vi "StreamEye_host_v6_32bit.vi"() -> ()   [LabVIEW 2018]
uses:
  CryoSubVIs/SubVIs/JS_Comm.llb/Comm_Paras.ctl
  CryoSubVIs/SubVIs/JS_Comm.llb/Comm_Method.ctl
  CryoSubVIs/SMC SubVIs/SMC_SubVIs.llb/SMC Paras.ctl
  CryoSubVIs/SMC SubVIs/SMC_SubVIs.llb/VENUSNr.ctl
  <vilib>/DAQmx/write.llb/DAQmx Write (Analog DBL 1Chan 1Samp).vi
  CryoSubVIs/SMC SubVIs/SMC_SubVIs.llb/glb_stop.vi
  CryoSubVIs/SMC SubVIs/SMC_SubVIs.llb/glb_pos.vi
  <vilib>/DAQmx/miscellaneous.llb/DAQmx Fill In Error Info.vi
  <vilib>/Utility/file.llb/Write Delimited Spreadsheet (I64).vi
  <vilib>/Utility/file.llb/Write Delimited Spreadsheet (DBL).vi
  <vilib>/DAQmx/create/channels.llb/DAQmx Create Channel (AO-Voltage-Basic).vi
  PicoHarpLibrary/ttrmode32_custom.llb/Global.vi
  PicoHarpLibrary/PHLib.dll
panel:
  in  "Start Sync":bool
  in  "Drift Comp BackStep":dbl caption="BackStep (µm)" min=-10000.0 max=10000.0 step=0.001
  in  "Compensate Int Time":dbl=1000.0 caption="Int. Time (s)" min=0.5 max=36000.0 step=0.5 format="%.1f"
  out "FiFo Overrun":bool
  out "T2 Photon Count":i32 caption="Sum Photon Count" format="%0#_6p"
  in  "T2 Segments":u32 caption="Segments (#)" min=1
  in  "Drift Comp Step":dbl caption="Step (µm)" min=-10000.0 max=10000.0 step=0.001
  in  "Drift Comp Range":dbl caption="+/- Range (µm)" min=-10000.0 max=10000.0 step=0.001
  in  "Drift Compensate Time":i32=1000 caption="Drift Period (s)" min=0 max=1000000 step=1
  in  "Start T2 Collect":bool
  out "TTTR ON":bool
  in  "Enable T2":bool
  in  "Compensate":bool
  in  "Acc. Threshold (cts)":i64=1000 min=-1000000000 max=1000000000 step=1
  in  "Integration Number (#)":i32=1000 min=1 max=36000 step=1
  in  "SyncOffset (ps)":i32=1000 min=0 max=1000000 step=1
  out "Histo Graph":cluster{"Array":dbl[], u32[]}(graph)
  in  "Start Histogram":bool
  in  "Start Cursors Pair XY Sca":bool
  in  "Wait Scan.":bool
  in  "G-asym":dbl
  out "Res. (ps)":i32 min=0 max=2000 step=1
  in  "Histo Time (s)":dbl=1000.0 min=0.5 max=36000.0 step=0.5 format="%.1f"
  out "PicoHarp error":bool
  in  "Signal source selection":T1(radio)
  in  "Binning":i32 min=0 max=7 step=1
  in  "Sync div":enum16{"1", "2", "4", "8"}(ring)
  in  "Apply PicoHarp Settings":bool
  in  "Ch1 Level (mV)":i32=50 min=0 max=800 step=10
  in  "Ch1 ZeroX (mV)":i32=10 min=0 max=20 step=1
  in  "Ch0 ZeroX (mV)":i32=10 min=0 max=20 step=1
  in  "Ch0 Level (mV)":i32=50 min=0 max=800 step=10
  in  "Init Picoharp":bool
  out "PicoHarp ON":bool
  out "Ch1 Rate":dbl caption="Ch1" format="%#_3p"
  out "Ch0 Rate":dbl caption="Ch0" format="%#_3p"
  in  "Start Cursor XY Sca":bool
  in  "G-Scalling (µm/V)":dbl
  in  "Filaname":string
  in  "Path":path
  out "time elapsed dummy":dbl caption="int."
  in  "Intensity mode selection":T2(radio)
  out "time elapsed":dbl caption="Time per step (s)"
  out "XYZ MegaArray Sca":i32[][][](array[numeric])
  out "Data available XW":bool
  in  "Save Data XW":bool
  in  "Save Data Gal":bool
  in  "Save Data Sca":bool
  out "Data available Sca":bool
  out "Data available Gal":bool
  in  "Steps Hyperspectral Sca":u32 caption="Steps Hyperspectral (#)"
  in  "Steps Hyperspectral Gal":u32 caption="Steps Hyperspectral (#)"
  out "busy":bool
  in  "Start Stream":bool
  in  "Misc Info/Variables":T3(tab)
  out "Yscale Gal":dbl[](array[numeric]) format="%.2f"
  out "Wscale Gal":dbl[](array[numeric]) format="%.2f"
  out "Wscale Sca":dbl[](array[numeric]) format="%.2f"
  out "XYZ MegaArray Gal":i32[][][](array[numeric])
  out "XW MegaArray":i32[][](array[numeric])
  out "Xscale hyper":dbl[](array[numeric]) format="%.2f"
  out "Yscale hyper":dbl[](array[numeric]) format="%.2f"
  out "Wscale hyper":dbl[](array[numeric]) format="%.2f"
  out "XY Array Sca":i32[][](array[numeric])
  out "XY Array Gal":i32[][](array[numeric])
  out "Xscale Sca":dbl[](array[numeric]) format="%.2f"
  out "Yscale Sca":dbl[](array[numeric]) format="%.2f"
  out "Xscale Gal":dbl[](array[numeric]) format="%.2f"
  out "Scanner error out":errorcluster
  out "Galvo error out X":errorcluster
  out "Galvo task out X":refnum<k21>
  out "Galvo error out Y":errorcluster
  out "Galvo task out Y":refnum<k21>
  in  "numPixels":u16
  out "time start":i32 caption="Time per step (s)"
  out "single spectrum?":bool
  out "error reader":errorcluster
  out "error writer":errorcluster
  out "writer endpoint":refnum<k21>
  out "reader endpoint":refnum<k21>
  in  "T2 Block Size":u16(ring) items=["Min"=1, "Small"=2, "Mid"=3, "Large"=4, "Max"=5]
  in  "Test Comp histo":bool
  in  "Autosave Histograms":bool
  out "PicoHarp handle":i32
  out "DLL Version (must be 3.0)":string caption="DLL Version"
  out "Initialization Status":string
  out "Calibration Status":string
  out "file error status":errorcluster
  in  "Start Cursors Pair XY Gal":bool
  in  "Start image Sca":bool
  in  "Start Hyperspectral Sca":bool
  in  "Start image Gal":bool
  in  "Start Hyperspectral Gal":bool
  in  "Start Cursor XY Gal":bool
  in  "Yoffset_Sca":dbl min=-10000.0 max=10000.0 step=0.001
  in  "Xoffset_Sca":dbl min=-10000.0 max=10000.0 step=0.001
  out "Xsteps_Sca":u32
  out "Ysteps_Sca":u32 caption="yRead"
  in  "Ydelay_Sca":dbl=0.001 min=0.0 max=300000.0 step=0.001
  in  "Ystep_Sca":dbl=0.001 min=0.001 max=200.0 step=0.001
  in  "Xstep_Sca":dbl=0.001 min=-1000.0 max=1000.0 step=0.001
  in  "Xdelay_Sca":dbl=0.1 min=0.0 max=360000.0 step=0.001
  in  "Yend_Sca":dbl min=-10000.0 max=10000.0 step=0.001
  in  "Ystart_Sca":dbl min=-10000.0 max=10000.0 step=0.001
  in  "Xend_Sca":dbl min=-10000.0 max=10000.0 step=0.001
  in  "Xstart_Sca":dbl min=-10000.0 max=10000.0 step=0.001
  out "Xread_Sca":dbl format="%#.3g"
  out "Yread_Sca":dbl caption="yRead" format="%#.3g"
  in  "Yset_Sca":dbl min=-5000.0 max=5000.0 step=0.001
  in  "Xset_Sca":dbl min=-10000.0 max=10000.0 step=0.001
  in  "Yoffset_Gal":dbl min=-100.0 max=100.0 step=0.001
  in  "Xoffset_Gal":dbl min=-100.0 max=100.0 step=0.001
  out "Xsteps_Gal":u32
  out "Ysteps_Gal":u32 caption="yRead"
  in  "Stop Measurement":bool
  out "Hosts Synchronized":bool
  in  "Synchronize Hosts":bool
  out "XYZ Graph Scanner":i32[][](graph)
  out "XYZ Graph Galvos":i32[][](graph)
  out "XYZ hyperspectral graph":i32[][](graph)
  out "Current Intensity":dbl format="%#_6p"
  out "Time Trace":dbl(graph)
  out "Spectrum Graph":T4(graph)
  in  "Go position Gal":bool
  in  "Ydelay_Gal":dbl=0.001 min=0.0 max=300000.0 step=0.001
  in  "Ystep_Gal":dbl=0.001 min=0.001 max=200.0 step=0.001
  in  "Xstep_Gal":dbl=0.001 min=-1000.0 max=1000.0 step=0.001
  in  "Xdelay_Gal":dbl=0.1 min=0.0 max=360000.0 step=0.001
  in  "Yend_Gal":dbl min=-100.0 max=100.0 step=0.001
  in  "Ystart_Gal":dbl min=-100.0 max=100.0 step=0.001
  in  "Xend_Gal":dbl min=-100.0 max=100.0 step=0.001
  in  "Xstart_Gal":dbl min=-100.0 max=100.0 step=0.001
  out "Xread_Gal":dbl format="%#.3g"
  out "Yread_Gal":dbl caption="yRead" format="%#.3g"
  in  "Yset_Gal":dbl min=-1000.0 max=1000.0 step=0.001
  in  "Xset_Gal":dbl min=-1000.0 max=1000.0 step=0.001
  out "Galvos ON":bool
  in  "Init Galvos":bool
  in  "Go position Sca":bool
  out "Scanner ON":bool
  in  "Init Scanner":bool
  in  "Exit":bool
  # "Signal Source"
  # "Stream Mode"
  # "Scanner"
  # "Galvos"
  # "X-axis"
  # "X-axis"
  # "Y-axis"
  # "Y-axis"
  # "Offset (µm)"
  # "Set (µm)"
  # "Readout"
  # "Start (µm)"
  # "End (µm)"
  # "Step (µm)"
  # "Intensity"
  # "Steps (#)"
  # "Delay (s)"
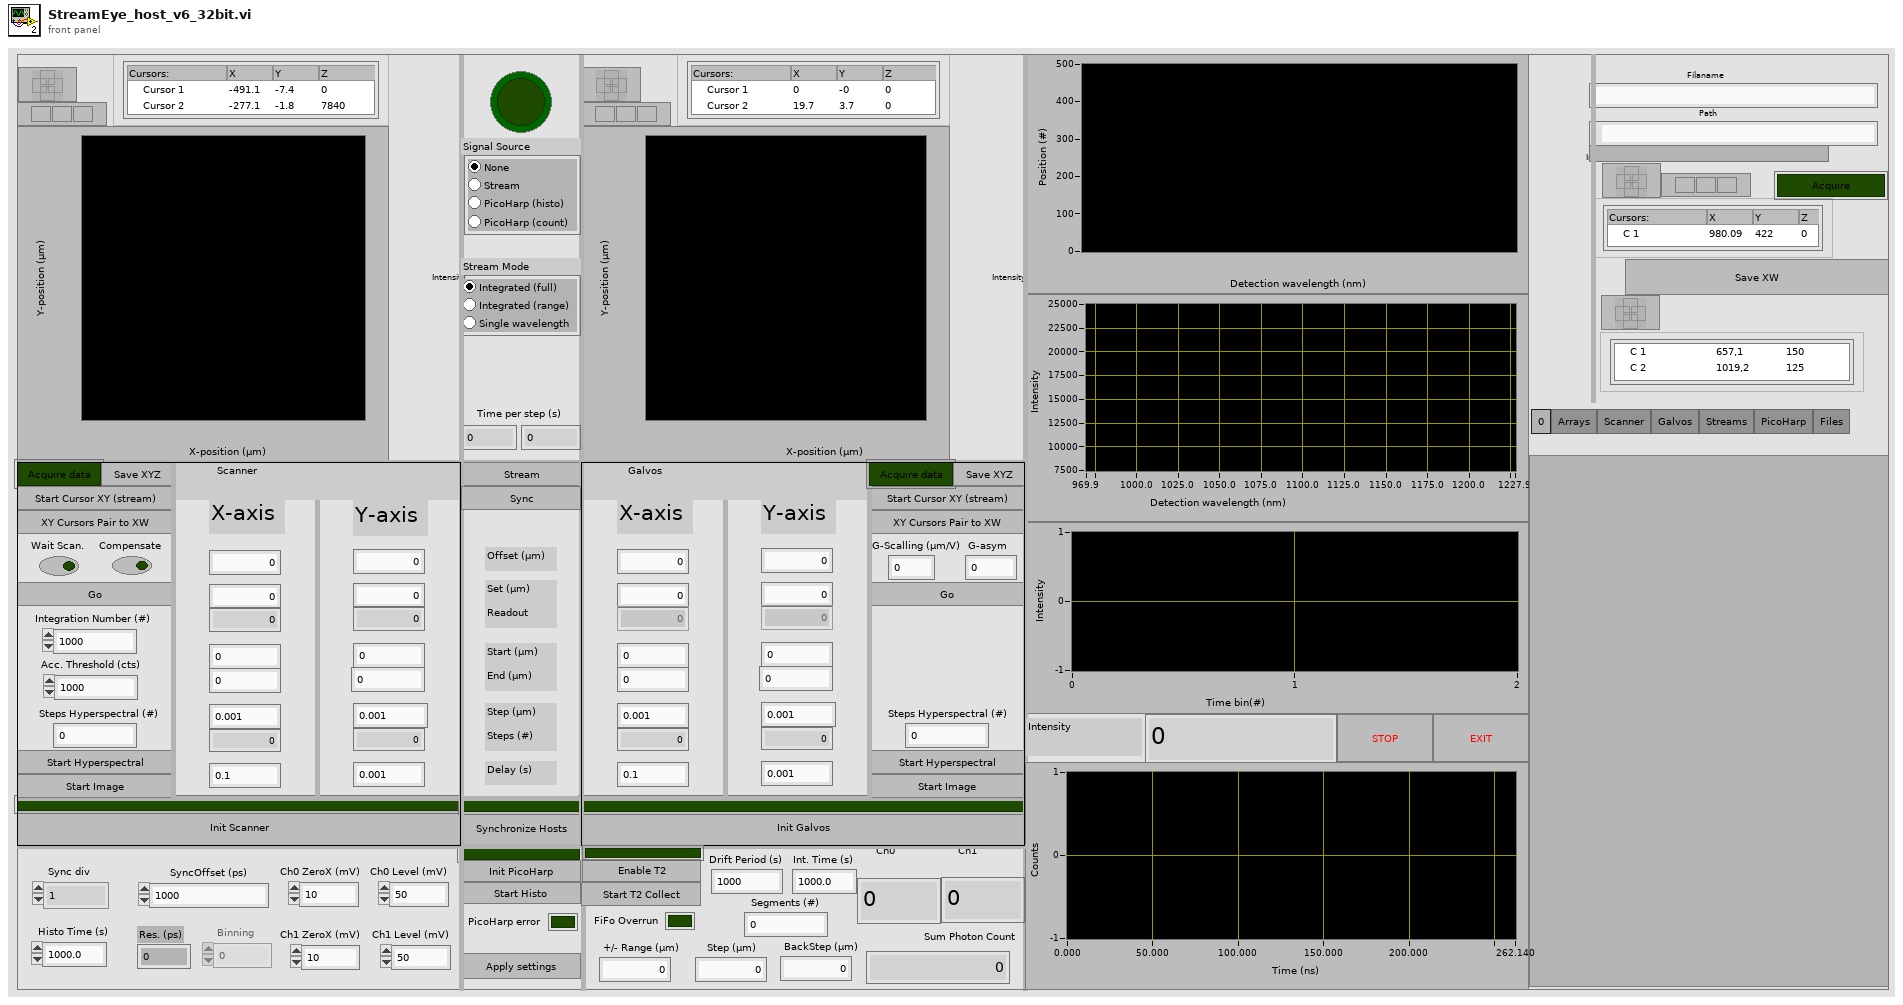
[diagram p1: front panel]
types:
  T1 = enum32{"Signal None", "Signal Stream", "Signal PicoHarp histro", "Signal PicoHarp count rate"}
  T2 = enum32{"Integrated (full)", "Integrated (range)", "Single wavelength"}
  T3 = enum32{"0", "Arrays", "Scanner", "Galvos", "Streams", "PicoHarp", "Files"}
  T4 = cluster{"Calibrated Array":dbl[], "Array F32":sgl[]}
  T5 = enum16{"big-endian, network order", "native, host order", "little-endian"}
  T6 = enum16{"open", "replace", "create", "open or create", "replace or create", "replace or create with confirmation"}
  T7 = typedef "SMC Paras.ctl" = cluster{"VENUS Language":T8, "Number of Axis":u8, "Controller Nr":u8, "Simulation":bool}
  T8 = typedef "VENUSNr.ctl" = enum16{"VENUS 2", "VENUS 1"}
  T9 = typedef "Comm_Paras.ctl" = cluster{"Comm Method":T10, "Com Port":i32, "Baud Rate":u32, "IP Address":string, "Remote Port":u16, "GPIB Address":string, "VISA Resource Name":refnum<visa-resource-name>, "Visa Baud Rate":u32, "Visa Serial":bool}
  T10 = typedef "Comm_Method.ctl" = enum16{"RS232", "TCPIP", "GPIB", "VISA"}
  T11 = typedef "LVCursorListTypeDef.ctl" = cluster{"Name":string, "Color":u32, "Style":u8, "Point Style":u8, "Name Visible":bool, "Allow Drag":bool, "Cursor Mode":u32, "Plot":i32, "Index":i32, "Position":cluster{"X":dbl, "Y":dbl}, "X Scale":u32, "Y Scale":u32, "Watch Plots":i32[], "Watch All Plots":bool, "Plot Area":i32, "Label Offset":cluster{"X":dbl, "Y":dbl}}[]
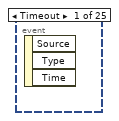
[diagram p2: hidden frame]
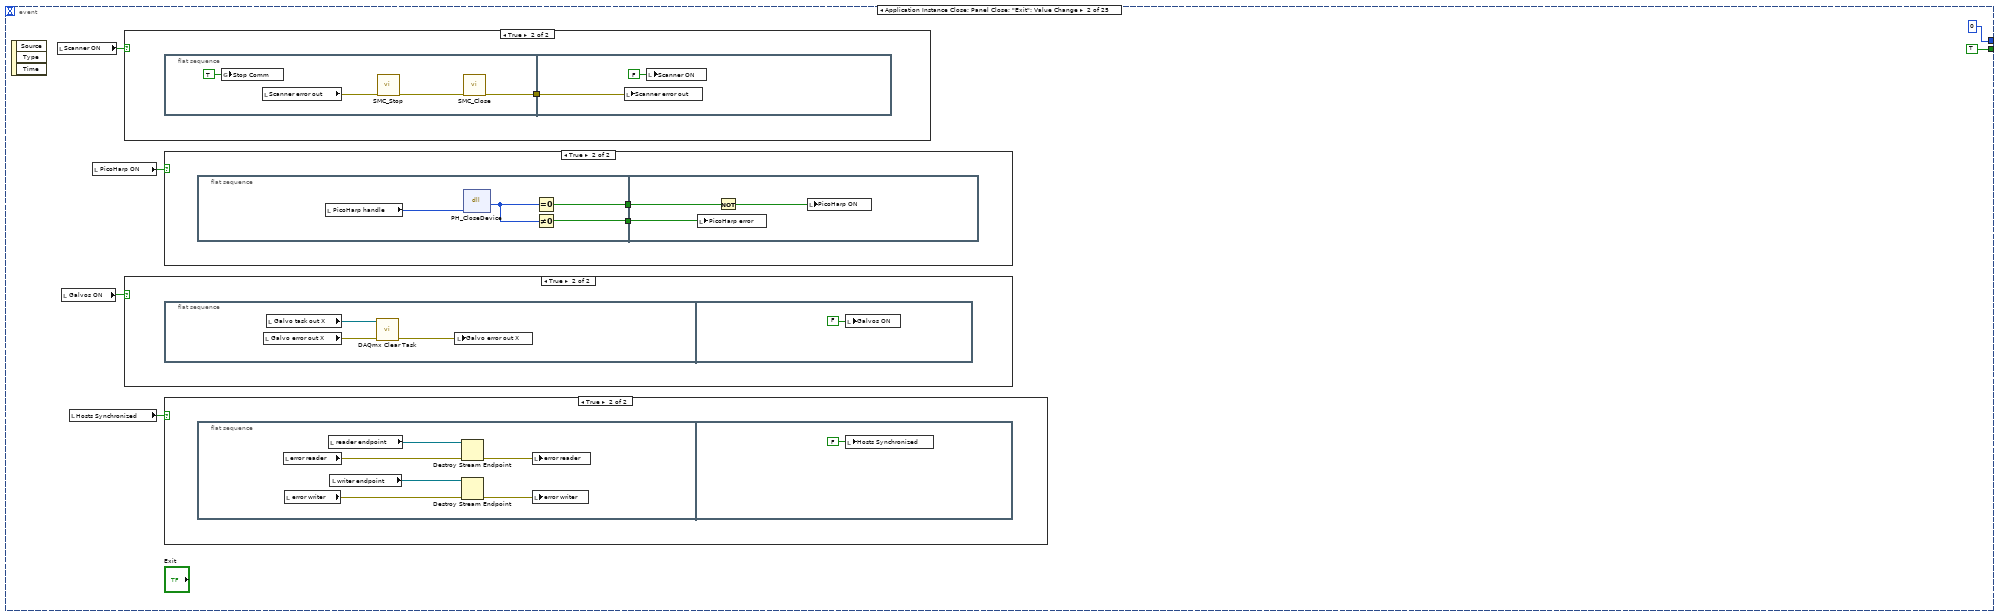
[diagram p3: hidden frame]
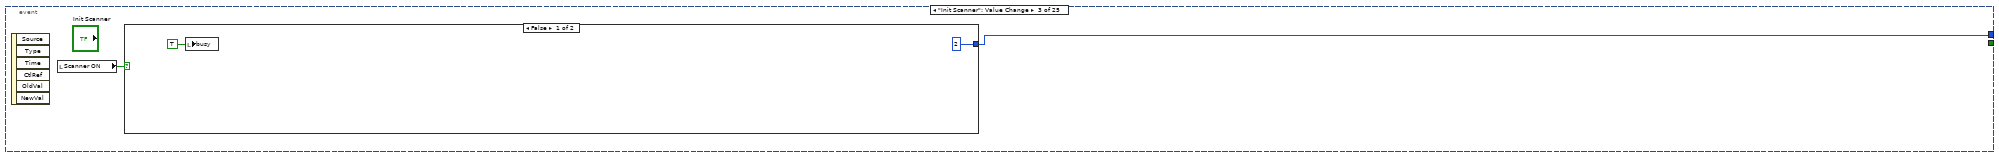
[diagram p8: hidden frame]
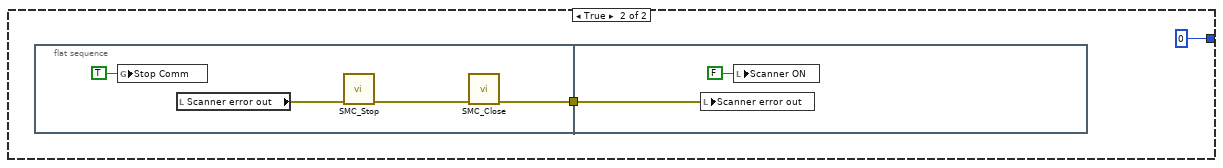
[diagram p9: hidden frame]
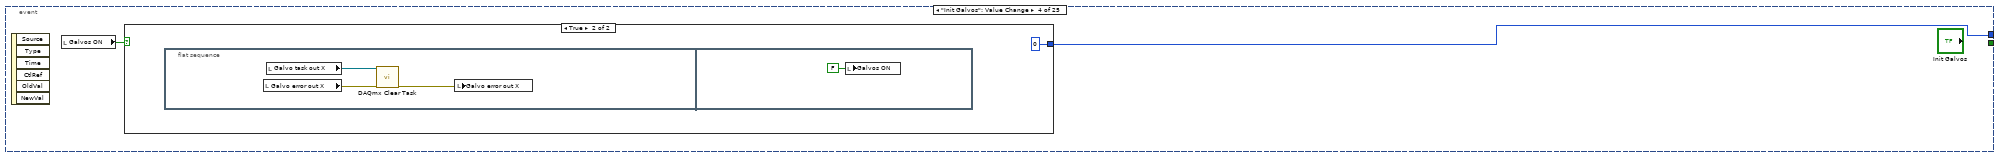
[diagram p10: hidden frame]
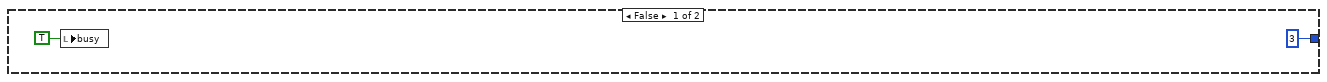
[diagram p11: hidden frame]
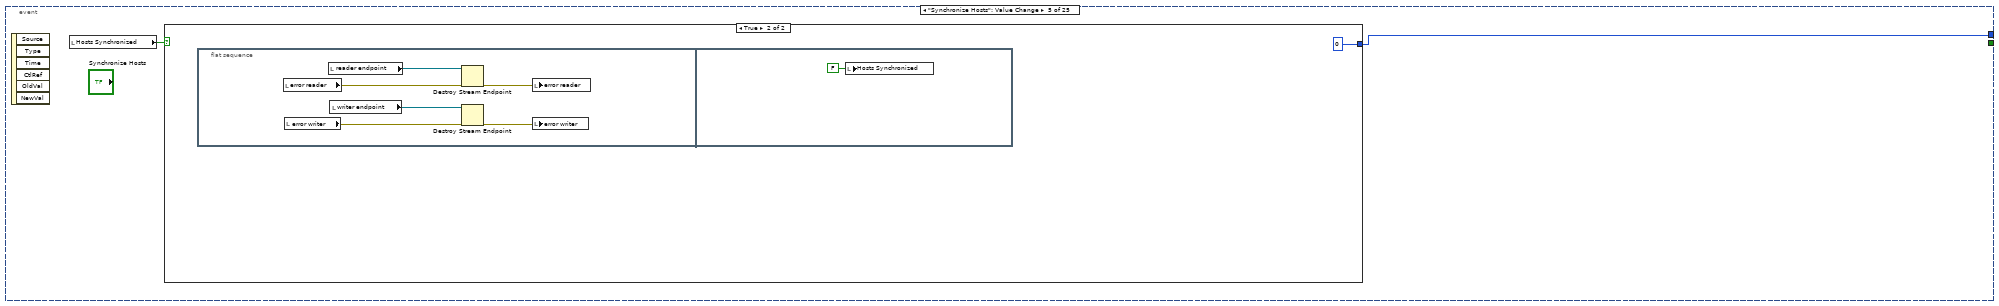
[diagram p12: hidden frame]
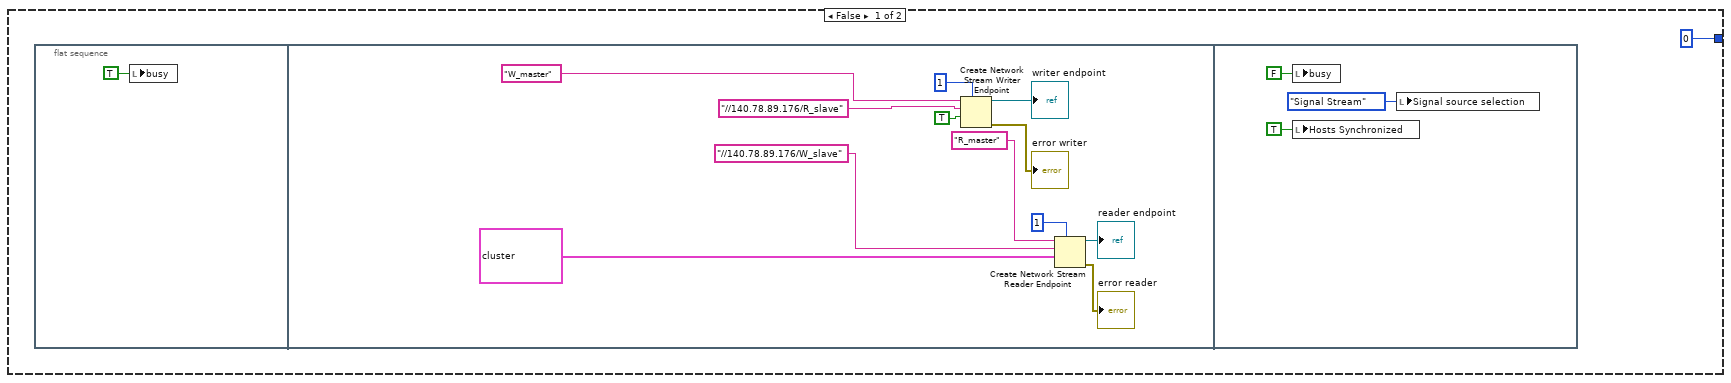
[diagram p13: hidden frame]
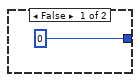
[diagram p14: hidden frame]
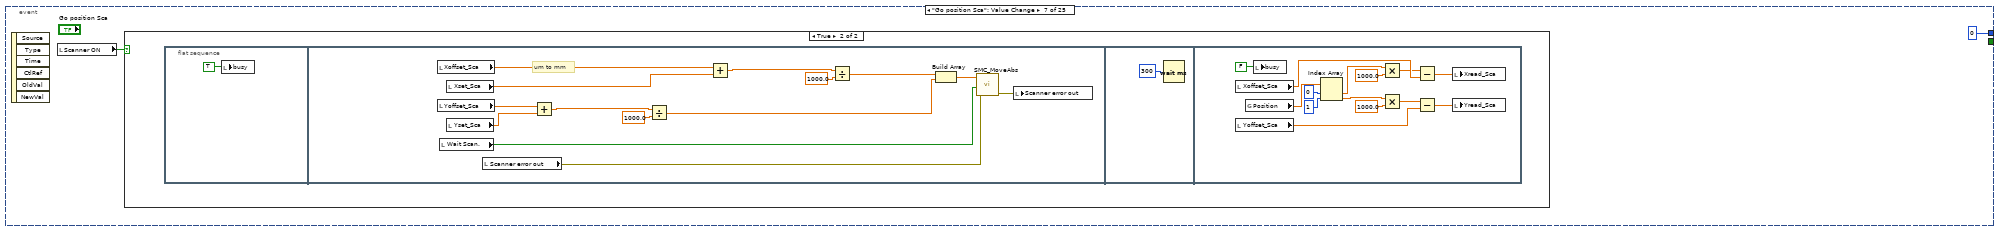
[diagram p15: hidden frame]
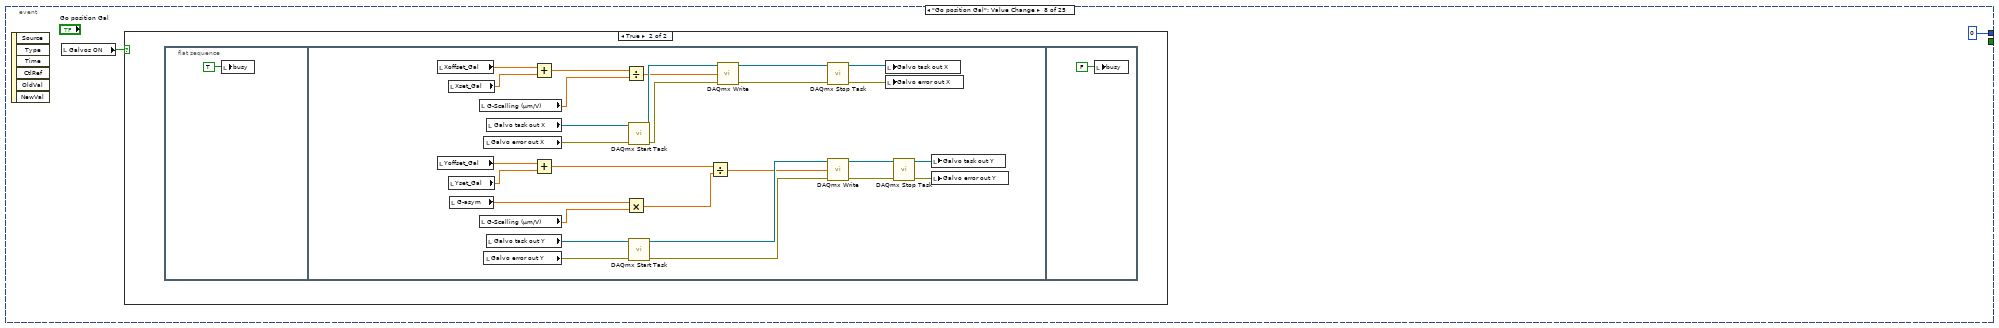
[diagram p17: hidden frame]
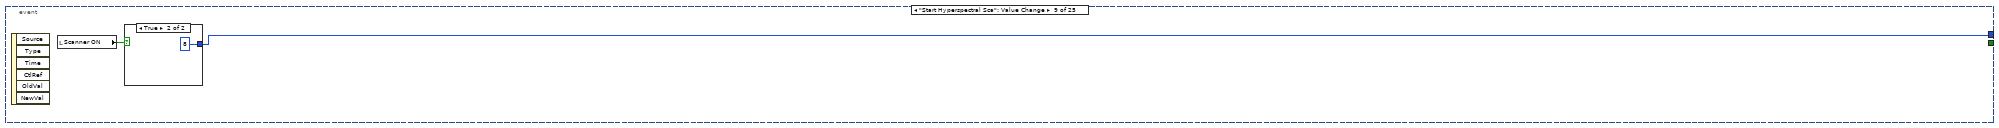
[diagram p19: hidden frame]
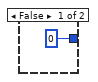
[diagram p20: hidden frame]
diagram:
  n1 = flat-sequence {
    frame #0 {
      w1 = u16 3 items=["Min"=1, "Small"=2, "Mid"=3, "Large"=4, "Max"=5] ("T2 Block Size")
      w22 = 1 ("dimension size")
      w21 = 1 ("dimension size")
      w19 = 1 ("dimension size")
      w20 = 1 ("dimension size")
      w2 = FALSE ("busy")
      n2 = Initialize Array(w22, w22, 1 ("dimension size")) -> (→"XY Array Sca":i32[][])
      n3 = Initialize Array(0, 1 ("dimension size"), 1 ("dimension size")) -> (→"XY Array Gal":i32[][])
      n4 = Initialize Array(w19, w19, 1 ("dimension size")) -> (→"XW MegaArray":i32[][])
      n5 = local write "Binning"(0 ("Range#")) -> ()
      n6 = local write "SyncOffset (ps)"(0 ("SyncOffset (ps)")) -> ()
      n7 = local write "Yoffset_Gal"(0.0 ("Yoffset_Gal")) -> ()
      n8 = local write "Histo Time (s)"(1.0 ("Histro Time (s)")) -> ()
      n9 = local write "Wait Scan."(TRUE ("Wait scanner?")) -> ()
      n10 = local write "Xoffset_Gal"(30.0 ("Xoffset_Gal")) -> ()
      n11 = local write "Ch1 ZeroX (mV)"(10 ("Ch1 ZeroX (mV)")) -> ()
      n12 = local write "G-Scalling (µm/V)"(30.0 ("Galvo Scalling (µm/V)")) -> ()
      n13 = local write "Ch0 ZeroX (mV)"(10 ("Ch0 ZeroX (mV)")) -> ()
      n14 = local write "Ch1 Level (mV)"(200 ("Ch1 Level (mV)")) -> ()
      n15 = local write "Ch0 Level (mV)"(200 ("Ch0 Level (mV)")) -> ()
      n16 = local write "G-asym"(1.45 ("G-asym")) -> ()
      n17 = local write "numPixels"(u16 1024 ("numPixels")) -> ()
      n18 = local write "numPixels"(u16 1024 ("numPixels")) -> ()
      n19 = local write "Sync div"(enum16{"1", "2", "4", "8"}."1" ("Syncdiv")) -> ()
      n20 = local write "T2 Block Size"(w1) -> ()
      n21 = call "subVI_RampGenerator.vi"("Number of Positions"=u16 1, "End  (um)"=10.0, "Start  (um)"=0.0) -> ("Array"=→"Xscale Sca" →"Xscale Gal" →"Yscale Gal" →"Yscale Sca" →"Wscale Gal" →"Wscale Sca" →"Xscale hyper" →"Yscale hyper" →"Wscale hyper":dbl[])  [unwired: 1 in]
      n22 = Initialize Array(w20, w20, 1 ("dimension size"), 1 ("dimension size")) -> (→"XYZ MegaArray Sca":i32[][][])
      n23 = Initialize Array(w21, w21, 1 ("dimension size"), 1 ("dimension size")) -> (→"XYZ MegaArray Gal":i32[][][])
      n24 = local write "Compensate"(w2) -> ()
      n25 = local write "Stop Measurement"(w2) -> ()
      "Scanner ON" <- w2
      "Galvos ON" <- w2
      "Hosts Synchronized" <- w2
      "busy" <- w2
      "Data available Gal" <- w2
      "Data available Sca" <- w2
      "single spectrum?" <- TRUE ("single spectrum?")
      "Data available XW" <- w2
      "PicoHarp ON" <- w2
      "PicoHarp error" <- w2
      "TTTR ON" <- w2
      "T2 Photon Count" <- u32 0 ("T2 Photon Count")
      "FiFo Overrun" <- w2
    }
    frame #1 {
      n26 = while {
        stop <- w42 stop-if-true
        n27 = flat-sequence {
          tunnel: [w45] -> w43
          tunnel: [w44] -> w42
          tunnel: w43 -> [w443]
          frame #0 {
            # "event catcher"
            n28 = event shown="[5] \"Start Stream\": Value Change" {
              selector: _ -> [_ _ _ _ _ _ _ _ _ _ _ _ _ _ _ _ _ _ _ _ _ _ _ _ _]
              dyn-events: _ -> [_ _ _ _ _ _ _ _ _ _ _ _ _ _ _ _ _ _ _ _ _ _ _ _ _]
              timeout: 250 -> [_ _ _ _ _ _ _ _ _ _ _ _ _ _ _ _ _ _ _ _ _ _ _ _ _]
              tunnel: [_ 0 w80 w93 w101 w133 0 0 w201 w205 w209 w213 w217 w221 _ _ _ w313 w318 _ w369 w372 w379 w383 w440] -> w45
              tunnel: [_ TRUE _ _ _ _ _ _ _ _ _ _ _ _ _ _ _ _ _ _ _ _ _ _ _] -> w44
              event Timeout {
                n29 = event-data() -> ()  [unwired: 1 in, 3 out]
              }
              event Application Instance Close; Panel Close; "Exit": Value Change {
                n30 = event-data() -> ()  [unwired: 1 in, 3 out]
                n31 = local read "Scanner ON"() -> (w49:bool)
                n32 = local read "Galvos ON"() -> (w48:bool)
                n33 = local read "Hosts Synchronized"() -> (w52:bool)
                n34 = local read "PicoHarp ON"() -> (w47:bool)
                n35 = case shown="True" w49 {
                  frame False {
                  }
                  frame True {
                    n36 = flat-sequence {
                      tunnel: [w70] -> w66
                      tunnel: w66 -> [w71]
                      frame #0 {
                        n37 = global write "glb_stop.vi" "Stop Comm"(TRUE ("Stop Comm")) -> ()
                        n38 = local read "Scanner error out"() -> (w67:errorcluster)
                        n39 = call "SMC_Stop.vi"("error in (no error)"=w67) -> ("error out"=w68:errorcluster)  [unwired: 10 in]
                        n40 = call "SMC_Close.vi"("error in (no error)"=w68) -> ("error out"=w70:errorcluster)  [unwired: 10 in]
                      }
                      frame #1 {
                        n41 = local write "Scanner error out"(w71) -> ()
                        n42 = local write "Scanner ON"(FALSE ("Scanner ON")) -> ()
                      }
                    }
                  }
                }
                n43 = case shown="True" w48 {
                  frame False {
                  }
                  frame True {
                    n44 = flat-sequence {
                      frame #0 {
                        n45 = local read "Galvo error out X"() -> (w63:errorcluster)
                        n46 = local read "Galvo task out X"() -> (w64:refnum<k21>)
                        n47 = call <vilib>:"DAQmx Clear Task.vi"("task in"=w64, "error in"=w63) -> ("error out"=w62:errorcluster)  [unwired: 13 in]
                        n48 = local write "Galvo error out X"(w62) -> ()
                      }
                      frame #1 {
                        n49 = local write "Galvos ON"(FALSE ("Galvos ON")) -> ()
                      }
                    }
                  }
                }
                n50 = case shown="True" w47 {
                  frame False {
                  }
                  frame True {
                    n51 = flat-sequence {
                      tunnel: [w56] -> w54
                      tunnel: [w55] -> w53
                      tunnel: w54 -> [w61]
                      tunnel: w53 -> [w59]
                      frame #0 {
                        n52 = local read "PicoHarp handle"() -> (w58:i32)
                        n53 = dll-call lib="F:/Users/Yuriy/Labview/JKU/StreamEye/StreamEye_master_v2_comp2015/PicoHarpLibrary/PHLib.dll" fn="PH_CloseDevice"("devidx"=w58) -> ("return type"=w57:i32)  [unwired: 4 in, 2 out]
                        n54 = Equal To 0?(x=w57) -> (x = 0?=w56:bool)
                        n55 = Not Equal To 0?(x=w57) -> (x != 0?=w55:bool)
                      }
                      frame #1 {
                        n56 = local write "PicoHarp error"(w59) -> ()
                        n57 = Not(x=w61) -> (.not. x?=w60:bool)
                        n58 = local write "PicoHarp ON"(w60) -> ()
                      }
                    }
                  }
                }
                n59 = case shown="True" w52 {
                  frame False {
                  }
                  frame True {
                    n60 = flat-sequence {
                      frame #0 {
                        n61 = local read "error reader"() -> (w78:errorcluster)
                        n62 = local read "error writer"() -> (w75:errorcluster)
                        n63 = local read "reader endpoint"() -> (w73:refnum<k21>)
                        n64 = local read "writer endpoint"() -> (w74:refnum<k21>)
                        n65 = Destroy Stream Endpoint(8:w78, 11:w73) -> (0:w77:errorcluster)
                        n66 = Destroy Stream Endpoint(8:w75, 11:w74) -> (0:w76:errorcluster)
                        n67 = local write "error reader"(w77) -> ()
                        n68 = local write "error writer"(w76) -> ()
                      }
                      frame #1 {
                        n69 = local write "Hosts Synchronized"(FALSE ("Hosts Synchronized")) -> ()
                      }
                    }
                  }
                }
              }
              event "Init Scanner": Value Change {
                n70 = event-data() -> ()  [unwired: 1 in, 6 out]
                n71 = local read "Scanner ON"() -> (w81:bool)
                n72 = case shown="False" w81 {
                  tunnel: [2 0] -> w80
                  frame False {
                    n73 = local write "busy"(TRUE ("busy")) -> ()
                  }
                  frame True {
                    n74 = flat-sequence {
                      tunnel: [w89] -> w84
                      tunnel: w84 -> [w90]
                      frame #0 {
                        n75 = global write "glb_stop.vi" "Stop Comm"(TRUE ("Stop Comm")) -> ()
                        n76 = local read "Scanner error out"() -> (w86:errorcluster)
                        n77 = call "SMC_Stop.vi"("error in (no error)"=w86) -> ("error out"=w87:errorcluster)  [unwired: 10 in]
                        n78 = call "SMC_Close.vi"("error in (no error)"=w87) -> ("error out"=w89:errorcluster)  [unwired: 10 in]
                      }
                      frame #1 {
                        n79 = local write "Scanner error out"(w90) -> ()
                        n80 = local write "Scanner ON"(FALSE ("Scanner ON")) -> ()
                      }
                    }
                  }
                }
              }
              event "Init Galvos": Value Change {
                n81 = event-data() -> ()  [unwired: 1 in, 6 out]
                n82 = local read "Galvos ON"() -> (w92:bool)
                n83 = case shown="True" w92 {
                  tunnel: [3 0] -> w93
                  frame False {
                    n84 = local write "busy"(TRUE ("busy")) -> ()
                  }
                  frame True {
                    n85 = flat-sequence {
                      frame #0 {
                        n86 = local read "Galvo error out X"() -> (w98:errorcluster)
                        n87 = local read "Galvo task out X"() -> (w99:refnum<k21>)
                        n88 = call <vilib>:"DAQmx Clear Task.vi"("task in"=w99, "error in"=w98) -> ("error out"=w97:errorcluster)  [unwired: 13 in]
                        n89 = local write "Galvo error out X"(w97) -> ()
                      }
                      frame #1 {
                        n90 = local write "Galvos ON"(FALSE ("Galvos ON")) -> ()
                      }
                    }
                  }
                }
              }
              event "Synchronize Hosts": Value Change {
                n91 = event-data() -> ()  [unwired: 1 in, 6 out]
                n92 = local read "Hosts Synchronized"() -> (w102:bool)
                n93 = case shown="True" w102 {
                  tunnel: [0 0] -> w101
                  frame False {
                    n94 = flat-sequence {
                      frame #0 {
                        n95 = local write "busy"(TRUE ("busy")) -> ()
                      }
                      frame #1 {
                        n96 = Create Network Stream Writer Endpoint(7:1 ("writer buffer size"), 9:TRUE, 10:"//140.78.89.176/R_slave" ("writer url"), 11:"W_master" ("reader name")) -> (0:→"error writer":errorcluster, 3:→"writer endpoint":refnum<k21>)  [unwired: 3 in]
                        n97 = Create Network Stream Reader Endpoint(7:1 ("reader buffer size"), 9:cluster{dbl[], dbl[]} {array[512 elements], array[512 elements]} ("XY Graph OMA V"), 10:"//140.78.89.176/W_slave" ("writer url"), 11:"R_master" ("reader name")) -> (0:→"error reader":errorcluster, 3:→"reader endpoint":refnum<k21>)  [unwired: 3 in]
                      }
                      frame #2 {
                        n98 = local write "busy"(FALSE ("busy")) -> ()
                        n99 = local write "Hosts Synchronized"(TRUE ("Hosts Synchronized")) -> ()
                        n100 = local write "Signal source selection"(T1."Signal Stream" ("Signal source selection")) -> ()
                      }
                    }
                  }
                  frame True {
                    n101 = flat-sequence {
                      frame #0 {
                        n102 = local read "error reader"() -> (w126:errorcluster)
                        n103 = local read "error writer"() -> (w123:errorcluster)
                        n104 = local read "reader endpoint"() -> (w121:refnum<k21>)
                        n105 = local read "writer endpoint"() -> (w122:refnum<k21>)
                        n106 = Destroy Stream Endpoint(8:w126, 11:w121) -> (0:w125:errorcluster)
                        n107 = Destroy Stream Endpoint(8:w123, 11:w122) -> (0:w124:errorcluster)
                        n108 = local write "error reader"(w125) -> ()
                        n109 = local write "error writer"(w124) -> ()
                      }
                      frame #1 {
                        n110 = local write "Hosts Synchronized"(FALSE ("Hosts Synchronized")) -> ()
                      }
                    }
                  }
                }
              }
              event "Start Stream": Value Change {
                n111 = event-data() -> ()  [unwired: 1 in, 6 out]
                n112 = local read "Hosts Synchronized"() -> (w131:bool)
                n113 = local read "Signal source selection"() -> (w130:T1)
                n114 = Equal?(x=w130, y=T1."Signal Stream" ("Signal source selection")) -> (x = y?=w128:bool)
                n115 = And(x=w131, y=w128) -> (x .and. y?=w132:bool)
                n116 = case shown="True" w132 {
                  tunnel: [0 5] -> w133
                  frame False {
                  }
                  frame True {
                  }
                }
              }
              event "Go position Sca": Value Change {
                n117 = event-data() -> ()  [unwired: 1 in, 6 out]
                n118 = local read "Scanner ON"() -> (w136:bool)
                n119 = case shown="True" w136 {
                  frame False {
                  }
                  frame True {
                    n120 = flat-sequence {
                      frame #0 {
                        n121 = local write "busy"(TRUE ("busy")) -> ()
                      }
                      frame #1 {
                        # "um to mm"
                        n122 = local read "Xoffset_Sca"() -> (w145:dbl)
                        n123 = local read "Yoffset_Sca"() -> (w147:dbl)
                        n124 = local read "Wait Scan."() -> (w139:bool)
                        n125 = local read "Xset_Sca"() -> (w144:dbl)
                        n126 = local read "Yset_Sca"() -> (w146:dbl)
                        n127 = local read "Scanner error out"() -> (w152:errorcluster)
                        n128 = Add(x=w147, y=w146) -> (x+y=w149:dbl)
                        n129 = Divide(x=w149, y=1000.0) -> (x/y=w142:dbl)
                        n130 = Add(x=w145, y=w144) -> (x+y=w151:dbl)
                        n131 = Divide(x=w151, y=1000.0) -> (x/y=w143:dbl)
                        n132 = Build Array(w143, w142) -> (w141:dbl[])
                        n133 = call "SMC_MoveAbs.vi"("error in (no error)"=w152, "WaitUntilReady"=w139, "Input Array"=w141) -> ("error out"=w140:errorcluster)  [unwired: 8 in]
                        n134 = local write "Scanner error out"(w140) -> ()
                      }
                      frame #2 {
                        n135 = Wait (ms)(milliseconds to wait=u32 300) -> ()  [unwired: 1 out]
                      }
                      frame #3 {
                        n136 = local read "Xoffset_Sca"() -> (w160:dbl)
                        n137 = local read "Yoffset_Sca"() -> (w163:dbl)
                        n138 = global read "glb_pos.vi" "Position"() -> (w158:dbl[])
                        n139 = local write "busy"(FALSE ("busy")) -> ()
                        n140 = Index Array(array=w158, index #1=0 ("index"), index #2=1 ("index")) -> (element #1=w162:dbl, element #2=w166:dbl)
                        n141 = Multiply(x=w162, y=1000.0) -> (x*y=w159:dbl)
                        n142 = Multiply(x=w166, y=1000.0) -> (x*y=w164:dbl)
                        n143 = Subtract(x=w159, y=w160) -> (x-y=w161:dbl)
                        n144 = Subtract(x=w164, y=w163) -> (x-y=w165:dbl)
                        n145 = local write "Xread_Sca"(w161) -> ()
                        n146 = local write "Yread_Sca"(w165) -> ()
                      }
                    }
                  }
                }
              }
              event "Go position Gal": Value Change {
                n147 = event-data() -> ()  [unwired: 1 in, 6 out]
                n148 = local read "Galvos ON"() -> (w168:bool)
                n149 = case shown="True" w168 {
                  frame False {
                  }
                  frame True {
                    n150 = flat-sequence {
                      frame #0 {
                        n151 = local write "busy"(TRUE ("busy")) -> ()
                      }
                      frame #1 {
                        n152 = local read "Xoffset_Gal"() -> (w198:dbl)
                        n153 = local read "Yoffset_Gal"() -> (w196:dbl)
                        n154 = local read "Xset_Gal"() -> (w197:dbl)
                        n155 = local read "Yset_Gal"() -> (w195:dbl)
                        n156 = local read "G-asym"() -> (w173:dbl)
                        n157 = local read "G-Scalling (µm/V)"() -> (w177:dbl)
                        n158 = local read "G-Scalling (µm/V)"() -> (w172:dbl)
                        n159 = local read "Galvo error out X"() -> (w187:errorcluster)
                        n160 = local read "Galvo error out Y"() -> (w179:errorcluster)
                        n161 = local read "Galvo task out X"() -> (w188:refnum<k21>)
                        n162 = local read "Galvo task out Y"() -> (w180:refnum<k21>)
                        n163 = Add(x=w198, y=w197) -> (x+y=w178:dbl)
                        n164 = Add(x=w196, y=w195) -> (x+y=w175:dbl)
                        n165 = Divide(x=w178, y=w177) -> (x/y=w176:dbl)
                        n166 = Multiply(x=w173, y=w172) -> (x*y=w171:dbl)
                        n167 = call <vilib>:"DAQmx Start Task.vi"("task/channels in"=w188, "error in"=w187) -> ("task out"=w192:refnum<k21>, "error out"=w189:errorcluster)  [unwired: 12 in]
                        n168 = call <vilib>:"DAQmx Start Task.vi"("task/channels in"=w180, "error in"=w179) -> ("task out"=w184:refnum<k21>, "error out"=w181:errorcluster)  [unwired: 12 in]
                        n169 = Divide(x=w175, y=w171) -> (x/y=w174:dbl)
                        n170 = call-poly <vilib>:"DAQmx Write.vi"("task/channels in"=w192, "data"=w176, "error in"=w189) -> ("task out"=w191:refnum<k21>, "error out"=w190:errorcluster)  [unwired: 10 in, 1 out]
                        n171 = call <vilib>:"DAQmx Stop Task.vi"("task/channels in"=w191, "error in"=w190) -> ("task out"=w193:refnum<k21>, "error out"=w194:errorcluster)  [unwired: 12 in]
                        n172 = call-poly <vilib>:"DAQmx Write.vi"("task/channels in"=w184, "data"=w174, "error in"=w181) -> ("task out"=w183:refnum<k21>, "error out"=w182:errorcluster)  [unwired: 10 in, 1 out]
                        n173 = local write "Galvo task out X"(w193) -> ()
                        n174 = local write "Galvo error out X"(w194) -> ()
                        n175 = call <vilib>:"DAQmx Stop Task.vi"("task/channels in"=w183, "error in"=w182) -> ("task out"=w185:refnum<k21>, "error out"=w186:errorcluster)  [unwired: 12 in]
                        n176 = local write "Galvo task out Y"(w185) -> ()
                        n177 = local write "Galvo error out Y"(w186) -> ()
                      }
                      frame #2 {
                        n178 = local write "busy"(FALSE ("busy")) -> ()
                      }
                    }
                  }
                }
              }
              event "Start Hyperspectral Sca": Value Change {
                n179 = event-data() -> ()  [unwired: 1 in, 6 out]
                n180 = local read "Scanner ON"() -> (w200:bool)
                n181 = case shown="True" w200 {
                  tunnel: [0 8] -> w201
                  frame False {
                  }
                  frame True {
                  }
                }
              }
              event "Start image Sca": Value Change {
                n182 = event-data() -> ()  [unwired: 1 in, 6 out]
                n183 = local read "Scanner ON"() -> (w204:bool)
                n184 = case shown="True" w204 {
                  tunnel: [0 9] -> w205
                  frame False {
                  }
                  frame True {
                  }
                }
              }
              event "Start Hyperspectral Gal": Value Change {
                n185 = event-data() -> ()  [unwired: 1 in, 6 out]
                n186 = local read "Galvos ON"() -> (w208:bool)
                n187 = case shown="True" w208 {
                  tunnel: [0 10] -> w209
                  frame False {
                  }
                  frame True {
                  }
                }
              }
              event "Start image Gal": Value Change {
                n188 = event-data() -> ()  [unwired: 1 in, 6 out]
                n189 = local read "Galvos ON"() -> (w212:bool)
                n190 = case shown="True" w212 {
                  tunnel: [0 11] -> w213
                  frame False {
                  }
                  frame True {
                  }
                }
              }
              event "Start Cursor XY Gal": Value Change {
                n191 = event-data() -> ()  [unwired: 1 in, 6 out]
                n192 = local read "Galvos ON"() -> (w216:bool)
                n193 = case shown="True" w216 {
                  tunnel: [0 12] -> w217
                  frame False {
                  }
                  frame True {
                  }
                }
              }
              event "Start Cursors Pair XY Gal": Value Change {
                n194 = event-data() -> ()  [unwired: 1 in, 6 out]
                n195 = local read "Data available Gal"() -> (w220:bool)
                n196 = case shown="True" w220 {
                  tunnel: [0 13] -> w221
                  frame False {
                  }
                  frame True {
                  }
                }
              }
              event "Save Data Sca": Value Change {
                n197 = event-data() -> ()  [unwired: 1 in, 6 out]
                n198 = local read "Data available Sca"() -> (w224:bool)
                n199 = case shown="True" w224 {
                  frame False {
                  }
                  frame True {
                    w225 = TRUE ("transpose? (F)")
                    # "scales in absolute values (no offset)"
                    n200 = local read "Path"() -> (w231:path)
                    n201 = local read "XY Array Sca"() -> (w244:i32[][])
                    n202 = local read "Wscale Sca"() -> (w255:dbl[])
                    n203 = local read "Yscale Sca"() -> (w256:dbl[])
                    n204 = local read "Xscale Sca"() -> (w257:dbl[])
                    n205 = local read "Filaname"() -> (w237:string)
                    n206 = local read "XYZ MegaArray Sca"() -> (w258:i32[][][])
                    n207 = Concatenate Strings(w237, "XYW_sca.dat") -> (w235:string)
                    n208 = Concatenate Strings(w237, "Wscale_sca.dat") -> (w232:string)
                    n209 = Concatenate Strings(w237, "Yscale_sca.dat") -> (w234:string)
                    n210 = Concatenate Strings(w237, "XY_sca.dat") -> (w236:string)
                    n211 = Concatenate Strings(w237, "Xscale_sca.dat") -> (w233:string)
                    n212 = Build Path(base path=w231, name or relative path=w235) -> (appended path=w226:path)
                    n213 = Build Path(base path=w231, name or relative path=w232) -> (appended path=w228:path)
                    n214 = Build Path(base path=w231, name or relative path=w234) -> (appended path=w230:path)
                    n215 = Build Path(base path=w231, name or relative path=w236) -> (appended path=w227:path)
                    n216 = Build Path(base path=w231, name or relative path=w233) -> (appended path=w229:path)
                    n217 = Open/Create/Replace File(file path (use dialog)=w226, operation (0:open)=T6."replace or create", access (0:read/write)=enum16{"read/write", "read-only", "write-only"}."read/write") -> (refnum out=w254:refnum<file>, error out=w253:errorcluster)  [unwired: 3 in, 1 out]
                    n218 = call-poly <vilib>:"Write Delimited Spreadsheet.vi"("file path (dialog if empty)"=w228, "1D data"=w255, "append to file? (new file:F)"=FALSE, "transpose? (no:F)"=w225) -> ()  [unwired: 10 in, 2 out]
                    n219 = call-poly <vilib>:"Write Delimited Spreadsheet.vi"("file path (dialog if empty)"=w230, "1D data"=w256, "append to file? (new file:F)"=FALSE, "transpose? (no:F)"=w225) -> ()  [unwired: 10 in, 2 out]
                    n220 = call-poly <vilib>:"Write Delimited Spreadsheet.vi"("file path (dialog if empty)"=w227, "2D data"=w244, "append to file? (new file:F)"=FALSE, "transpose? (no:F)"=w225) -> ()  [unwired: 10 in, 2 out]
                    n221 = call-poly <vilib>:"Write Delimited Spreadsheet.vi"("file path (dialog if empty)"=w229, "1D data"=w257, "append to file? (new file:F)"=FALSE, "transpose? (no:F)"=w225) -> ()  [unwired: 10 in, 2 out]
                    n222 = Write to Binary File(file (use dialog)=w254, data=w258, error in=w253, 9:T5."little-endian" ("byte order (0:big-endian, network order)")) -> (refnum out=w252:refnum<file>, error out=w251:errorcluster)  [unwired: 2 in, 1 out]
                    n223 = Close File(refnum=w252, error in=w251) -> ()  [unwired: 2 out]
                  }
                }
              }
              event "Save Data Gal": Value Change {
                n224 = event-data() -> ()  [unwired: 1 in, 6 out]
                n225 = local read "Data available Gal"() -> (w259:bool)
                n226 = case shown="True" w259 {
                  frame False {
                  }
                  frame True {
                    w260 = TRUE ("transpose? (F)")
                    # "scales in absolute values (no offset)"
                    n227 = local read "Path"() -> (w266:path)
                    n228 = local read "XY Array Gal"() -> (w279:i32[][])
                    n229 = local read "Wscale Gal"() -> (w290:dbl[])
                    n230 = local read "Yscale Gal"() -> (w291:dbl[])
                    n231 = local read "Xscale Gal"() -> (w292:dbl[])
                    n232 = local read "Filaname"() -> (w272:string)
                    n233 = local read "XYZ MegaArray Gal"() -> (w293:i32[][][])
                    n234 = Concatenate Strings(w272, "Yscale_gal.dat") -> (w269:string)
                    n235 = Concatenate Strings(w272, "XYW_gal.dat") -> (w270:string)
                    n236 = Concatenate Strings(w272, "Xscale_gal.dat") -> (w268:string)
                    n237 = Concatenate Strings(w272, "Wscale_gal.dat") -> (w267:string)
                    n238 = Concatenate Strings(w272, "XY_gal.dat") -> (w271:string)
                    n239 = Build Path(base path=w266, name or relative path=w270) -> (appended path=w261:path)
                    n240 = Build Path(base path=w266, name or relative path=w268) -> (appended path=w264:path)
                    n241 = Build Path(base path=w266, name or relative path=w267) -> (appended path=w263:path)
                    n242 = Build Path(base path=w266, name or relative path=w271) -> (appended path=w262:path)
                    n243 = Open/Create/Replace File(file path (use dialog)=w261, operation (0:open)=T6."replace or create", access (0:read/write)=enum16{"read/write", "read-only", "write-only"}."read/write") -> (refnum out=w289:refnum<file>, error out=w288:errorcluster)  [unwired: 3 in, 1 out]
                    n244 = call-poly <vilib>:"Write Delimited Spreadsheet.vi"("file path (dialog if empty)"=w264, "1D data"=w292, "append to file? (new file:F)"=FALSE, "transpose? (no:F)"=w260) -> ()  [unwired: 10 in, 2 out]
                    n245 = call-poly <vilib>:"Write Delimited Spreadsheet.vi"("file path (dialog if empty)"=w263, "1D data"=w290, "append to file? (new file:F)"=FALSE, "transpose? (no:F)"=w260) -> ()  [unwired: 10 in, 2 out]
                    n246 = call-poly <vilib>:"Write Delimited Spreadsheet.vi"("file path (dialog if empty)"=w262, "2D data"=w279, "append to file? (new file:F)"=FALSE, "transpose? (no:F)"=w260) -> ()  [unwired: 10 in, 2 out]
                    n247 = Write to Binary File(file (use dialog)=w289, data=w293, error in=w288, 9:T5."little-endian" ("byte order (0:big-endian, network order)")) -> (refnum out=w287:refnum<file>, error out=w286:errorcluster)  [unwired: 2 in, 1 out]
                    n248 = Close File(refnum=w287, error in=w286) -> ()  [unwired: 2 out]
                    n249 = Build Path(base path=w266, name or relative path=w269) -> (appended path=w265:path)
                    n250 = call-poly <vilib>:"Write Delimited Spreadsheet.vi"("file path (dialog if empty)"=w265, "1D data"=w291, "append to file? (new file:F)"=FALSE, "transpose? (no:F)"=w260) -> ()  [unwired: 10 in, 2 out]
                  }
                }
              }
              event "Save Data XW": Value Change {
                n251 = event-data() -> ()  [unwired: 1 in, 6 out]
                n252 = local read "Data available XW"() -> (w294:bool)
                n253 = case shown="True" w294 {
                  frame False {
                  }
                  frame True {
                    w295 = TRUE ("transpose? (F)")
                    # "scales in absolute values (no offset)"
                    n254 = local read "Path"() -> (w299:path)
                    n255 = local read "Xscale hyper"() -> (w312:dbl[])
                    n256 = local read "Filaname"() -> (w303:string)
                    n257 = local read "XW MegaArray"() -> (w308:i32[][])
                    n258 = local read "Wscale hyper"() -> (w311:dbl[])
                    n259 = Concatenate Strings(w303, "XW_hyper.dat") -> (w302:string)
                    n260 = Concatenate Strings(w303, "Xscale_hyper.dat") -> (w301:string)
                    n261 = Build Path(base path=w299, name or relative path=w302) -> (appended path=w296:path)
                    n262 = Concatenate Strings(w303, "Wscale_hyper.dat") -> (w300:string)
                    n263 = Build Path(base path=w299, name or relative path=w300) -> (appended path=w297:path)
                    n264 = call-poly <vilib>:"Write Delimited Spreadsheet.vi"("file path (dialog if empty)"=w296, "2D data"=w308, "append to file? (new file:F)"=FALSE, "transpose? (no:F)"=w295) -> ()  [unwired: 10 in, 2 out]
                    n265 = call-poly <vilib>:"Write Delimited Spreadsheet.vi"("file path (dialog if empty)"=w297, "1D data"=w311, "append to file? (new file:F)"=FALSE, "transpose? (no:F)"=w295) -> ()  [unwired: 10 in, 2 out]
                    n266 = Build Path(base path=w299, name or relative path=w301) -> (appended path=w298:path)
                    n267 = call-poly <vilib>:"Write Delimited Spreadsheet.vi"("file path (dialog if empty)"=w298, "1D data"=w312, "append to file? (new file:F)"=FALSE, "transpose? (no:F)"=w295) -> ()  [unwired: 10 in, 2 out]
                  }
                }
              }
              event "Start Cursor XY Sca": Value Change {
                n268 = event-data() -> ()  [unwired: 1 in, 6 out]
                n269 = local read "Scanner ON"() -> (w314:bool)
                n270 = case shown="True" w314 {
                  tunnel: [0 17] -> w313
                  frame False {
                  }
                  frame True {
                  }
                }
              }
              event "Init Picoharp": Value Change {
                n271 = event-data() -> ()  [unwired: 1 in, 6 out]
                n272 = local read "PicoHarp ON"() -> (w317:bool)
                n273 = case shown="False" w317 {
                  tunnel: [18 0] -> w318
                  frame False {
                    n274 = flat-sequence {
                      tunnel: [w326] -> w319
                      tunnel: w319 -> [w335]
                      frame #0 {
                        n275 = local write "busy"(TRUE ("busy")) -> ()
                      }
                      frame #1 {
                        n276 = call "Initialization.vi"("Mode"=0) -> ("Deviceindex"=w329:i32, "Initialization Status"=w325:string, "DLL Version"=w324:string, "Initialisation Error"=w328:bool)  [unwired: 1 in]
                        n277 = local write "PicoHarp handle"(w329) -> ()
                        n278 = local write "Initialization Status"(w325) -> ()
                        n279 = case shown="False" w328 {
                          selector: w328 -> [_ w333]
                          tunnel: [w332 "Not calibrated"] -> w323
                          tunnel: [w331 w333] -> w327
                          tunnel: w329 -> [w330 _]
                          frame False {
                            n280 = call "Calibrate.vi"("Deviceindex"=w330) -> ("Calib Error"=w331:bool, "Status"=w332:string)  [unwired: 1 in]
                          }
                          frame True {
                          }
                        }
                        n281 = local write "DLL Version (must be 3.0)"(w324) -> ()
                        n282 = local write "Calibration Status"(w323) -> ()
                        n283 = local write "PicoHarp error"(w327) -> ()
                        n284 = Not(x=w327) -> (.not. x?=w326:bool)
                        n285 = local write "PicoHarp ON"(w326) -> ()
                      }
                      frame #2 {
                        n286 = case shown="True" w335 {
                          frame False {
                          }
                          frame True {
                            n287 = local write "Signal source selection"(T1."Signal PicoHarp count rate" ("Signal source selection")) -> ()
                          }
                        }
                        n288 = local write "busy"(FALSE ("busy")) -> ()
                      }
                    }
                  }
                  frame True {
                    n289 = flat-sequence {
                      tunnel: [w342] -> w339
                      tunnel: [w341] -> w338
                      tunnel: w339 -> [w347]
                      tunnel: w338 -> [w345]
                      frame #0 {
                        n290 = local read "PicoHarp handle"() -> (w344:i32)
                        n291 = dll-call lib="F:/Users/Yuriy/Labview/JKU/StreamEye/StreamEye_master_v2_comp2015/PicoHarpLibrary/PHLib.dll" fn="PH_CloseDevice"("devidx"=w344) -> ("return type"=w343:i32)  [unwired: 4 in, 2 out]
                        n292 = Equal To 0?(x=w343) -> (x = 0?=w342:bool)
                        n293 = Not Equal To 0?(x=w343) -> (x != 0?=w341:bool)
                      }
                      frame #1 {
                        n294 = local write "PicoHarp error"(w345) -> ()
                        n295 = Not(x=w347) -> (.not. x?=w346:bool)
                        n296 = local write "PicoHarp ON"(w346) -> ()
                      }
                    }
                  }
                }
              }
              event "Apply PicoHarp Settings": Value Change {
                n297 = event-data() -> ()  [unwired: 1 in, 6 out]
                n298 = local read "PicoHarp ON"() -> (w348:bool)
                n299 = case shown="True" w348 {
                  frame False {
                  }
                  frame True {
                    n300 = flat-sequence {
                      tunnel: [w350] -> w349
                      tunnel: w349 -> [w365]
                      frame #0 {
                        n301 = local read "Sync div"() -> (w354:enum16{"1", "2", "4", "8"})
                        n302 = local read "Binning"() -> (w355:i32)
                        n303 = local read "PicoHarp handle"() -> (w350:i32)
                        n304 = local read "Ch0 ZeroX (mV)"() -> (w358:i32)
                        n305 = local read "Ch1 ZeroX (mV)"() -> (w356:i32)
                        n306 = local read "Ch0 Level (mV)"() -> (w359:i32)
                        n307 = local read "Ch1 Level (mV)"() -> (w357:i32)
                        n308 = Scale By Power Of 2(n=w354, x=1) -> (x*2^n=w360:i32)
                        n309 = call "Settings.vi"("StopOnOverflow"=TRUE, "DeviceIndex"=w350, "Range No."=w355, "SyncDiv"=w360, "CFD1 zero X"=w356, "CFD1 level"=w357, "CFD0 zero X"=w358, "CFD0 level"=w359) -> ("Resolution"=w351:i32, "Error"=w352:bool)  [unwired: 2 in]
                        n310 = local write "PicoHarp error"(w352) -> ()
                        n311 = local write "Res. (ps)"(w351) -> ()
                      }
                      frame #1 {
                        n312 = local read "SyncOffset (ps)"() -> (w364:i32)
                        n313 = dll-call lib="F:/Users/Yuriy/Labview/JKU/StreamEye/StreamEye_master_v2_comp2015/PicoHarpLibrary/phlib.dll" fn="PH_SetOffset"("devidx"=w365, "offset"=w364) -> ("return type"=w363:i32)  [unwired: 5 in, 2 out]
                        n314 = Less Than 0?(x=w363) -> (x < 0?=w362:bool)
                        n315 = local write "PicoHarp error"(w362) -> ()
                      }
                    }
                  }
                }
              }
              event "Start Histogram": Value Change {
                n316 = event-data() -> ()  [unwired: 1 in, 6 out]
                n317 = local read "Test Comp histo"() -> (w368:bool)
                n318 = local read "PicoHarp ON"() -> (w367:bool)
                n319 = Or(x=w367, y=w368) -> (x .or. y?=w366:bool)
                n320 = case shown="True" w366 {
                  tunnel: [0 20] -> w369
                  frame False {
                  }
                  frame True {
                  }
                }
              }
              event "Start Cursors Pair XY Sca": Value Change {
                n321 = event-data() -> ()  [unwired: 1 in, 6 out]
                n322 = local read "Data available Sca"() -> (w373:bool)
                n323 = case shown="True" w373 {
                  tunnel: [0 21] -> w372
                  frame False {
                  }
                  frame True {
                  }
                }
              }
              event "Start T2 Collect": Value Change {
                n324 = event-data() -> ()  [unwired: 1 in, 6 out]
                n325 = local read "PicoHarp ON"() -> (w378:bool)
                n326 = local read "TTTR ON"() -> (w377:bool)
                n327 = And(x=w377, y=w378) -> (x .and. y?=w376:bool)
                n328 = case shown="False" w376 {
                  tunnel: [0 22] -> w379
                  frame False {
                  }
                  frame True {
                  }
                }
              }
              event "Enable T2": Value Change {
                n329 = event-data() -> ()  [unwired: 1 in, 6 out]
                n330 = local read "PicoHarp ON"() -> (w382:bool)
                n331 = case shown="True" w382 {
                  tunnel: [18 0] -> w383
                  frame False {
                    n332 = flat-sequence {
                      tunnel: [w390] -> w384
                      tunnel: w384 -> [w400]
                      frame #0 {
                        n333 = local write "busy"(TRUE ("busy")) -> ()
                      }
                      frame #1 {
                        n334 = call "Initialization.vi"("Mode"=2) -> ("Deviceindex"=w394:i32, "Initialization Status"=w389:string, "DLL Version"=w388:string, "Initialisation Error"=w393:bool)  [unwired: 1 in]
                        n335 = local write "PicoHarp handle"(w394) -> ()
                        n336 = local write "Initialization Status"(w389) -> ()
                        n337 = case shown="False" w393 {
                          selector: w393 -> [_ w398]
                          tunnel: [w397 "Not calibrated"] -> w387
                          tunnel: [w396 w398] -> w392
                          tunnel: w394 -> [w395 _]
                          frame False {
                            n338 = call "Calibrate.vi"("Deviceindex"=w395) -> ("Calib Error"=w396:bool, "Status"=w397:string)  [unwired: 1 in]
                          }
                          frame True {
                          }
                        }
                        n339 = local write "DLL Version (must be 3.0)"(w388) -> ()
                        n340 = local write "Calibration Status"(w387) -> ()
                        n341 = local write "PicoHarp error"(w392) -> ()
                        n342 = Not(x=w392) -> (.not. x?=w390:bool)
                        n343 = local write "PicoHarp ON"(w390) -> ()
                        n344 = local write "TTTR ON"(w390) -> ()
                      }
                      frame #2 {
                        n345 = case shown="True" w400 {
                          frame False {
                          }
                          frame True {
                            n346 = local write "Signal source selection"(T1."Signal PicoHarp count rate" ("Signal source selection")) -> ()
                          }
                        }
                        n347 = local write "busy"(FALSE ("busy")) -> ()
                      }
                    }
                  }
                  frame True {
                    n348 = flat-sequence {
                      tunnel: [w409] -> w405
                      tunnel: [w408] -> w404
                      tunnel: w405 -> [w414]
                      tunnel: w404 -> [w412]
                      tunnel: [w418] -> w403
                      tunnel: w403 -> [w436]
                      frame #0 {
                        n349 = local write "busy"(TRUE ("busy")) -> ()
                      }
                      frame #1 {
                        n350 = local read "PicoHarp handle"() -> (w411:i32)
                        n351 = dll-call lib="F:/Users/Yuriy/Labview/JKU/StreamEye/StreamEye_master_v2_comp2015/PicoHarpLibrary/PHLib.dll" fn="PH_CloseDevice"("devidx"=w411) -> ("return type"=w410:i32)  [unwired: 4 in, 2 out]
                        n352 = Equal To 0?(x=w410) -> (x = 0?=w409:bool)
                        n353 = Not Equal To 0?(x=w410) -> (x != 0?=w408:bool)
                      }
                      frame #2 {
                        n354 = local write "PicoHarp error"(w412) -> ()
                        n355 = Not(x=w414) -> (.not. x?=w413:bool)
                        n356 = local write "PicoHarp ON"(w413) -> ()
                      }
                      frame #3 {
                        n357 = local read "TTTR ON"() -> (w420:bool)
                        n358 = case shown="False" w420 {
                          selector: w420 -> [w426 w428]
                          tunnel: [2 ("Mode") 0 ("Mode")] -> w421
                          tunnel: [w425 w429] -> w419
                          frame False {
                            n359 = Not(x=w426) -> (.not. x?=w425:bool)
                          }
                          frame True {
                            n360 = Not(x=w428) -> (.not. x?=w429:bool)
                          }
                        }
                        n361 = local write "TTTR ON"(w419) -> ()
                        n362 = call "Initialization.vi"("Mode"=w421) -> ("Deviceindex"=w422:i32, "Initialization Status"=w417:string, "DLL Version"=w416:string, "Initialisation Error"=w423:bool)  [unwired: 1 in]
                        n363 = local write "PicoHarp handle"(w422) -> ()
                        n364 = local write "Initialization Status"(w417) -> ()
                        n365 = case shown="False" w423 {
                          selector: w423 -> [_ w434]
                          tunnel: [w433 "Not calibrated"] -> w415
                          tunnel: [w432 w434] -> w424
                          tunnel: w422 -> [w431 _]
                          frame False {
                            n366 = call "Calibrate.vi"("Deviceindex"=w431) -> ("Calib Error"=w432:bool, "Status"=w433:string)  [unwired: 1 in]
                          }
                          frame True {
                          }
                        }
                        n367 = local write "DLL Version (must be 3.0)"(w416) -> ()
                        n368 = local write "Calibration Status"(w415) -> ()
                        n369 = local write "PicoHarp error"(w424) -> ()
                        n370 = Not(x=w424) -> (.not. x?=w418:bool)
                        n371 = local write "PicoHarp ON"(w418) -> ()
                      }
                      frame #4 {
                        n372 = case shown="True" w436 {
                          frame False {
                          }
                          frame True {
                            n373 = local write "Signal source selection"(T1."Signal PicoHarp count rate" ("Signal source selection")) -> ()
                          }
                        }
                        n374 = local write "busy"(FALSE ("busy")) -> ()
                      }
                    }
                  }
                }
              }
              event "Start Sync": Value Change {
                n375 = event-data() -> ()  [unwired: 1 in, 6 out]
                n376 = local read "Hosts Synchronized"() -> (w439:bool)
                n377 = case shown="True" w439 {
                  tunnel: [0 24] -> w440
                  frame False {
                  }
                  frame True {
                  }
                }
              }
            }
          }
          frame #1 {
            # "event handler"
            n378 = case shown="8" w443 {
              frame 0, Default {
              }
              frame 2 {
                # "init Scanner"
                n379 = flat-sequence {
                  frame #0 {
                    # "set speed?"
                    n380 = case shown="True" FALSE {
                      tunnel: [T9 {"Comm Method"=enum."RS232", "Com Port"=4, "Baud Rate"=57600, "IP Address"="10.0.10.84", "Remote Port"=23, "GPIB Address"="4", "VISA Resource Name"="ASRL3::INSTR", "Visa Baud Rate"=57600, "Visa Serial"=FALSE} ("Communication Parameter") w457] -> w445
                      tunnel: [T7 {"VENUS Language"=enum."VENUS 1", "Number of Axis"=2, "Controller Nr"=1, "Simulation"=FALSE} ("SMC Parameter") w456] -> w446
                      frame False {
                      }
                      frame True {
                        n381 = call "Dlg_Parameter.vi"() -> ("SMC Parameter"=w456:T7, "Communication Parameter"=w457:T9)  [unwired: 10 in]
                      }
                    }
                    n382 = call "SMC_INIT.vi"("SMC Parameter"=w446, "Communication Parameter"=w445) -> ("error out"=w449:errorcluster)  [unwired: 9 in]
                    n383 = case shown="False" FALSE {
                      tunnel: w449 -> [w450 w452]
                      tunnel: [w450 w451] -> w447
                      frame False {
                      }
                      frame True {
                        n384 = call "Dlg_Speed.vi"("error in (no error)"=w452) -> ("error out"=w451:errorcluster)  [unwired: 10 in]
                      }
                    }
                    "Scanner error out" <- w447
                    n385 = case shown="No Error" w447 {
                      frame No Error {
                        n386 = local write "Scanner ON"(TRUE ("Scanner ON")) -> ()
                      }
                      frame Error {
                      }
                    }
                  }
                  frame #1 {
                    n387 = global write "glb_stop.vi" "Stop Comm"(FALSE ("Stop Comm")) -> ()
                    n388 = local write "busy"(FALSE ("busy")) -> ()
                    n389 = local read "Xoffset_Sca"() -> (w468:dbl)
                    n390 = local read "Yoffset_Sca"() -> (w465:dbl)
                    n391 = global read "glb_pos.vi" "Position"() -> (w470:dbl[])
                    n392 = Index Array(array=w470, index #1=0 ("index"), index #2=1 ("index")) -> (element #1=w466:dbl, element #2=w462:dbl)
                    n393 = Multiply(x=w466, y=1000.0) -> (x*y=w469:dbl)
                    n394 = Multiply(x=w462, y=1000.0) -> (x*y=w464:dbl)
                    n395 = Subtract(x=w469, y=w468) -> (x-y=w467:dbl)
                    n396 = Subtract(x=w464, y=w465) -> (x-y=w463:dbl)
                    n397 = local write "Xread_Sca"(w467) -> ()
                    n398 = local write "Yread_Sca"(w463) -> ()
                  }
                }
              }
              frame 3 {
                # "init galvos"
                n399 = flat-sequence {
                  frame #0 {
                    w473 = -1 items=["Default"=-1, "RSE"=10083, "Differential"=10106, "Pseudodifferential"=12529] ("output terminal configuration")
                    w474 = -1 items=["Default"=-1, "RSE"=10083, "Differential"=10106, "Pseudodifferential"=12529] ("output terminal configuration")
                    w478 = 10348 items=["Volts"=10348, "From Custom Scale"=10065] ("units")
                    w484 = 10348 items=["Volts"=10348, "From Custom Scale"=10065] ("units")
                    # "Y"
                    # "X"
                    n400 = call-poly <vilib>:"DAQmx Create Virtual Channel.vi"("maximum value"=10.0, "minimum value"=-10.0, "output terminal configuration"=w474, "physical channels"=tag "Dev2/ao0" ("counter"), "name to assign"="Y-axis", "units"=w478) -> ("task out"=→"Galvo task out Y":refnum<k21>, "error out"=w477:errorcluster)  [unwired: 8 in]
                    "Galvo error out Y" <- w477
                    n401 = call-poly <vilib>:"DAQmx Create Virtual Channel.vi"("maximum value"=10.0, "minimum value"=-10.0, "output terminal configuration"=w473, "physical channels"=tag "Dev2/ao1" ("counter"), "name to assign"="X-axis", "units"=w484) -> ("task out"=→"Galvo task out X":refnum<k21>, "error out"=w483:errorcluster)  [unwired: 8 in]
                    "Galvo error out X" <- w483
                    n402 = case shown="No Error" w483 {
                      tunnel: w477 -> [w489 _]
                      frame No Error {
                        n403 = case shown="No Error" w489 {
                          frame No Error {
                            n404 = local write "Galvos ON"(TRUE ("Galvos ON")) -> ()
                          }
                          frame Error {
                          }
                        }
                      }
                      frame Error {
                      }
                    }
                  }
                  frame #1 {
                    n405 = local write "busy"(FALSE ("busy")) -> ()
                  }
                }
              }
              frame 5 {
                # "start streaming"
                n406 = property on="Spectrum Graph" class="XYGraph (strict)"() -> ("CrsrList"=w493:T11)  [unwired: 2 in, 2 out]
                n407 = control-ref of="Spectrum Graph"() -> (w501:refnum<vi>)
                n408 = local read "error reader"() -> (w504:errorcluster)
                n409 = local read "error writer"() -> (w506:errorcluster)
                n410 = control-ref of="time elapsed"() -> (w495:refnum<vi>)
                n411 = local read "reader endpoint"() -> (w505:refnum<k21>)
                n412 = local read "writer endpoint"() -> (w507:refnum<k21>)
                n413 = control-ref of="Time Trace"() -> (w503:refnum<vi>)
                n414 = control-ref of="Stop Measurement"() -> (w496:refnum<vi>)
                n415 = control-ref of="Current Intensity"() -> (w502:refnum<vi>)
                n416 = local read "Intensity mode selection"() -> (w494:T2)
                n417 = for {
                  tunnel: w493 -> [w510] mode=indexing
                  tunnel: [w508] -> w492 mode=indexing
                  n418 = Unbundle(w510) -> ("Position"=w509:cluster{"X":dbl, "Y":dbl})  [unwired: 15 out]
                  n419 = Unbundle(w509) -> ("X"=w508:dbl)  [unwired: 1 out]
                }
                n420 = call "subVI_get spectrum_master_v1.vi"("writer IN"=w507, "error writer IN"=w506, "reader IN"=w505, "error reader IN"=w504, "time trace IN"=w503, "intensity integral IN"=w502, "Stop IN"=w496, "reference XY graph IN"=w501, "Intensity mode selection"=w494, "reference time elapsed IN"=w495, "cursors positions"=w492) -> ("writer OUT"=w500:refnum<k21>, "error writer OUT"=w499:errorcluster, "reader OUT"=w498:refnum<k21>, "error reader OUT"=w497:errorcluster)  [unwired: 5 in]
                n421 = flat-sequence {
                  tunnel: w500 -> [w515]
                  tunnel: w499 -> [w514]
                  tunnel: w498 -> [w513]
                  tunnel: w497 -> [w512]
                  frame #0 {
                    n422 = local write "writer endpoint"(w515) -> ()
                    n423 = local write "error writer"(w514) -> ()
                    n424 = local write "reader endpoint"(w513) -> ()
                    n425 = local write "error reader"(w512) -> ()
                    n426 = local write "Stop Measurement"(FALSE ("Stop Measurement")) -> ()
                  }
                }
              }
              frame 8 {
                # "XW MegaArray"
                # "Start Hyperspectral Scanner"
                # "Y"
                # "X"
                n427 = local read "error reader"() -> (w536:errorcluster)
                n428 = local read "Xoffset_Sca"() -> (w532:dbl)
                n429 = local read "Yoffset_Sca"() -> (w529:dbl)
                n430 = local read "error writer"() -> (w538:errorcluster)
                n431 = local read "numPixels"() -> (w516:u16)
                n432 = local read "Xstart_Sca"() -> (w535:dbl)
                n433 = local read "Ystart_Sca"() -> (w530:dbl)
                n434 = local read "Xend_Sca"() -> (w533:dbl)
                n435 = local read "Yend_Sca"() -> (w528:dbl)
                n436 = property on="XYZ hyperspectral graph" class="IntGraph (strict)"("YScale.Offset"=-0.5 ("Y Scale.Offset and Multiplier:Offset"), "YScale.Multiplier"=1.0 ("Y Scale.Offset and Multiplier:Multiplier"), "YScale.Precision"=u8 0 ("X Scale.Display Format:Precision")) -> ()  [unwired: 2 in, 2 out]
                n437 = local read "reader endpoint"() -> (w537:refnum<k21>)
                n438 = local read "writer endpoint"() -> (w539:refnum<k21>)
                n439 = local read "Steps Hyperspectral Sca"() -> (w517:u32)
                n440 = Add(x=w535, y=w532) -> (x+y=w534:dbl)
                n441 = Add(x=w533, y=w532) -> (x+y=w531:dbl)
                n442 = Add(x=w530, y=w529) -> (x+y=w527:dbl)
                n443 = Add(x=w529, y=w528) -> (x+y=w526:dbl)
                n444 = call "subVI_RampGenerator.vi"("Number of Positions"=w517, "End  (um)"=w526, "Start  (um)"=w527) -> ("Array"=w520:dbl[])  [unwired: 1 in]
                n445 = local write "Yscale hyper"(w520) -> ()
                n446 = call "subVI_RampGenerator.vi"("Number of Positions"=w517, "End  (um)"=w531, "Start  (um)"=w534) -> ("Array"=w521:dbl[])  [unwired: 1 in]
                n447 = Initialize Array(0, w517, w516) -> (w525:i32[][])
                n448 = while {
                  tunnel: w517 -> [w571]
                  shift-right: [w568] -> w543
                  shift-left: w539 -> [w564]
                  shift-right: [w567] -> w542
                  shift-left: w538 -> [w563]
                  shift-right: [w566] -> w541
                  shift-left: w537 -> [w562]
                  shift-right: [w565] -> w540
                  shift-left: w536 -> [w561]
                  tunnel: w521 -> [w560]
                  tunnel: w520 -> [w559]
                  shift-right: [w558] -> w519
                  shift-left: w525 -> [w557]
                  i -> [w553]
                  stop <- w569 stop-if-true
                  n449 = flat-sequence {
                    tunnel: w559 -> [w574]
                    tunnel: w553 -> [w575]
                    tunnel: w560 -> [w576]
                    tunnel: [w576] -> w551
                    tunnel: [w575] -> w550
                    tunnel: [w574] -> w549
                    tunnel: [w578] -> w554
                    tunnel: w551 -> [w582]
                    tunnel: w550 -> [w578]
                    tunnel: w549 -> [w579]
                    tunnel: [w590] -> w555
                    tunnel: w554 -> [w590]
                    tunnel: [w607] -> w556
                    tunnel: w555 -> [w607]
                    tunnel: w564 -> [w619]
                    tunnel: w563 -> [w618]
                    tunnel: w562 -> [w617]
                    tunnel: w561 -> [w616]
                    tunnel: w557 -> [w614]
                    tunnel: w556 -> [w613]
                    tunnel: [w623] -> w548
                    tunnel: [w622] -> w547
                    tunnel: [w621] -> w546
                    tunnel: [w620] -> w545
                    tunnel: [w615] -> w544
                    tunnel: [w799] -> w558
                    tunnel: [w800] -> w565
                    tunnel: [w801] -> w566
                    tunnel: [w802] -> w567
                    tunnel: [w803] -> w568
                    tunnel: w548 -> [w803]
                    tunnel: w547 -> [w802]
                    tunnel: w546 -> [w801]
                    tunnel: w545 -> [w800]
                    tunnel: w544 -> [w799]
                    frame #0 {
                      n450 = Tick Count (ms)() -> (millisecond timer value=w573:u32)
                      n451 = local write "time start"(w573) -> ()
                    }
                    frame #1 {
                      # "um to mm"
                      # "go"
                      n452 = Index Array(array=w582, index=w578) -> (element=w581:dbl)
                      n453 = Index Array(array=w579, index=w578) -> (element=w580:dbl)
                      n454 = local read "Wait Scan."() -> (w577:bool)
                      n455 = Divide(x=w581, y=1000.0) -> (x/y=w588:dbl)
                      n456 = Divide(x=w580, y=1000.0) -> (x/y=w587:dbl)
                      n457 = local read "Scanner error out"() -> (w589:errorcluster)
                      n458 = Build Array(w588, w587) -> (w586:dbl[])
                      n459 = call "SMC_MoveAbs.vi"("error in (no error)"=w589, "WaitUntilReady"=w577, "Input Array"=w586) -> ("error out"=w585:errorcluster)  [unwired: 8 in]
                      n460 = local write "Scanner error out"(w585) -> ()
                    }
                    frame #2 {
                      # "wait"
                      n461 = local read "Xdelay_Sca"() -> (w593:dbl)
                      n462 = Multiply(x=w593, y=1000.0) -> (x*y=w591:dbl)
                      n463 = Wait (ms)(milliseconds to wait=w591) -> ()  [unwired: 1 out]
                    }
                    frame #3 {
                      # "read"
                      n464 = local read "Xoffset_Sca"() -> (w598:dbl)
                      n465 = local read "Yoffset_Sca"() -> (w603:dbl)
                      n466 = global read "glb_pos.vi" "Position"() -> (w594:dbl[])
                      n467 = Index Array(array=w594, index #1=0 ("index"), index #2=1 ("index")) -> (element #1=w601:dbl, element #2=w606:dbl)
                      n468 = Multiply(x=w601, y=1000.0) -> (x*y=w597:dbl)
                      n469 = Multiply(x=w606, y=1000.0) -> (x*y=w604:dbl)
                      n470 = Subtract(x=w597, y=w598) -> (x-y=w600:dbl)
                      n471 = Subtract(x=w604, y=w603) -> (x-y=w605:dbl)
                      n472 = local write "Xread_Sca"(w600) -> ()
                      n473 = local write "Yread_Sca"(w605) -> ()
                    }
                    frame #4 {
                      # "get spectrum"
                      n474 = local read "Hosts Synchronized"() -> (w612:bool)
                      n475 = local read "Signal source selection"() -> (w609:T1)
                      n476 = Equal?(x=w609, y=T1."Signal Stream" ("Signal source selection")) -> (x = y?=w608:bool)
                      n477 = And(x=w612, y=w608) -> (x .and. y?=w611:bool)
                      n478 = case shown="True" w611 {
                        tunnel: [w630 w757] -> w623
                        tunnel: [w629 w756] -> w622
                        tunnel: [w628 w755] -> w621
                        tunnel: [w627 w746] -> w620
                        tunnel: w619 -> [w630 w754]
                        tunnel: w618 -> [w629 w753]
                        tunnel: w617 -> [w628 w752]
                        tunnel: w616 -> [w627 w751]
                        tunnel: [w626 w734] -> w615
                        tunnel: w614 -> [w626 w728]
                        tunnel: w613 -> [_ w727]
                        frame False {
                          n479 = local read "PicoHarp ON"() -> (w625:bool)
                          n480 = case shown="True" w625 {
                            tunnel: [w631 w633] -> w624
                            frame False {
                              n481 = Random Number (0-1)() -> (number: 0 to 1=w631:dbl)
                            }
                            frame True {
                              n482 = local read "PicoHarp handle"() -> (w632:i32)
                              n483 = local read "Signal source selection"() -> (w634:T1)
                              n484 = case shown="\"Signal Stream\"" w634 {
                                tunnel: [w635 w636 w643 w701] -> w633
                                tunnel: w632 -> [_ _ w648 w703]
                                frame "Signal None", Default {
                                n485 = Random Number (0-1)() -> (number: 0 to 1=w635:dbl)
                                }
                                frame "Signal Stream" {
                                n486 = Random Number (0-1)() -> (number: 0 to 1=w636:dbl)
                                }
                                frame "Signal PicoHarp histro" {
                                w650 = u16 65535 ("Number of Positions")
                                n487 = local read "Res. (ps)"() -> (w656:i32)
                                n488 = Initialize Array "Initialize Array"(u32 0, 65536) -> (w654:u32[])
                                n489 = local read "Histo Time (s)"() -> (w647:dbl)
                                n490 = local read "Integration Number (#)"() -> (w645:i32)
                                n491 = local read "Autosave Histograms"() -> (w640:bool)
                                n492 = Divide(x=w656, y=1000) -> (x/y=w655:dbl)
                                n493 = To Long Integer(number=w647) -> (32bit integer=w638:i32)
                                n494 = Multiply(x=w655, y=w650) -> (x*y=w657:dbl)
                                n495 = Multiply(x=w638, y=1000) -> (x*y=w637:i32)
                                n496 = call "subVI_RampGenerator.vi"("Number of Positions"=w650, "End  (um)"=w657, "Start  (um)"=0.0) -> ("Array"=w642:dbl[])  [unwired: 1 in]
                                n497 = for {
                                N: w645 -> [_]
                                tunnel: w637 -> [w692]
                                tunnel: w648 -> [w690]
                                shift-right: [w687] -> w641
                                shift-left: w654 -> [w691]
                                tunnel: w642 -> [w689]
                                tunnel: [w682] -> w646 mode=indexing
                                i -> [w683]
                                stop <- w679 stop-if-true
                                n498 = call "Start Measurement.vi"("Acquisition time"=w692, "DeviceIndex"=w690) -> ("DataValid"=w693:bool)
                                n499 = case shown="True" w693 {
                                tunnel: [u32 0 w700] -> w682
                                tunnel: w690 -> [_ w699]
                                tunnel: [w694 w696] -> w687
                                tunnel: w691 -> [w694 w698]
                                frame False {
                                }
                                frame True {
                                n500 = call "Get Histogram.vi"("DeviceIndex"=w699) -> ("Histogram"=w697:u32[], "IntegralCount"=w700:i32)  [unwired: 1 in, 1 out]
                                n501 = Add(x=w698, y=w697) -> (x+y=w696:u32[])
                                }
                                }
                                n502 = local read "Acc. Threshold (cts)"() -> (w685:i64)
                                n503 = local read "Stop Measurement"() -> (w681:bool)
                                n504 = local write "Current Intensity"(w682) -> ()
                                n505 = Less?(x=w682, y=w685) -> (x < y?=w686:bool)
                                n506 = Bundle("Array"=w689, w687) -> (w688:cluster{"Array":dbl[], u32[]})  [unwired: 1 in]
                                n507 = local write "Histo Graph"(w688) -> ()
                                n508 = Equal To 0?(x=w683) -> (x = 0?=w684:bool)
                                n509 = And(x=w686, y=w684) -> (x .and. y?=w680:bool)
                                n510 = Or(x=w680, y=w681) -> (x .or. y?=w679:bool)
                                }
                                n511 = case shown="True" w640 {
                                tunnel: w642 -> [_ w673]
                                tunnel: w641 -> [_ w661]
                                frame False {
                                }
                                frame True {
                                n512 = local read "Filaname"() -> (w676:string)
                                n513 = local read "Filaname"() -> (w664:string)
                                n514 = Get Date/Time In Seconds() -> (seconds since 1Jan1904=w659:timestamp)
                                n515 = Format Date/Time String(time format string (%c)="_%Y%m%d_%H%M%S_", seconds (now)=w659) -> (date/time string=w658:string)  [unwired: 1 in]
                                n516 = Concatenate Strings("Histo_", w664, w658, ".dat") -> (w663:string)
                                n517 = Concatenate Strings("Tscale_", w676, w658, ".dat") -> (w677:string)
                                n518 = local read "Path"() -> (w665:path)
                                n519 = local read "Path"() -> (w675:path)
                                n520 = Build Path(base path=w665, name or relative path=w663) -> (appended path=w662:path)
                                n521 = Build Path(base path=w675, name or relative path=w677) -> (appended path=w678:path)
                                n522 = call-poly <vilib>:"Write Delimited Spreadsheet.vi"("file path (dialog if empty)"=w662, "1D data"=w661, "append to file? (new file:F)"=FALSE, "transpose? (no:F)"=TRUE) -> ()  [unwired: 10 in, 2 out]
                                n523 = call-poly <vilib>:"Write Delimited Spreadsheet.vi"("file path (dialog if empty)"=w678, "1D data"=w673, "append to file? (new file:F)"=FALSE, "transpose? (no:F)"=TRUE) -> ()  [unwired: 10 in, 2 out]
                                }
                                }
                                n524 = Add Array Elements(numeric array=w646) -> (sum=w644:u32)
                                n525 = Divide(x=w644, y=w645) -> (x/y=w643:dbl)
                                }
                                frame "Signal PicoHarp count rate" {
                                n526 = dll-call lib="F:/Users/Yuriy/Labview/JKU/StreamEye/StreamEye_master_v2_comp2015/PicoHarpLibrary/PHLib.dll" fn="PH_GetCountRate"("devidx"=w703, "channel"=1, "rate"=0) -> ("rate"=w702:i32)  [unwired: 6 in, 2 out]
                                n527 = local read "Acc. Threshold (cts)"() -> (w705:i64)
                                n528 = Greater?(x=w702, y=w705) -> (0:w704:bool)
                                n529 = case shown="True" w704 {
                                tunnel: w703 -> [_ w713]
                                tunnel: [w708 w710] -> w701
                                tunnel: w702 -> [w708 w709]
                                frame False {
                                }
                                frame True {
                                n530 = local read "Integration Number (#)"() -> (w711:i32)
                                n531 = Decrement(x=w711) -> (x-1=w714:i32)
                                n532 = for {
                                N: w714 -> [_]
                                shift-right: [w717] -> w712
                                shift-left: w709 -> [w718]
                                tunnel: w713 -> [w719]
                                stop <- w715 stop-if-true
                                n533 = dll-call lib="F:/Users/Yuriy/Labview/JKU/StreamEye/StreamEye_master_v2_comp2015/PicoHarpLibrary/PHLib.dll" fn="PH_GetCountRate"("devidx"=w719, "channel"=1, "rate"=0) -> ("rate"=w716:i32)  [unwired: 6 in, 2 out]
                                n534 = local read "Stop Measurement"() -> (w715:bool)
                                n535 = local write "Current Intensity"(w716) -> ()
                                n536 = local write "Time Trace"(w716) -> ()
                                n537 = Add(x=w718, y=w716) -> (x+y=w717:i32)
                                }
                                n538 = Divide(x=w712, y=w711) -> (x/y=w710:dbl)
                                }
                                }
                                }
                              }
                            }
                          }
                          n539 = local write "Current Intensity"(w624) -> ()
                          n540 = local write "Time Trace"(w624) -> ()
                        }
                        frame True {
                          n541 = property on="Spectrum Graph" class="XYGraph (strict)"() -> ("CrsrList"=w743:T11)  [unwired: 2 in, 2 out]
                          n542 = control-ref of="Spectrum Graph"() -> (w748:refnum<vi>)
                          n543 = local write "Data available XW"(TRUE ("Data available XW")) -> ()
                          n544 = control-ref of="time elapsed dummy"() -> (w744:refnum<vi>)
                          n545 = control-ref of="Time Trace"() -> (w750:refnum<vi>)
                          n546 = control-ref of="single spectrum?"() -> (w747:refnum<vi>)
                          n547 = control-ref of="Current Intensity"() -> (w749:refnum<vi>)
                          n548 = local read "Intensity mode selection"() -> (w742:T2)
                          n549 = local read "Integration Number (#)"() -> (w724:i32)
                          n550 = for {
                            tunnel: w743 -> [w793] mode=indexing
                            tunnel: [w791] -> w741 mode=indexing
                            n551 = Unbundle(w793) -> ("Position"=w792:cluster{"X":dbl, "Y":dbl})  [unwired: 15 out]
                            n552 = Unbundle(w792) -> ("X"=w791:dbl)  [unwired: 1 out]
                          }
                          n553 = for {
                            N: w724 -> [_]
                            tunnel: [w785] -> w757
                            tunnel: [w783] -> w755
                            tunnel: w754 -> [w782]
                            tunnel: w752 -> [w780]
                            tunnel: w750 -> [w778]
                            tunnel: w749 -> [w777]
                            tunnel: w748 -> [w776]
                            tunnel: w747 -> [w775]
                            tunnel: w744 -> [w772]
                            tunnel: w742 -> [w771]
                            tunnel: w741 -> [w770]
                            tunnel: [w769] -> w729
                            tunnel: [w768] -> w723 mode=indexing
                            shift-right: [w784] -> w756
                            shift-left: w753 -> [w781]
                            shift-right: [w773] -> w746
                            shift-left: w751 -> [w779]
                            i -> [w762]
                            stop <- w761 stop-if-true
                            n554 = call "subVI_get spectrum_master_v1.vi"("writer IN"=w782, "error writer IN"=w781, "reader IN"=w780, "error reader IN"=w779, "time trace IN"=w778, "intensity integral IN"=w777, "Stop IN"=w775, "reference XY graph IN"=w776, "Intensity mode selection"=w771, "reference time elapsed IN"=w772, "cursors positions"=w770) -> ("writer OUT"=w785:refnum<k21>, "error writer OUT"=w784:errorcluster, "reader OUT"=w783:refnum<k21>, "error reader OUT"=w774:errorcluster)  [unwired: 5 in]
                            n555 = flat-sequence {
                              tunnel: w774 -> [w790]
                              tunnel: [w790] -> w773
                              tunnel: [w788] -> w769
                              tunnel: [w787] -> w768
                              tunnel: [w786] -> w760
                              frame #0 {
                                n556 = local read "Current Intensity"() -> (w786:dbl)
                                n557 = local read "Spectrum Graph"() -> (w789:T4)
                                n558 = Unbundle(w789) -> ("Calibrated Array"=w788:dbl[], "Array F32"=w787:sgl[])
                              }
                            }
                            n559 = local read "Acc. Threshold (cts)"() -> (w764:i64)
                            n560 = local read "Stop Measurement"() -> (w767:bool)
                            n561 = Less?(x=w760, y=w764) -> (x < y?=w763:bool)
                            n562 = Equal To 0?(x=w762) -> (x = 0?=w765:bool)
                            n563 = And(x=w763, y=w765) -> (x .and. y?=w766:bool)
                            n564 = Or(x=w766, y=w767) -> (x .or. y?=w761:bool)
                          }
                          n565 = local write "Wscale hyper"(w729) -> ()
                          n566 = Transpose 2D Array(2D array=w723) -> (transposed array=w722:sgl[][])
                          n567 = Index Array(array=w729, index=1) -> (element=w736:dbl)
                          n568 = Index Array(array=w729, index=0) -> (element=w739:dbl)
                          n569 = for {
                            tunnel: w722 -> [w759] mode=indexing
                            tunnel: [w758] -> w726 mode=indexing
                            n570 = Add Array Elements(numeric array=w759) -> (sum=w758:sgl)
                          }
                          n571 = Subtract(x=w736, y=w739) -> (x-y=w738:dbl)
                          n572 = Divide(x=w738, y=2.0) -> (x/y=w737:dbl)
                          n573 = Subtract(x=w739, y=w737) -> (x-y=w740:dbl)
                          n574 = Divide(x=w726, y=w724) -> (x/y=w725:sgl[])
                          n575 = property on="XYZ hyperspectral graph" class="IntGraph (strict)"("XScale.Offset"=w740, "XScale.Multiplier"=w738, "XScale.Precision"=u8 2 ("X Scale.Display Format:Precision")) -> ()  [unwired: 2 in, 2 out]
                          n576 = Replace Array Subset(array=w728, new element=w725, index (row)=w727) -> (w734:i32[][])  [unwired: 1 in]
                          n577 = Transpose 2D Array(2D array=w734) -> (transposed array=w735:i32[][])
                          n578 = local write "XYZ hyperspectral graph"(w735) -> ()
                        }
                      }
                    }
                    frame #5 {
                      n579 = local read "time start"() -> (w797:i32)
                      n580 = Tick Count (ms)() -> (millisecond timer value=w798:u32)
                      n581 = Subtract(x=w798, y=w797) -> (x-y=w796:u32)
                      n582 = Divide(x=w796, y=u32 1000) -> (x/y=w794:dbl)
                      n583 = local write "time elapsed"(w794) -> ()
                    }
                  }
                  n584 = Increment(x=w553) -> (x+1=w552:i32)
                  n585 = local read "Stop Measurement"() -> (w570:bool)
                  n586 = Equal?(x=w552, y=w571) -> (x = y?=w572:bool)
                  n587 = Or(x=w570, y=w572) -> (x .or. y?=w569:bool)
                }
                n588 = local write "Xscale hyper"(w521) -> ()
                n589 = flat-sequence {
                  tunnel: w543 -> [w808]
                  tunnel: w542 -> [w807]
                  tunnel: w541 -> [w806]
                  tunnel: w540 -> [w805]
                  frame #0 {
                    n590 = local write "writer endpoint"(w808) -> ()
                    n591 = local write "error writer"(w807) -> ()
                    n592 = local write "reader endpoint"(w806) -> ()
                    n593 = local write "error reader"(w805) -> ()
                    n594 = local write "Stop Measurement"(FALSE ("Stop Measurement")) -> ()
                  }
                }
                n595 = local write "XW MegaArray"(w519) -> ()
              }
              frame 9 {
                # "XYZ Array"
                # "XYZ MegaArray"
                # "Start Image Scanner"
                n596 = local read "Xoffset_Sca"() -> (w854:dbl)
                n597 = local read "Yoffset_Sca"() -> (w852:dbl)
                n598 = local read "error reader"() -> (w856:errorcluster)
                n599 = local read "error writer"() -> (w858:errorcluster)
                n600 = local read "Xsteps_Sca"() -> (w836:u32)
                n601 = local read "Ysteps_Sca"() -> (w837:u32)
                n602 = local read "numPixels"() -> (w809:u16)
                n603 = local read "Xstep_Sca"() -> (w829:dbl)
                n604 = local read "Ystep_Sca"() -> (w816:dbl)
                n605 = local read "Xstart_Sca"() -> (w826:dbl)
                n606 = local read "Ystart_Sca"() -> (w813:dbl)
                n607 = local read "Xend_Sca"() -> (w825:dbl)
                n608 = local read "Yend_Sca"() -> (w814:dbl)
                n609 = local read "reader endpoint"() -> (w857:refnum<k21>)
                n610 = local read "writer endpoint"() -> (w859:refnum<k21>)
                n611 = Greater?(x=w825, y=w826) -> (0:w830:bool)
                n612 = Add(x=w825, y=w854) -> (x+y=w853:dbl)
                n613 = Add(x=w813, y=w852) -> (x+y=w851:dbl)
                n614 = Greater?(x=w814, y=w813) -> (0:w817:bool)
                n615 = Add(x=w852, y=w814) -> (x+y=w850:dbl)
                n616 = Divide(x=w816, y=2.0) -> (x/y=w812:dbl)
                n617 = Add(x=w826, y=w854) -> (x+y=w855:dbl)
                n618 = call "subVI_RampGenerator.vi"("Number of Positions"=w837, "End  (um)"=w850, "Start  (um)"=w851) -> ("Array"=w845:dbl[])  [unwired: 1 in]
                n619 = Divide(x=w829, y=2.0) -> (x/y=w822:dbl)
                n620 = Select(t=1.0, s=w830, f=-1.0) -> (s? t:f=w821:dbl)
                n621 = Select(t=1.0, s=w817, f=-1.0) -> (s? t:f=w810:dbl)
                n622 = local write "Yscale Sca"(w845) -> ()
                n623 = Multiply(x=w822, y=w821) -> (x*y=w820:dbl)
                n624 = Multiply(x=w821, y=w829) -> (x*y=w828:dbl)
                n625 = Multiply(x=w812, y=w810) -> (x*y=w811:dbl)
                n626 = Multiply(x=w810, y=w816) -> (x*y=w815:dbl)
                n627 = call "subVI_RampGenerator.vi"("Number of Positions"=w836, "End  (um)"=w853, "Start  (um)"=w855) -> ("Array"=w844:dbl[])  [unwired: 1 in]
                n628 = local write "Xscale Sca"(w844) -> ()
                n629 = Subtract(x=w826, y=w820) -> (x-y=w823:dbl)
                n630 = Subtract(x=w813, y=w811) -> (x-y=w831:dbl)
                n631 = Initialize Array(0.0 ("element"), w836, w837) -> (w839:dbl[][])
                n632 = Initialize Array(0.0 ("element"), w836, w837, w809) -> (w842:dbl[][][])
                n633 = while {
                  tunnel: w836 -> [w880]
                  tunnel: w844 -> [w875]
                  tunnel: w845 -> [w874]
                  shift-right: [w872] -> w848
                  shift-left: w858 -> [w878]
                  shift-right: [w870] -> w846
                  shift-left: w856 -> [w876]
                  shift-right: [w873] -> w849
                  shift-left: w859 -> [w879]
                  shift-right: [w871] -> w847
                  shift-left: w857 -> [w877]
                  tunnel: w837 -> [w866]
                  shift-right: [w865] -> w841
                  shift-left: w842 -> [w864]
                  shift-right: [w862] -> w838
                  shift-left: w839 -> [w863]
                  i -> [w861]
                  stop <- w869 stop-if-true
                  n634 = while {
                    tunnel: w880 -> [w917]
                    shift-right: [w915] -> w873
                    shift-left: w879 -> [w911]
                    shift-right: [w914] -> w872
                    shift-left: w878 -> [w910]
                    shift-right: [w913] -> w871
                    shift-left: w877 -> [w909]
                    shift-right: [w912] -> w870
                    shift-left: w876 -> [w908]
                    tunnel: w875 -> [w907]
                    tunnel: w874 -> [w906]
                    tunnel: [w905] -> w867
                    shift-right: [w900] -> w865
                    shift-left: w864 -> [w899]
                    tunnel: w861 -> [w898]
                    tunnel: w861 -> [w897]
                    shift-right: [w895] -> w862
                    shift-left: w863 -> [w896]
                    i -> [w893]
                    stop <- w916 stop-if-true
                    n635 = flat-sequence {
                      tunnel: w897 -> [w920]
                      tunnel: w899 -> [w921]
                      tunnel: w893 -> [w922]
                      tunnel: w906 -> [w923]
                      tunnel: w893 -> [w924]
                      tunnel: w907 -> [w925]
                      tunnel: [w925] -> w892
                      tunnel: [w924] -> w891
                      tunnel: [w923] -> w890
                      tunnel: [w922] -> w889
                      tunnel: [w921] -> w888
                      tunnel: [w920] -> w887
                      tunnel: [w935] -> w904
                      tunnel: [w934] -> w901
                      tunnel: w892 -> [w940]
                      tunnel: w891 -> [w938]
                      tunnel: w890 -> [w936]
                      tunnel: w889 -> [w935]
                      tunnel: w888 -> [w934]
                      tunnel: w887 -> [w933]
                      tunnel: w904 -> [w957]
                      tunnel: [w955] -> w902
                      tunnel: w901 -> [w955]
                      tunnel: [w965] -> w903
                      tunnel: w902 -> [w965]
                      tunnel: w911 -> [w993]
                      tunnel: w910 -> [w992]
                      tunnel: w909 -> [w991]
                      tunnel: w908 -> [w990]
                      tunnel: w903 -> [w989]
                      tunnel: w893 -> [w987]
                      tunnel: w898 -> [w986]
                      tunnel: w896 -> [w985]
                      tunnel: [w997] -> w886
                      tunnel: [w996] -> w885
                      tunnel: [w995] -> w884
                      tunnel: [w994] -> w883
                      tunnel: [w988] -> w882
                      tunnel: [w984] -> w881
                      tunnel: [w1173] -> w895
                      tunnel: [w1174] -> w900
                      tunnel: [w1175] -> w912
                      tunnel: [w1176] -> w913
                      tunnel: [w1177] -> w914
                      tunnel: [w1178] -> w915
                      tunnel: w886 -> [w1178]
                      tunnel: w885 -> [w1177]
                      tunnel: w884 -> [w1176]
                      tunnel: w883 -> [w1175]
                      tunnel: w882 -> [w1174]
                      tunnel: w881 -> [w1173]
                      frame #0 {
                        n636 = Tick Count (ms)() -> (millisecond timer value=w919:u32)
                        n637 = local write "time start"(w919) -> ()
                      }
                      frame #1 {
                        # "um to mm"
                        # "go"
                        n638 = Index Array(array=w940, index=w938) -> (element=w939:dbl)
                        n639 = Index Array(array=w936, index=w933) -> (element=w937:dbl)
                        n640 = local read "Wait Scan."() -> (w930:bool)
                        n641 = Divide(x=w937, y=1000.0) -> (x/y=w927:dbl)
                        n642 = local read "Scanner error out"() -> (w943:errorcluster)
                        n643 = local read "Compensate"() -> (w932:bool)
                        n644 = Divide(x=w939, y=1000.0) -> (x/y=w926:dbl)
                        n645 = Build Array(w926, w927) -> (w929:dbl[])
                        n646 = call "SMC_MoveAbs.vi"("error in (no error)"=w943, "WaitUntilReady"=w930, "Input Array"=w929) -> ("error out"=w931:errorcluster)  [unwired: 8 in]
                        n647 = case shown="True" w932 {
                          tunnel: w931 -> [w944 w954]
                          tunnel: w930 -> [_ w952]
                          tunnel: w929 -> [_ w951]
                          tunnel: [w944 w950] -> w928
                          tunnel: w927 -> [_ w949]
                          tunnel: w926 -> [_ w947]
                          frame False {
                          }
                          frame True {
                            n648 = Subtract(x=w947, y=0.0002) -> (x-y=w946:dbl)
                            n649 = Build Array(w946, w949) -> (w945:dbl[])
                            n650 = call "SMC_MoveAbs.vi"("error in (no error)"=w954, "WaitUntilReady"=w952, "Input Array"=w945) -> ("error out"=w953:errorcluster)  [unwired: 8 in]
                            n651 = call "SMC_MoveAbs.vi"("error in (no error)"=w953, "WaitUntilReady"=w952, "Input Array"=w951) -> ("error out"=w950:errorcluster)  [unwired: 8 in]
                          }
                        }
                        n652 = local write "Scanner error out"(w928) -> ()
                      }
                      frame #2 {
                        # "wait"
                        n653 = Equal?(x=w957, y=0) -> (x = y?=w958:bool)
                        n654 = local read "Xdelay_Sca"() -> (w961:dbl)
                        n655 = case shown="True" w958 {
                          frame False {
                          }
                          frame True {
                            # "first in the line"
                            n656 = local read "Ydelay_Sca"() -> (w962:dbl)
                            n657 = Multiply(x=w962, y=1000.0) -> (x*y=w964:dbl)
                            n658 = Wait (ms)(milliseconds to wait=w964) -> ()  [unwired: 1 out]
                          }
                        }
                        n659 = Multiply(x=w961, y=1000.0) -> (x*y=w959:dbl)
                        n660 = Wait (ms)(milliseconds to wait=w959) -> ()  [unwired: 1 out]
                      }
                      frame #3 {
                        # "read"
                        n661 = local read "Xoffset_Sca"() -> (w970:dbl)
                        n662 = local read "Yoffset_Sca"() -> (w975:dbl)
                        n663 = global read "glb_pos.vi" "Position"() -> (w966:dbl[])
                        n664 = Index Array(array=w966, index #1=0 ("index"), index #2=1 ("index")) -> (element #1=w973:dbl, element #2=w978:dbl)
                        n665 = Multiply(x=w973, y=1000.0) -> (x*y=w969:dbl)
                        n666 = Multiply(x=w978, y=1000.0) -> (x*y=w976:dbl)
                        n667 = Subtract(x=w969, y=w970) -> (x-y=w972:dbl)
                        n668 = Subtract(x=w976, y=w975) -> (x-y=w977:dbl)
                        n669 = local write "Xread_Sca"(w972) -> ()
                        n670 = local write "Yread_Sca"(w977) -> ()
                      }
                      frame #4 {
                        # "get spectrum"
                        n671 = local read "Hosts Synchronized"() -> (w983:bool)
                        n672 = local read "Signal source selection"() -> (w981:T1)
                        n673 = Equal?(x=w981, y=T1."Signal Stream" ("Signal source selection")) -> (x = y?=w979:bool)
                        n674 = And(x=w983, y=w979) -> (x .and. y?=w982:bool)
                        n675 = case shown="True" w982 {
                          tunnel: [w1009 w1131] -> w997
                          tunnel: [w1008 w1130] -> w996
                          tunnel: [w1007 w1129] -> w995
                          tunnel: [w1006 w1119] -> w994
                          tunnel: w993 -> [w1009 w1128]
                          tunnel: w992 -> [w1008 w1127]
                          tunnel: w991 -> [w1007 w1126]
                          tunnel: w990 -> [w1006 w1125]
                          tunnel: w989 -> [w1005 w1112]
                          tunnel: [w1005 w1111] -> w988
                          tunnel: w987 -> [w1004 w1118]
                          tunnel: w986 -> [w1003 w1117]
                          tunnel: w985 -> [w1002 w1110]
                          tunnel: [w1001 w1109] -> w984
                          frame False {
                            n676 = local write "Data available Sca"(TRUE ("Data available Sca")) -> ()
                            n677 = local read "PicoHarp ON"() -> (w999:bool)
                            n678 = case shown="True" w999 {
                              tunnel: [w1010 w1011] -> w998
                              frame False {
                                n679 = Random Number (0-1)() -> (number: 0 to 1=w1010:dbl)
                              }
                              frame True {
                                n680 = local read "PicoHarp handle"() -> (w1012:i32)
                                n681 = local read "Signal source selection"() -> (w1013:T1)
                                n682 = case shown="\"Signal PicoHarp count rate\"" w1013 {
                                tunnel: [w1014 w1015 w1022 w1080] -> w1011
                                tunnel: w1012 -> [_ _ w1027 w1082]
                                frame "Signal None", Default {
                                n683 = Random Number (0-1)() -> (number: 0 to 1=w1014:dbl)
                                }
                                frame "Signal Stream" {
                                n684 = Random Number (0-1)() -> (number: 0 to 1=w1015:dbl)
                                }
                                frame "Signal PicoHarp histro" {
                                w1029 = u16 65535 ("Number of Positions")
                                n685 = local read "Res. (ps)"() -> (w1035:i32)
                                n686 = Initialize Array "Initialize Array"(u32 0, 65536) -> (w1033:u32[])
                                n687 = local read "Histo Time (s)"() -> (w1026:dbl)
                                n688 = local read "Integration Number (#)"() -> (w1024:i32)
                                n689 = local read "Autosave Histograms"() -> (w1019:bool)
                                n690 = Divide(x=w1035, y=1000) -> (x/y=w1034:dbl)
                                n691 = To Long Integer(number=w1026) -> (32bit integer=w1017:i32)
                                n692 = Multiply(x=w1034, y=w1029) -> (x*y=w1036:dbl)
                                n693 = Multiply(x=w1017, y=1000) -> (x*y=w1016:i32)
                                n694 = call "subVI_RampGenerator.vi"("Number of Positions"=w1029, "End  (um)"=w1036, "Start  (um)"=0.0) -> ("Array"=w1021:dbl[])  [unwired: 1 in]
                                n695 = for {
                                N: w1024 -> [_]
                                tunnel: w1016 -> [w1071]
                                tunnel: w1027 -> [w1069]
                                shift-right: [w1066] -> w1020
                                shift-left: w1033 -> [w1070]
                                tunnel: w1021 -> [w1068]
                                tunnel: [w1061] -> w1023 mode=indexing
                                i -> [w1062]
                                stop <- w1058 stop-if-true
                                n696 = call "Start Measurement.vi"("Acquisition time"=w1071, "DeviceIndex"=w1069) -> ("DataValid"=w1072:bool)
                                n697 = local read "Acc. Threshold (cts)"() -> (w1064:i64)
                                n698 = local read "Stop Measurement"() -> (w1060:bool)
                                n699 = case shown="True" w1072 {
                                tunnel: [u32 0 w1079] -> w1061
                                tunnel: w1069 -> [_ w1078]
                                tunnel: [w1073 w1075] -> w1066
                                tunnel: w1070 -> [w1073 w1077]
                                frame False {
                                }
                                frame True {
                                n700 = call "Get Histogram.vi"("DeviceIndex"=w1078) -> ("Histogram"=w1076:u32[], "IntegralCount"=w1079:i32)  [unwired: 1 in, 1 out]
                                n701 = Add(x=w1077, y=w1076) -> (x+y=w1075:u32[])
                                }
                                }
                                n702 = local write "Current Intensity"(w1061) -> ()
                                n703 = Less?(x=w1061, y=w1064) -> (x < y?=w1065:bool)
                                n704 = Bundle("Array"=w1068, w1066) -> (w1067:cluster{"Array":dbl[], u32[]})  [unwired: 1 in]
                                n705 = local write "Histo Graph"(w1067) -> ()
                                n706 = Equal To 0?(x=w1062) -> (x = 0?=w1063:bool)
                                n707 = And(x=w1065, y=w1063) -> (x .and. y?=w1059:bool)
                                n708 = Or(x=w1059, y=w1060) -> (x .or. y?=w1058:bool)
                                }
                                n709 = case shown="True" w1019 {
                                tunnel: w1021 -> [_ w1043]
                                tunnel: w1020 -> [_ w1042]
                                frame False {
                                }
                                frame True {
                                n710 = local read "Filaname"() -> (w1056:string)
                                n711 = local read "Filaname"() -> (w1053:string)
                                n712 = Get Date/Time In Seconds() -> (seconds since 1Jan1904=w1039:timestamp)
                                n713 = Format Date/Time String(time format string (%c)="_%Y%m%d_%H%M%S_", seconds (now)=w1039) -> (date/time string=w1037:string)  [unwired: 1 in]
                                n714 = Concatenate Strings("Histo_", w1053, w1037, ".dat") -> (w1052:string)
                                n715 = Concatenate Strings("Tscale_", w1056, w1037, ".dat") -> (w1057:string)
                                n716 = local read "Path"() -> (w1054:path)
                                n717 = local read "Path"() -> (w1055:path)
                                n718 = Build Path(base path=w1054, name or relative path=w1052) -> (appended path=w1040:path)
                                n719 = Build Path(base path=w1055, name or relative path=w1057) -> (appended path=w1041:path)
                                n720 = call-poly <vilib>:"Write Delimited Spreadsheet.vi"("file path (dialog if empty)"=w1040, "1D data"=w1042, "append to file? (new file:F)"=FALSE, "transpose? (no:F)"=TRUE) -> ()  [unwired: 10 in, 2 out]
                                n721 = call-poly <vilib>:"Write Delimited Spreadsheet.vi"("file path (dialog if empty)"=w1041, "1D data"=w1043, "append to file? (new file:F)"=FALSE, "transpose? (no:F)"=TRUE) -> ()  [unwired: 10 in, 2 out]
                                }
                                }
                                n722 = Add Array Elements(numeric array=w1023) -> (sum=w1025:u32)
                                n723 = Divide(x=w1025, y=w1024) -> (x/y=w1022:dbl)
                                }
                                frame "Signal PicoHarp count rate" {
                                n724 = local read "Acc. Threshold (cts)"() -> (w1084:i64)
                                n725 = dll-call lib="F:/Users/Yuriy/Labview/JKU/StreamEye/StreamEye_master_v2_comp2015/PicoHarpLibrary/PHLib.dll" fn="PH_GetCountRate"("devidx"=w1082, "channel"=1, "rate"=0) -> ("rate"=w1081:i32)  [unwired: 6 in, 2 out]
                                n726 = Greater?(x=w1081, y=w1084) -> (0:w1083:bool)
                                n727 = case shown="True" w1083 {
                                tunnel: w1082 -> [_ w1092]
                                tunnel: [w1087 w1089] -> w1080
                                tunnel: w1081 -> [w1087 w1088]
                                frame False {
                                }
                                frame True {
                                n728 = local read "Integration Number (#)"() -> (w1090:i32)
                                n729 = Decrement(x=w1090) -> (x-1=w1093:i32)
                                n730 = for {
                                N: w1093 -> [_]
                                shift-right: [w1096] -> w1091
                                shift-left: w1088 -> [w1097]
                                tunnel: w1092 -> [w1098]
                                stop <- w1094 stop-if-true
                                n731 = local read "Stop Measurement"() -> (w1094:bool)
                                n732 = dll-call lib="F:/Users/Yuriy/Labview/JKU/StreamEye/StreamEye_master_v2_comp2015/PicoHarpLibrary/PHLib.dll" fn="PH_GetCountRate"("devidx"=w1098, "channel"=1, "rate"=0) -> ("rate"=w1095:i32)  [unwired: 6 in, 2 out]
                                n733 = local write "Current Intensity"(w1095) -> ()
                                n734 = local write "Time Trace"(w1095) -> ()
                                n735 = Add(x=w1097, y=w1095) -> (x+y=w1096:i32)
                                }
                                n736 = Divide(x=w1091, y=w1090) -> (x/y=w1089:dbl)
                                }
                                }
                                }
                                }
                              }
                            }
                            n737 = local write "Current Intensity"(w998) -> ()
                            n738 = local write "Time Trace"(w998) -> ()
                            n739 = Replace Array Subset(array=w1002, new element=w998, index (row)=w1004, index (col)=w1003) -> (w1001:dbl[][])
                          }
                          frame True {
                            n740 = local write "Data available Sca"(TRUE ("Data available Sca")) -> ()
                            n741 = property on="Spectrum Graph" class="XYGraph (strict)"() -> ("CrsrList"=w1115:T11)  [unwired: 2 in, 2 out]
                            n742 = control-ref of="Spectrum Graph"() -> (w1122:refnum<vi>)
                            n743 = control-ref of="time elapsed dummy"() -> (w1116:refnum<vi>)
                            n744 = control-ref of="Time Trace"() -> (w1124:refnum<vi>)
                            n745 = control-ref of="single spectrum?"() -> (w1121:refnum<vi>)
                            n746 = control-ref of="Current Intensity"() -> (w1123:refnum<vi>)
                            n747 = local read "Intensity mode selection"() -> (w1114:T2)
                            n748 = local read "Integration Number (#)"() -> (w1104:i32)
                            n749 = for {
                              tunnel: w1115 -> [w1167] mode=indexing
                              tunnel: [w1165] -> _ mode=indexing
                              tunnel: [w1165] -> w1113 mode=indexing
                              n750 = Unbundle(w1167) -> ("Position"=w1166:cluster{"X":dbl, "Y":dbl})  [unwired: 15 out]
                              n751 = Unbundle(w1166) -> ("X"=w1165:dbl)  [unwired: 1 out]
                            }
                            n752 = for {
                              N: w1104 -> [_]
                              tunnel: [w1159] -> w1131
                              tunnel: [w1157] -> w1129
                              tunnel: w1128 -> [w1156]
                              tunnel: w1126 -> [w1154]
                              tunnel: w1124 -> [w1152]
                              tunnel: w1123 -> [w1151]
                              tunnel: w1122 -> [w1150]
                              tunnel: w1121 -> [w1149]
                              tunnel: w1116 -> [w1146]
                              tunnel: w1114 -> [w1145]
                              tunnel: w1113 -> [w1144]
                              tunnel: [w1143] -> w1102 mode=indexing
                              tunnel: [w1142] -> w1107 mode=indexing
                              shift-right: [w1158] -> w1130
                              shift-left: w1127 -> [w1155]
                              shift-right: [w1147] -> w1119
                              shift-left: w1125 -> [w1153]
                              i -> [w1138]
                              stop <- w1134 stop-if-true
                              n753 = call "subVI_get spectrum_master_v1.vi"("writer IN"=w1156, "error writer IN"=w1155, "reader IN"=w1154, "error reader IN"=w1153, "time trace IN"=w1152, "intensity integral IN"=w1151, "Stop IN"=w1149, "reference XY graph IN"=w1150, "Intensity mode selection"=w1145, "reference time elapsed IN"=w1146, "cursors positions"=w1144) -> ("writer OUT"=w1159:refnum<k21>, "error writer OUT"=w1158:errorcluster, "reader OUT"=w1157:refnum<k21>, "error reader OUT"=w1148:errorcluster)  [unwired: 5 in]
                              n754 = flat-sequence {
                                tunnel: w1148 -> [w1164]
                                tunnel: [w1164] -> w1147
                                tunnel: [w1161] -> w1143
                                tunnel: [w1160] -> w1142
                                tunnel: [w1160] -> w1137
                                frame #0 {
                                n755 = local read "Current Intensity"() -> (w1160:dbl)
                                n756 = local read "Spectrum Graph"() -> (w1163:T4)
                                n757 = Unbundle(w1163) -> ("Calibrated Array"=w1162:dbl[], "Array F32"=w1161:sgl[])
                                n758 = local write "Wscale Sca"(w1162) -> ()
                                }
                              }
                              n759 = local read "Acc. Threshold (cts)"() -> (w1140:i64)
                              n760 = local read "Stop Measurement"() -> (w1135:bool)
                              n761 = Less?(x=w1137, y=w1140) -> (x < y?=w1141:bool)
                              n762 = Equal To 0?(x=w1138) -> (x = 0?=w1139:bool)
                              n763 = And(x=w1141, y=w1139) -> (x .and. y?=w1136:bool)
                              n764 = Or(x=w1136, y=w1135) -> (x .or. y?=w1134:bool)
                            }
                            n765 = Add Array Elements(numeric array=w1107) -> (sum=w1108:dbl)
                            n766 = Transpose 2D Array(2D array=w1102) -> (transposed array=w1101:sgl[][])
                            n767 = for {
                              tunnel: w1101 -> [w1133] mode=indexing
                              tunnel: [w1132] -> w1105 mode=indexing
                              n768 = Add Array Elements(numeric array=w1133) -> (sum=w1132:sgl)
                            }
                            n769 = Divide(x=w1108, y=w1104) -> (x/y=w1106:dbl)
                            n770 = Replace Array Subset(array=w1110, new element=w1106, index (row)=w1118, index (col)=w1117) -> (w1109:dbl[][])
                            n771 = Divide(x=w1105, y=w1104) -> (x/y=w1103:sgl[])
                            n772 = Replace Array Subset(array=w1112, new element=w1103, index (dim 0)=w1118, index (dim 1)=w1117) -> (w1111:dbl[][][])  [unwired: 1 in]
                          }
                        }
                      }
                      frame #5 {
                        n773 = local read "time start"() -> (w1170:i32)
                        n774 = Tick Count (ms)() -> (millisecond timer value=w1171:u32)
                        n775 = Subtract(x=w1171, y=w1170) -> (x-y=w1169:u32)
                        n776 = Divide(x=w1169, y=u32 1000) -> (x/y=w1172:dbl)
                        n777 = local write "time elapsed"(w1172) -> ()
                      }
                    }
                    n778 = Increment(x=w893) -> (x+1=w894:i32)
                    n779 = local read "Stop Measurement"() -> (w905:bool)
                    n780 = Equal?(x=w894, y=w917) -> (x = y?=w918:bool)
                    n781 = Or(x=w905, y=w918) -> (x .or. y?=w916:bool)
                    n782 = local write "XYZ Graph Scanner"(w895) -> ()
                  }
                  n783 = Increment(x=w861) -> (x+1=w860:i32)
                  n784 = Equal?(x=w860, y=w866) -> (x = y?=w868:bool)
                  n785 = Or(x=w867, y=w868) -> (x .or. y?=w869:bool)
                }
                n786 = property on="XYZ Graph Scanner" class="IntGraph (strict)"("XScale.Offset"=w823, "XScale.Multiplier"=w828, "XScale.Precision"=u8 1 ("X Scale.Display Format:Precision")) -> ()  [unwired: 2 in, 2 out]
                n787 = property on="XYZ Graph Scanner" class="IntGraph (strict)"("YScale.Offset"=w831, "YScale.Multiplier"=w815, "YScale.Precision"=u8 1 ("Y Scale.Display Format:Precision")) -> ()  [unwired: 2 in, 2 out]
                n788 = local write "XY Array Sca"(w838) -> ()
                n789 = local write "XYZ MegaArray Sca"(w841) -> ()
                n790 = flat-sequence {
                  tunnel: [w1181] -> _
                  tunnel: w848 -> [w1183]
                  tunnel: w847 -> [w1182]
                  tunnel: w849 -> [w1181]
                  tunnel: w846 -> [w1180]
                  frame #0 {
                    n791 = local write "reader endpoint"(w1182) -> ()
                    n792 = local write "error writer"(w1183) -> ()
                    n793 = local write "writer endpoint"(w1181) -> ()
                    n794 = local write "error reader"(w1180) -> ()
                    n795 = local write "Stop Measurement"(FALSE ("Stop Measurement")) -> ()
                  }
                }
              }
              frame 10 {
                # "XW MegaArray"
                # "Y"
                # "X"
                # "Start Hyperspectral Galvos"
                n796 = local read "error reader"() -> (w1216:errorcluster)
                n797 = local read "Yoffset_Gal"() -> (w1209:dbl)
                n798 = local read "Xoffset_Gal"() -> (w1212:dbl)
                n799 = local read "error writer"() -> (w1218:errorcluster)
                n800 = local read "numPixels"() -> (w1184:u16)
                n801 = local read "Ystart_Gal"() -> (w1210:dbl)
                n802 = local read "Xstart_Gal"() -> (w1215:dbl)
                n803 = local read "Yend_Gal"() -> (w1208:dbl)
                n804 = local read "Xend_Gal"() -> (w1213:dbl)
                n805 = local read "Galvo error out Y"() -> (w1200:errorcluster)
                n806 = local read "Galvo error out X"() -> (w1198:errorcluster)
                n807 = local read "Galvo task out Y"() -> (w1201:refnum<k21>)
                n808 = local read "Galvo task out X"() -> (w1199:refnum<k21>)
                n809 = local read "reader endpoint"() -> (w1217:refnum<k21>)
                n810 = local read "writer endpoint"() -> (w1219:refnum<k21>)
                n811 = local read "Steps Hyperspectral Gal"() -> (w1191:u32)
                n812 = Add(x=w1210, y=w1209) -> (x+y=w1207:dbl)
                n813 = Add(x=w1209, y=w1208) -> (x+y=w1206:dbl)
                n814 = Add(x=w1215, y=w1212) -> (x+y=w1214:dbl)
                n815 = Add(x=w1213, y=w1212) -> (x+y=w1211:dbl)
                n816 = call "subVI_RampGenerator.vi"("Number of Positions"=w1191, "End  (um)"=w1206, "Start  (um)"=w1207) -> ("Array"=w1192:dbl[])  [unwired: 1 in]
                n817 = call "subVI_RampGenerator.vi"("Number of Positions"=w1191, "End  (um)"=w1211, "Start  (um)"=w1214) -> ("Array"=w1193:dbl[])  [unwired: 1 in]
                n818 = Initialize Array(0, w1191, w1184) -> (w1190:i32[][])
                n819 = local write "Yscale hyper"(w1192) -> ()
                n820 = local write "Xscale hyper"(w1193) -> ()
                n821 = while {
                  tunnel: w1191 -> [w1260]
                  shift-right: [w1257] -> w1205
                  shift-left: w1219 -> [w1253]
                  shift-right: [w1256] -> w1204
                  shift-left: w1218 -> [w1252]
                  shift-right: [w1255] -> w1203
                  shift-left: w1217 -> [w1251]
                  shift-right: [w1254] -> w1202
                  shift-left: w1216 -> [w1250]
                  tunnel: w1193 -> [w1249]
                  tunnel: w1192 -> [w1248]
                  tunnel: w1201 -> [w1247]
                  tunnel: w1200 -> [w1246]
                  tunnel: w1199 -> [w1245]
                  tunnel: w1198 -> [w1244]
                  tunnel: [w1243] -> w1197
                  tunnel: [w1242] -> w1196
                  tunnel: [w1241] -> w1195
                  tunnel: [w1240] -> w1194
                  shift-right: [w1238] -> w1189
                  shift-left: w1190 -> [w1239]
                  i -> [w1233]
                  stop <- w1258 stop-if-true
                  n822 = flat-sequence {
                    tunnel: w1244 -> [w1263]
                    tunnel: w1245 -> [w1264]
                    tunnel: w1246 -> [w1265]
                    tunnel: w1247 -> [w1266]
                    tunnel: w1248 -> [w1267]
                    tunnel: w1233 -> [w1268]
                    tunnel: w1249 -> [w1269]
                    tunnel: [w1269] -> w1232
                    tunnel: [w1268] -> w1231
                    tunnel: [w1267] -> w1230
                    tunnel: [w1266] -> w1229
                    tunnel: [w1265] -> w1228
                    tunnel: [w1264] -> w1227
                    tunnel: [w1263] -> w1226
                    tunnel: [w1283] -> w1243
                    tunnel: [w1282] -> w1242
                    tunnel: [w1281] -> w1241
                    tunnel: [w1280] -> w1240
                    tunnel: [w1273] -> w1235
                    tunnel: w1232 -> [w1299]
                    tunnel: w1231 -> [w1273]
                    tunnel: w1230 -> [w1298]
                    tunnel: w1229 -> [w1287]
                    tunnel: w1228 -> [w1286]
                    tunnel: w1227 -> [w1285]
                    tunnel: w1226 -> [w1284]
                    tunnel: [w1300] -> w1236
                    tunnel: w1235 -> [w1300]
                    tunnel: [w1307] -> w1237
                    tunnel: w1236 -> [w1307]
                    tunnel: [w1304] -> w1220
                    tunnel: w1253 -> [w1317]
                    tunnel: w1252 -> [w1316]
                    tunnel: w1251 -> [w1315]
                    tunnel: w1250 -> [w1314]
                    tunnel: w1239 -> [w1313]
                    tunnel: w1237 -> [w1311]
                    tunnel: [w1321] -> w1225
                    tunnel: [w1320] -> w1224
                    tunnel: [w1319] -> w1223
                    tunnel: [w1318] -> w1222
                    tunnel: [w1312] -> w1221
                    tunnel: w1220 -> [w1308]
                    tunnel: [w1395] -> w1238
                    tunnel: [w1396] -> w1254
                    tunnel: [w1397] -> w1255
                    tunnel: [w1398] -> w1256
                    tunnel: [w1399] -> w1257
                    tunnel: w1225 -> [w1399]
                    tunnel: w1224 -> [w1398]
                    tunnel: w1223 -> [w1397]
                    tunnel: w1222 -> [w1396]
                    tunnel: w1221 -> [w1395]
                    frame #0 {
                      n823 = Tick Count (ms)() -> (millisecond timer value=w1262:u32)
                      n824 = local write "time start"(w1262) -> ()
                    }
                    frame #1 {
                      # "um to Volts"
                      # "go"
                      n825 = Index Array(array=w1298, index=w1273) -> (element=w1274:dbl)
                      n826 = Index Array(array=w1299, index=w1273) -> (element=w1277:dbl)
                      n827 = call <vilib>:"DAQmx Start Task.vi"("task/channels in"=w1285, "error in"=w1284) -> ("task out"=w1290:refnum<k21>, "error out"=w1293:errorcluster)  [unwired: 12 in]
                      n828 = local read "Yoffset_Gal"() -> (w1275:dbl)
                      n829 = local read "Xoffset_Gal"() -> (w1278:dbl)
                      n830 = local read "G-asym"() -> (w1272:dbl)
                      n831 = local read "G-Scalling (µm/V)"() -> (w1271:dbl)
                      n832 = Subtract(x=w1274, y=w1275) -> (x-y=w1276:dbl)
                      n833 = Subtract(x=w1277, y=w1278) -> (x-y=w1279:dbl)
                      n834 = local write "Yread_Gal"(w1276) -> ()
                      n835 = local write "Xread_Gal"(w1279) -> ()
                      n836 = Multiply(x=w1272, y=w1271) -> (x*y=w1270:dbl)
                      n837 = Divide(x=w1277, y=w1271) -> (x/y=w1289:dbl)
                      n838 = Divide(x=w1274, y=w1270) -> (x/y=w1288:dbl)
                      n839 = call-poly <vilib>:"DAQmx Write.vi"("task/channels in"=w1290, "data"=w1289, "error in"=w1293) -> ("task out"=w1291:refnum<k21>, "error out"=w1292:errorcluster)  [unwired: 10 in, 1 out]
                      n840 = call <vilib>:"DAQmx Start Task.vi"("task/channels in"=w1287, "error in"=w1286) -> ("task out"=w1294:refnum<k21>, "error out"=w1297:errorcluster)  [unwired: 12 in]
                      n841 = call <vilib>:"DAQmx Stop Task.vi"("task/channels in"=w1291, "error in"=w1292) -> ("task out"=w1281:refnum<k21>, "error out"=w1280:errorcluster)  [unwired: 12 in]
                      n842 = call-poly <vilib>:"DAQmx Write.vi"("task/channels in"=w1294, "data"=w1288, "error in"=w1297) -> ("task out"=w1295:refnum<k21>, "error out"=w1296:errorcluster)  [unwired: 10 in, 1 out]
                      n843 = call <vilib>:"DAQmx Stop Task.vi"("task/channels in"=w1295, "error in"=w1296) -> ("task out"=w1282:refnum<k21>, "error out"=w1283:errorcluster)  [unwired: 12 in]
                    }
                    frame #2 {
                      # "wait"
                      n844 = local read "Xdelay_Gal"() -> (w1303:dbl)
                      n845 = Multiply(x=w1303, y=1000.0) -> (x*y=w1301:dbl)
                      n846 = Wait (ms)(milliseconds to wait=w1301) -> ()  [unwired: 1 out]
                    }
                    frame #3 {
                      # "read"
                      n847 = local read "Signal source selection"() -> (w1306:T1)
                      n848 = Equal?(x=w1306, y=T1."Signal Stream" ("Signal source selection")) -> (x = y?=w1304:bool)
                    }
                    frame #4 {
                      # "get spectrum"
                      n849 = local read "Hosts Synchronized"() -> (w1310:bool)
                      n850 = And(x=w1310, y=w1308) -> (x .and. y?=w1309:bool)
                      n851 = case shown="True" w1309 {
                        tunnel: [w1328 w1369] -> w1321
                        tunnel: [w1327 w1368] -> w1320
                        tunnel: [w1326 w1367] -> w1319
                        tunnel: [w1325 w1356] -> w1318
                        tunnel: w1317 -> [w1328 w1366]
                        tunnel: w1316 -> [w1327 w1365]
                        tunnel: w1315 -> [w1326 w1364]
                        tunnel: w1314 -> [w1325 w1363]
                        tunnel: w1313 -> [w1324 w1355]
                        tunnel: [w1324 w1354] -> w1312
                        tunnel: w1311 -> [_ w1353]
                        frame False {
                          n852 = local read "PicoHarp ON"() -> (w1323:bool)
                          n853 = case shown="True" w1323 {
                            tunnel: [w1329 w1331] -> w1322
                            frame False {
                              n854 = Random Number (0-1)() -> (number: 0 to 1=w1329:dbl)
                            }
                            frame True {
                              n855 = local read "PicoHarp handle"() -> (w1330:i32)
                              n856 = local read "Signal source selection"() -> (w1332:T1)
                              n857 = case shown="\"Signal PicoHarp histro\"" w1332 {
                                tunnel: [w1333 w1334 w1339 w1347] -> w1331
                                tunnel: w1330 -> [_ _ w1338 w1348]
                                frame "Signal None", Default {
                                n858 = Random Number (0-1)() -> (number: 0 to 1=w1333:dbl)
                                }
                                frame "Signal Stream" {
                                n859 = Random Number (0-1)() -> (number: 0 to 1=w1334:dbl)
                                }
                                frame "Signal PicoHarp histro" {
                                n860 = local read "Histo Time (s)"() -> (w1337:dbl)
                                n861 = Multiply(x=w1337, y=1000) -> (x*y=w1336:dbl)
                                n862 = To Long Integer(number=w1336) -> (32bit integer=w1335:i32)
                                n863 = call "Start Measurement.vi"("Acquisition time"=w1335, "DeviceIndex"=w1338) -> ("DataValid"=w1341:bool)
                                n864 = case shown="True" w1341 {
                                tunnel: [u32 0 w1344] -> w1339
                                tunnel: w1338 -> [_ w1343]
                                frame False {
                                }
                                frame True {
                                n865 = call "Get Histogram.vi"("DeviceIndex"=w1343) -> ("IntegralCount"=w1344:i32)  [unwired: 1 in, 2 out]
                                }
                                }
                                }
                                frame "Signal PicoHarp count rate" {
                                n866 = dll-call lib="F:/Users/Yuriy/Labview/JKU/StreamEye/StreamEye_master_v2_comp2015/PicoHarpLibrary/PHLib.dll" fn="PH_GetCountRate"("devidx"=w1348, "channel"=1, "rate"=0) -> ("rate"=w1347:i32)  [unwired: 6 in, 2 out]
                                }
                              }
                            }
                          }
                          n867 = local write "Current Intensity"(w1322) -> ()
                          n868 = local write "Time Trace"(w1322) -> ()
                        }
                        frame True {
                          n869 = control-ref of="Spectrum Graph"() -> (w1360:refnum<vi>)
                          n870 = property on="Spectrum Graph" class="XYGraph (strict)"() -> ("CrsrList"=w1351:T11)  [unwired: 2 in, 2 out]
                          n871 = local write "Data available XW"(TRUE ("Data available XW")) -> ()
                          n872 = control-ref of="time elapsed dummy"() -> (w1352:refnum<vi>)
                          n873 = control-ref of="Time Trace"() -> (w1362:refnum<vi>)
                          n874 = local read "Intensity mode selection"() -> (w1350:T2)
                          n875 = control-ref of="single spectrum?"() -> (w1359:refnum<vi>)
                          n876 = control-ref of="Current Intensity"() -> (w1361:refnum<vi>)
                          n877 = for {
                            tunnel: w1351 -> [w1372] mode=indexing
                            tunnel: [w1370] -> w1349 mode=indexing
                            n878 = Unbundle(w1372) -> ("Position"=w1371:cluster{"X":dbl, "Y":dbl})  [unwired: 15 out]
                            n879 = Unbundle(w1371) -> ("X"=w1370:dbl)  [unwired: 1 out]
                          }
                          n880 = call "subVI_get spectrum_master_v1.vi"("writer IN"=w1366, "error writer IN"=w1365, "reader IN"=w1364, "error reader IN"=w1363, "time trace IN"=w1362, "intensity integral IN"=w1361, "Stop IN"=w1359, "reference XY graph IN"=w1360, "Intensity mode selection"=w1350, "reference time elapsed IN"=w1352, "cursors positions"=w1349) -> ("writer OUT"=w1369:refnum<k21>, "error writer OUT"=w1368:errorcluster, "reader OUT"=w1367:refnum<k21>, "error reader OUT"=w1357:errorcluster)  [unwired: 5 in]
                          n881 = flat-sequence {
                            tunnel: [w1389] -> w1354
                            tunnel: w1355 -> [w1388]
                            tunnel: w1353 -> [w1386]
                            tunnel: w1357 -> [w1385]
                            tunnel: [w1385] -> w1356
                            frame #0 {
                              n882 = local read "Spectrum Graph"() -> (w1384:T4)
                              n883 = Unbundle(w1384) -> ("Calibrated Array"=w1378:dbl[], "Array F32"=w1383:sgl[])
                              n884 = local write "Wscale hyper"(w1378) -> ()
                              n885 = Replace Array Subset(array=w1388, new element=w1383, index (row)=w1386) -> (w1389:i32[][])  [unwired: 1 in]
                              n886 = Index Array(array=w1378, index=1) -> (element=w1382:dbl)
                              n887 = Index Array(array=w1378, index=0) -> (element=w1374:dbl)
                              n888 = Subtract(x=w1382, y=w1374) -> (x-y=w1376:dbl)
                              n889 = Transpose 2D Array(2D array=w1389) -> (transposed array=w1387:i32[][])
                              n890 = local write "XYZ hyperspectral graph"(w1387) -> ()
                              n891 = Divide(x=w1376, y=2.0) -> (x/y=w1375:dbl)
                              n892 = Subtract(x=w1374, y=w1375) -> (x-y=w1373:dbl)
                              n893 = property on="XYZ hyperspectral graph" class="IntGraph (strict)"("XScale.Offset"=w1373, "XScale.Multiplier"=w1376, "XScale.Precision"=u8 2 ("X Scale.Display Format:Precision")) -> ()  [unwired: 2 in, 2 out]
                            }
                          }
                        }
                      }
                    }
                    frame #5 {
                      n894 = local read "time start"() -> (w1391:i32)
                      n895 = Tick Count (ms)() -> (millisecond timer value=w1390:u32)
                      n896 = Subtract(x=w1390, y=w1391) -> (x-y=w1392:u32)
                      n897 = Divide(x=w1392, y=u32 1000) -> (x/y=w1394:dbl)
                      n898 = local write "time elapsed"(w1394) -> ()
                    }
                  }
                  n899 = Increment(x=w1233) -> (x+1=w1234:i32)
                  n900 = local read "Stop Measurement"() -> (w1259:bool)
                  n901 = Equal?(x=w1234, y=w1260) -> (x = y?=w1261:bool)
                  n902 = Or(x=w1259, y=w1261) -> (x .or. y?=w1258:bool)
                }
                n903 = property on="XYZ hyperspectral graph" class="IntGraph (strict)"("YScale.Offset"=-0.5 ("Y Scale.Offset and Multiplier:Offset"), "YScale.Multiplier"=1.0 ("Y Scale.Offset and Multiplier:Multiplier"), "YScale.Precision"=u8 0 ("X Scale.Display Format:Precision")) -> ()  [unwired: 2 in, 2 out]
                n904 = local write "XW MegaArray"(w1189) -> ()
                n905 = flat-sequence {
                  tunnel: [w1403] -> _
                  tunnel: [w1402] -> _
                  tunnel: w1203 -> [w1404]
                  tunnel: w1205 -> [w1403]
                  tunnel: w1204 -> [w1402]
                  tunnel: w1202 -> [w1401]
                  frame #0 {
                    n906 = local write "writer endpoint"(w1403) -> ()
                    n907 = local write "error writer"(w1402) -> ()
                    n908 = local write "error reader"(w1401) -> ()
                    n909 = local write "reader endpoint"(w1404) -> ()
                    n910 = local write "Stop Measurement"(FALSE ("Stop Measurement")) -> ()
                  }
                }
                n911 = local write "Galvo task out Y"(w1196) -> ()
                n912 = local write "Galvo error out Y"(w1197) -> ()
                n913 = local write "Galvo task out X"(w1195) -> ()
                n914 = local write "Galvo error out X"(w1194) -> ()
              }
              frame 11 {
                # "XYZ Array"
                # "XYZ MegaArray"
                # "Y"
                # "X"
                # "Start Image Galvos"
                n915 = local read "error reader"() -> (w1460:errorcluster)
                n916 = local read "Yoffset_Gal"() -> (w1456:dbl)
                n917 = local read "Xoffset_Gal"() -> (w1458:dbl)
                n918 = local read "error writer"() -> (w1462:errorcluster)
                n919 = local read "Xsteps_Gal"() -> (w1432:u32)
                n920 = local read "Ysteps_Gal"() -> (w1431:u32)
                n921 = local read "numPixels"() -> (w1405:u16)
                n922 = local read "Ystart_Gal"() -> (w1412:dbl)
                n923 = local read "Xstart_Gal"() -> (w1414:dbl)
                n924 = local read "Ystep_Gal"() -> (w1419:dbl)
                n925 = local read "Xstep_Gal"() -> (w1417:dbl)
                n926 = local read "Yend_Gal"() -> (w1413:dbl)
                n927 = local read "Xend_Gal"() -> (w1415:dbl)
                n928 = local read "Galvo error out Y"() -> (w1452:errorcluster)
                n929 = local read "Galvo error out X"() -> (w1450:errorcluster)
                n930 = local read "Galvo task out Y"() -> (w1451:refnum<k21>)
                n931 = local read "reader endpoint"() -> (w1461:refnum<k21>)
                n932 = local read "Galvo task out X"() -> (w1453:refnum<k21>)
                n933 = local read "writer endpoint"() -> (w1463:refnum<k21>)
                n934 = Subtract(x=w1413, y=w1412) -> ()  [unwired: 1 out]
                n935 = Subtract(x=w1415, y=w1414) -> ()  [unwired: 1 out]
                n936 = Greater?(x=w1413, y=w1412) -> (0:w1420:bool)
                n937 = Add(x=w1456, y=w1413) -> (x+y=w1454:dbl)
                n938 = Add(x=w1414, y=w1458) -> (x+y=w1459:dbl)
                n939 = Greater?(x=w1415, y=w1414) -> (0:w1425:bool)
                n940 = Add(x=w1415, y=w1458) -> (x+y=w1457:dbl)
                n941 = Initialize Array(0.0 ("element"), w1432, w1431, w1405) -> (w1438:dbl[][][])
                n942 = Add(x=w1412, y=w1456) -> (x+y=w1455:dbl)
                n943 = call "subVI_RampGenerator.vi"("Number of Positions"=w1432, "End  (um)"=w1457, "Start  (um)"=w1459) -> ("Array"=w1441:dbl[])  [unwired: 1 in]
                n944 = Divide(x=w1419, y=2.0) -> (x/y=w1408:dbl)
                n945 = Divide(x=w1417, y=2.0) -> (x/y=w1411:dbl)
                n946 = Select(t=1.0, s=w1420, f=-1.0) -> (s? t:f=w1406:dbl)
                n947 = Select(t=1.0, s=w1425, f=-1.0) -> (s? t:f=w1409:dbl)
                n948 = local write "Xscale Gal"(w1441) -> ()
                n949 = Multiply(x=w1408, y=w1406) -> (x*y=w1407:dbl)
                n950 = Multiply(x=w1406, y=w1419) -> (x*y=w1418:dbl)
                n951 = Multiply(x=w1411, y=w1409) -> (x*y=w1410:dbl)
                n952 = Multiply(x=w1409, y=w1417) -> (x*y=w1416:dbl)
                n953 = call "subVI_RampGenerator.vi"("Number of Positions"=w1431, "End  (um)"=w1454, "Start  (um)"=w1455) -> ("Array"=w1440:dbl[])  [unwired: 1 in]
                n954 = local write "Yscale Gal"(w1440) -> ()
                n955 = Subtract(x=w1412, y=w1407) -> (x-y=w1428:dbl)
                n956 = Subtract(x=w1414, y=w1410) -> (x-y=w1426:dbl)
                n957 = Initialize Array(0.0 ("element"), w1432, w1431) -> (w1435:dbl[][])
                n958 = while {
                  tunnel: w1432 -> [w1492]
                  tunnel: w1463 -> [w1491]
                  tunnel: w1461 -> [w1489]
                  tunnel: w1441 -> [w1487]
                  tunnel: w1440 -> [w1486]
                  tunnel: [w1478] -> w1444
                  tunnel: [w1477] -> w1443
                  shift-right: [w1479] -> w1445
                  shift-left: w1462 -> [w1490]
                  shift-right: [w1481] -> w1449
                  shift-left: w1460 -> [w1488]
                  shift-right: [w1465] -> w1448
                  shift-left: w1453 -> [w1485]
                  shift-right: [w1476] -> w1442
                  shift-left: w1452 -> [w1484]
                  shift-right: [w1464] -> w1447
                  shift-left: w1451 -> [w1483]
                  shift-right: [w1480] -> w1446
                  shift-left: w1450 -> [w1482]
                  tunnel: w1431 -> [w1473]
                  shift-right: [w1470] -> w1437
                  shift-left: w1438 -> [w1471]
                  shift-right: [w1468] -> w1434
                  shift-left: w1435 -> [w1469]
                  i -> [w1466]
                  stop <- w1472 stop-if-true
                  n959 = while {
                    tunnel: w1492 -> [w1539]
                    shift-right: [w1537] -> w1477
                    shift-left: w1491 -> [w1533]
                    shift-right: [w1536] -> w1476
                    shift-left: w1490 -> [w1532]
                    shift-right: [w1535] -> w1478
                    shift-left: w1489 -> [w1531]
                    shift-right: [w1534] -> w1479
                    shift-left: w1488 -> [w1530]
                    tunnel: w1487 -> [w1529]
                    tunnel: w1486 -> [w1528]
                    tunnel: w1484 -> [w1526]
                    tunnel: w1482 -> [w1524]
                    tunnel: [w1523] -> w1481
                    tunnel: [w1522] -> w1480
                    tunnel: [w1521] -> w1474
                    tunnel: w1466 -> [w1520]
                    shift-right: [w1517] -> w1470
                    shift-left: w1471 -> [w1518]
                    shift-right: [w1512] -> w1468
                    shift-left: w1469 -> [w1513]
                    shift-right: [w1501] -> w1465
                    shift-left: w1485 -> [w1527]
                    shift-right: [w1500] -> w1464
                    shift-left: w1483 -> [w1525]
                    i -> [w1502]
                    stop <- w1538 stop-if-true
                    n960 = flat-sequence {
                      tunnel: w1520 -> [w1542]
                      tunnel: w1524 -> [w1543]
                      tunnel: w1525 -> [w1544]
                      tunnel: w1526 -> [w1545]
                      tunnel: w1527 -> [w1546]
                      tunnel: w1528 -> [w1547]
                      tunnel: w1502 -> [w1548]
                      tunnel: w1529 -> [w1549]
                      tunnel: [w1549] -> w1511
                      tunnel: [w1548] -> w1510
                      tunnel: [w1547] -> w1509
                      tunnel: [w1546] -> w1508
                      tunnel: [w1545] -> w1507
                      tunnel: [w1544] -> w1506
                      tunnel: [w1543] -> w1505
                      tunnel: [w1542] -> w1504
                      tunnel: [w1568] -> w1523
                      tunnel: [w1567] -> w1500
                      tunnel: [w1566] -> w1522
                      tunnel: [w1563] -> w1519
                      tunnel: [w1556] -> w1514
                      tunnel: w1511 -> [w1578]
                      tunnel: w1510 -> [w1565]
                      tunnel: w1509 -> [w1577]
                      tunnel: w1508 -> [w1572]
                      tunnel: w1507 -> [w1571]
                      tunnel: w1506 -> [w1570]
                      tunnel: w1505 -> [w1569]
                      tunnel: w1504 -> [w1556]
                      tunnel: [w1555] -> w1501
                      tunnel: w1519 -> [w1591]
                      tunnel: [w1590] -> w1515
                      tunnel: w1514 -> [w1590]
                      tunnel: [w1601] -> w1516
                      tunnel: w1515 -> [w1601]
                      tunnel: [w1598] -> w1493
                      tunnel: w1533 -> [w1614]
                      tunnel: w1532 -> [w1613]
                      tunnel: w1531 -> [w1612]
                      tunnel: w1530 -> [w1611]
                      tunnel: w1518 -> [w1610]
                      tunnel: w1502 -> [w1608]
                      tunnel: w1516 -> [w1607]
                      tunnel: w1513 -> [w1606]
                      tunnel: [w1618] -> w1499
                      tunnel: [w1617] -> w1498
                      tunnel: [w1616] -> w1497
                      tunnel: [w1615] -> w1496
                      tunnel: [w1609] -> w1495
                      tunnel: [w1605] -> w1494
                      tunnel: w1493 -> [w1602]
                      tunnel: [w1693] -> w1512
                      tunnel: [w1694] -> w1517
                      tunnel: [w1695] -> w1534
                      tunnel: [w1696] -> w1535
                      tunnel: [w1697] -> w1536
                      tunnel: [w1698] -> w1537
                      tunnel: w1499 -> [w1698]
                      tunnel: w1498 -> [w1697]
                      tunnel: w1497 -> [w1696]
                      tunnel: w1496 -> [w1695]
                      tunnel: w1495 -> [w1694]
                      tunnel: w1494 -> [w1693]
                      frame #0 {
                        n961 = Tick Count (ms)() -> (millisecond timer value=w1541:u32)
                        n962 = local write "time start"(w1541) -> ()
                      }
                      frame #1 {
                        # "um to Volts"
                        # "go"
                        n963 = Index Array(array=w1577, index=w1556) -> (element=w1559:dbl)
                        n964 = Index Array(array=w1578, index=w1565) -> (element=w1562:dbl)
                        n965 = local read "Yoffset_Gal"() -> (w1558:dbl)
                        n966 = local read "Xoffset_Gal"() -> (w1561:dbl)
                        n967 = local read "G-asym"() -> (w1550:dbl)
                        n968 = local read "G-Scalling (µm/V)"() -> (w1551:dbl)
                        n969 = Subtract(x=w1559, y=w1558) -> (x-y=w1557:dbl)
                        n970 = Subtract(x=w1562, y=w1561) -> (x-y=w1560:dbl)
                        n971 = call <vilib>:"DAQmx Start Task.vi"("task/channels in"=w1572, "error in"=w1571) -> ("task out"=w1573:refnum<k21>, "error out"=w1576:errorcluster)  [unwired: 12 in]
                        n972 = local write "Yread_Gal"(w1557) -> ()
                        n973 = local write "Xread_Gal"(w1560) -> ()
                        n974 = Divide(x=w1562, y=w1551) -> (x/y=w1554:dbl)
                        n975 = Multiply(x=w1550, y=w1551) -> (x*y=w1552:dbl)
                        n976 = Divide(x=w1559, y=w1552) -> (x/y=w1553:dbl)
                        n977 = call-poly <vilib>:"DAQmx Write.vi"("task/channels in"=w1573, "data"=w1554, "error in"=w1576) -> ("task out"=w1574:refnum<k21>, "error out"=w1575:errorcluster)  [unwired: 10 in, 1 out]
                        n978 = Equal?(x=w1565, y=0) -> (x = y?=w1563:bool)
                        n979 = case shown="True" w1563 {
                          tunnel: w1553 -> [_ w1585]
                          tunnel: w1570 -> [w1580 w1584]
                          tunnel: w1569 -> [w1579 w1583]
                          tunnel: [w1580 w1582] -> w1567
                          tunnel: [w1579 w1581] -> w1566
                          frame False {
                          }
                          frame True {
                            n980 = call <vilib>:"DAQmx Start Task.vi"("task/channels in"=w1584, "error in"=w1583) -> ("task out"=w1586:refnum<k21>, "error out"=w1589:errorcluster)  [unwired: 12 in]
                            n981 = call-poly <vilib>:"DAQmx Write.vi"("task/channels in"=w1586, "data"=w1585, "error in"=w1589) -> ("task out"=w1587:refnum<k21>, "error out"=w1588:errorcluster)  [unwired: 10 in, 1 out]
                            n982 = call <vilib>:"DAQmx Stop Task.vi"("task/channels in"=w1587, "error in"=w1588) -> ("task out"=w1582:refnum<k21>, "error out"=w1581:errorcluster)  [unwired: 12 in]
                          }
                        }
                        n983 = call <vilib>:"DAQmx Stop Task.vi"("task/channels in"=w1574, "error in"=w1575) -> ("task out"=w1555:refnum<k21>, "error out"=w1568:errorcluster)  [unwired: 12 in]
                      }
                      frame #2 {
                        # "wait"
                        n984 = case shown="True" w1591 {
                          frame False {
                          }
                          frame True {
                            # "first in the line"
                            n985 = local read "Ydelay_Gal"() -> (w1595:dbl)
                            n986 = Multiply(x=w1595, y=1000.0) -> (x*y=w1597:dbl)
                            n987 = Wait (ms)(milliseconds to wait=w1597) -> ()  [unwired: 1 out]
                          }
                        }
                        n988 = local read "Xdelay_Gal"() -> (w1594:dbl)
                        n989 = Multiply(x=w1594, y=1000.0) -> (x*y=w1592:dbl)
                        n990 = Wait (ms)(milliseconds to wait=w1592) -> ()  [unwired: 1 out]
                      }
                      frame #3 {
                        # "read"
                        n991 = local read "Signal source selection"() -> (w1600:T1)
                        n992 = Equal?(x=w1600, y=T1."Signal Stream" ("Signal source selection")) -> (x = y?=w1598:bool)
                      }
                      frame #4 {
                        # "get spectrum"
                        n993 = local read "Hosts Synchronized"() -> (w1604:bool)
                        n994 = And(x=w1604, y=w1602) -> (x .and. y?=w1603:bool)
                        n995 = case shown="True" w1603 {
                          tunnel: [w1629 w1673] -> w1618
                          tunnel: [w1628 w1672] -> w1617
                          tunnel: [w1627 w1671] -> w1616
                          tunnel: [w1626 w1660] -> w1615
                          tunnel: w1614 -> [w1629 w1670]
                          tunnel: w1613 -> [w1628 w1669]
                          tunnel: w1612 -> [w1627 w1668]
                          tunnel: w1611 -> [w1626 w1667]
                          tunnel: w1610 -> [w1625 w1659]
                          tunnel: [w1625 w1658] -> w1609
                          tunnel: w1608 -> [w1623 w1657]
                          tunnel: w1607 -> [w1624 w1656]
                          tunnel: w1606 -> [w1622 w1655]
                          tunnel: [w1621 w1654] -> w1605
                          frame False {
                            n996 = local read "PicoHarp ON"() -> (w1620:bool)
                            n997 = case shown="True" w1620 {
                              tunnel: [w1630 w1632] -> w1619
                              frame False {
                                n998 = Random Number (0-1)() -> (number: 0 to 1=w1630:dbl)
                              }
                              frame True {
                                n999 = local read "PicoHarp handle"() -> (w1631:i32)
                                n1000 = local read "Signal source selection"() -> (w1633:T1)
                                n1001 = case shown="\"Signal PicoHarp count rate\"" w1633 {
                                tunnel: [w1634 w1635 w1640 w1648] -> w1632
                                tunnel: w1631 -> [_ _ w1639 w1649]
                                frame "Signal None", Default {
                                n1002 = Random Number (0-1)() -> (number: 0 to 1=w1634:dbl)
                                }
                                frame "Signal Stream" {
                                n1003 = Random Number (0-1)() -> (number: 0 to 1=w1635:dbl)
                                }
                                frame "Signal PicoHarp histro" {
                                n1004 = local read "Histo Time (s)"() -> (w1638:dbl)
                                n1005 = Multiply(x=w1638, y=1000) -> (x*y=w1637:dbl)
                                n1006 = To Long Integer(number=w1637) -> (32bit integer=w1636:i32)
                                n1007 = call "Start Measurement.vi"("Acquisition time"=w1636, "DeviceIndex"=w1639) -> ("DataValid"=w1642:bool)
                                n1008 = case shown="False" w1642 {
                                tunnel: [u32 0 w1645] -> w1640
                                tunnel: w1639 -> [_ w1644]
                                frame False {
                                }
                                frame True {
                                n1009 = call "Get Histogram.vi"("DeviceIndex"=w1644) -> ("IntegralCount"=w1645:i32)  [unwired: 1 in, 2 out]
                                }
                                }
                                }
                                frame "Signal PicoHarp count rate" {
                                n1010 = dll-call lib="F:/Users/Yuriy/Labview/JKU/StreamEye/StreamEye_master_v2_comp2015/PicoHarpLibrary/PHLib.dll" fn="PH_GetCountRate"("devidx"=w1649, "channel"=1, "rate"=0) -> ("rate"=w1648:i32)  [unwired: 6 in, 2 out]
                                }
                                }
                              }
                            }
                            n1011 = local write "Current Intensity"(w1619) -> ()
                            n1012 = local write "Time Trace"(w1619) -> ()
                            n1013 = Replace Array Subset(array=w1622, new element=w1619, index (row)=w1623, index (col)=w1624) -> (w1621:dbl[][])
                          }
                          frame True {
                            n1014 = local write "Data available Gal"(TRUE ("Data available Gal")) -> ()
                            n1015 = property on="Spectrum Graph" class="XYGraph (strict)"() -> ("CrsrList"=w1652:T11)  [unwired: 2 in, 2 out]
                            n1016 = control-ref of="Spectrum Graph"() -> (w1664:refnum<vi>)
                            n1017 = control-ref of="time elapsed dummy"() -> (w1653:refnum<vi>)
                            n1018 = control-ref of="Time Trace"() -> (w1666:refnum<vi>)
                            n1019 = control-ref of="single spectrum?"() -> (w1663:refnum<vi>)
                            n1020 = control-ref of="Current Intensity"() -> (w1665:refnum<vi>)
                            n1021 = local read "Intensity mode selection"() -> (w1651:T2)
                            n1022 = for {
                              tunnel: w1652 -> [w1676] mode=indexing
                              tunnel: [w1674] -> _ mode=indexing
                              tunnel: [w1674] -> w1650 mode=indexing
                              n1023 = Unbundle(w1676) -> ("Position"=w1675:cluster{"X":dbl, "Y":dbl})  [unwired: 15 out]
                              n1024 = Unbundle(w1675) -> ("X"=w1674:dbl)  [unwired: 1 out]
                            }
                            n1025 = call "subVI_get spectrum_master_v1.vi"("writer IN"=w1670, "error writer IN"=w1669, "reader IN"=w1668, "error reader IN"=w1667, "time trace IN"=w1666, "intensity integral IN"=w1665, "Stop IN"=w1663, "reference XY graph IN"=w1664, "Intensity mode selection"=w1651, "reference time elapsed IN"=w1653, "cursors positions"=w1650) -> ("writer OUT"=w1673:refnum<k21>, "error writer OUT"=w1672:errorcluster, "reader OUT"=w1671:refnum<k21>, "error reader OUT"=w1661:errorcluster)  [unwired: 5 in]
                            n1026 = flat-sequence {
                              tunnel: w1661 -> [w1687]
                              tunnel: [w1687] -> w1660
                              tunnel: w1659 -> [w1684]
                              tunnel: [w1683] -> w1658
                              tunnel: w1657 -> [w1677]
                              tunnel: w1656 -> [w1678]
                              tunnel: w1655 -> [w1682]
                              tunnel: [w1680] -> w1654
                              frame #0 {
                                n1027 = local read "Current Intensity"() -> (w1681:dbl)
                                n1028 = local read "Spectrum Graph"() -> (w1686:T4)
                                n1029 = Replace Array Subset(array=w1682, new element=w1681, index (row)=w1677, index (col)=w1678) -> (w1680:dbl[][])
                                n1030 = Unbundle(w1686) -> ("Calibrated Array"=w1679:dbl[], "Array F32"=w1685:sgl[])
                                n1031 = local write "Wscale Gal"(w1679) -> ()
                                n1032 = Replace Array Subset(array=w1684, new element=w1685, index (dim 0)=w1677, index (dim 1)=w1678) -> (w1683:dbl[][][])  [unwired: 1 in]
                              }
                            }
                          }
                        }
                      }
                      frame #5 {
                        n1033 = local read "time start"() -> (w1689:i32)
                        n1034 = Tick Count (ms)() -> (millisecond timer value=w1688:u32)
                        n1035 = Subtract(x=w1688, y=w1689) -> (x-y=w1690:u32)
                        n1036 = Divide(x=w1690, y=u32 1000) -> (x/y=w1692:dbl)
                        n1037 = local write "time elapsed"(w1692) -> ()
                      }
                    }
                    n1038 = Increment(x=w1502) -> (x+1=w1503:i32)
                    n1039 = local read "Stop Measurement"() -> (w1521:bool)
                    n1040 = Equal?(x=w1503, y=w1539) -> (x = y?=w1540:bool)
                    n1041 = Or(x=w1521, y=w1540) -> (x .or. y?=w1538:bool)
                    n1042 = local write "XYZ Graph Galvos"(w1512) -> ()
                  }
                  n1043 = Increment(x=w1466) -> (x+1=w1467:i32)
                  n1044 = Equal?(x=w1473, y=w1467) -> (x = y?=w1475:bool)
                  n1045 = Or(x=w1474, y=w1475) -> (x .or. y?=w1472:bool)
                }
                n1046 = property on="XYZ Graph Galvos" class="IntGraph (strict)"("YScale.Offset"=w1428, "YScale.Multiplier"=w1418, "YScale.Precision"=u8 1 ("X Scale.Display Format:Precision")) -> ()  [unwired: 2 in, 2 out]
                n1047 = property on="XYZ Graph Galvos" class="IntGraph (strict)"("XScale.Offset"=w1426, "XScale.Multiplier"=w1416, "XScale.Precision"=u8 1 ("X Scale.Display Format:Precision")) -> ()  [unwired: 2 in, 2 out]
                n1048 = local write "Galvo error out Y"(w1449) -> ()
                n1049 = flat-sequence {
                  tunnel: w1443 -> [w1703]
                  tunnel: w1442 -> [w1702]
                  tunnel: w1444 -> [w1701]
                  tunnel: w1445 -> [w1700]
                  frame #0 {
                    n1050 = local write "writer endpoint"(w1703) -> ()
                    n1051 = local write "error writer"(w1702) -> ()
                    n1052 = local write "error reader"(w1700) -> ()
                    n1053 = local write "reader endpoint"(w1701) -> ()
                    n1054 = local write "Stop Measurement"(FALSE ("Stop Measurement")) -> ()
                  }
                }
                n1055 = local write "XY Array Gal"(w1434) -> ()
                n1056 = local write "XYZ MegaArray Gal"(w1437) -> ()
                n1057 = local write "Galvo task out Y"(w1447) -> ()
                n1058 = local write "Galvo error out X"(w1446) -> ()
                n1059 = local write "Galvo task out X"(w1448) -> ()
              }
              frame 12 {
                # "Start Cursor XY gal"
                n1060 = local read "error reader"() -> (w1716:errorcluster)
                n1061 = local read "error writer"() -> (w1718:errorcluster)
                n1062 = local read "Galvo error out Y"() -> (w1714:errorcluster)
                n1063 = local read "Galvo error out X"() -> (w1712:errorcluster)
                n1064 = local read "Galvo task out Y"() -> (w1715:refnum<k21>)
                n1065 = local read "Galvo task out X"() -> (w1713:refnum<k21>)
                n1066 = local read "reader endpoint"() -> (w1717:refnum<k21>)
                n1067 = local read "writer endpoint"() -> (w1719:refnum<k21>)
                n1068 = while {
                  shift-right: [w1737] -> w1707
                  shift-left: w1719 -> [w1733]
                  shift-right: [w1736] -> w1704
                  shift-left: w1718 -> [w1732]
                  shift-right: [w1735] -> w1705
                  shift-left: w1717 -> [w1731]
                  shift-right: [w1734] -> w1706
                  shift-left: w1716 -> [w1730]
                  tunnel: w1715 -> [w1729]
                  tunnel: w1714 -> [w1728]
                  tunnel: w1713 -> [w1727]
                  tunnel: w1712 -> [w1726]
                  tunnel: [w1725] -> w1708
                  tunnel: [w1724] -> w1711
                  tunnel: [w1723] -> w1710
                  tunnel: [w1722] -> w1709
                  stop <- w1721 stop-if-true
                  n1069 = flat-sequence {
                    tunnel: w1729 -> [w1754]
                    tunnel: w1728 -> [w1753]
                    tunnel: w1727 -> [w1752]
                    tunnel: w1726 -> [w1751]
                    tunnel: [w1750] -> w1725
                    tunnel: [w1749] -> w1724
                    tunnel: [w1748] -> w1723
                    tunnel: [w1747] -> w1722
                    tunnel: [w1766] -> w1720
                    tunnel: [w1779] -> w1737
                    tunnel: [w1778] -> w1736
                    tunnel: [w1777] -> w1735
                    tunnel: [w1776] -> w1734
                    tunnel: w1733 -> [w1775]
                    tunnel: w1732 -> [w1774]
                    tunnel: w1731 -> [w1773]
                    tunnel: w1730 -> [w1772]
                    tunnel: w1720 -> [w1769]
                    frame #0 {
                      # "um to Volts"
                      # "go"
                      n1070 = call <vilib>:"DAQmx Start Task.vi"("task/channels in"=w1754, "error in"=w1753) -> ("task out"=w1761:refnum<k21>, "error out"=w1764:errorcluster)  [unwired: 12 in]
                      n1071 = local read "Yoffset_Gal"() -> (w1743:dbl)
                      n1072 = local read "Xoffset_Gal"() -> (w1746:dbl)
                      n1073 = local read "G-asym"() -> (w1738:dbl)
                      n1074 = local read "G-Scalling (µm/V)"() -> (w1739:dbl)
                      n1075 = property on="XYZ Graph Galvos" class="IntGraph (strict)"() -> ("Cursor.Cursor X"=w1745:dbl)  [unwired: 2 in, 2 out]
                      n1076 = property on="XYZ Graph Galvos" class="IntGraph (strict)"() -> ("Cursor.Cursor Y"=w1742:dbl)  [unwired: 2 in, 2 out]
                      n1077 = local write "Xread_Gal"(w1745) -> ()
                      n1078 = local write "Yread_Gal"(w1742) -> ()
                      n1079 = Multiply(x=w1739, y=w1738) -> (x*y=w1740:dbl)
                      n1080 = Add(x=w1742, y=w1743) -> (x+y=w1741:dbl)
                      n1081 = Add(x=w1746, y=w1745) -> (x+y=w1744:dbl)
                      n1082 = Divide(x=w1741, y=w1740) -> (x/y=w1755:dbl)
                      n1083 = Divide(x=w1744, y=w1739) -> (x/y=w1756:dbl)
                      n1084 = call <vilib>:"DAQmx Start Task.vi"("task/channels in"=w1752, "error in"=w1751) -> ("task out"=w1757:refnum<k21>, "error out"=w1760:errorcluster)  [unwired: 12 in]
                      n1085 = call-poly <vilib>:"DAQmx Write.vi"("task/channels in"=w1761, "data"=w1755, "error in"=w1764) -> ("task out"=w1762:refnum<k21>, "error out"=w1763:errorcluster)  [unwired: 10 in, 1 out]
                      n1086 = call-poly <vilib>:"DAQmx Write.vi"("task/channels in"=w1757, "data"=w1756, "error in"=w1760) -> ("task out"=w1758:refnum<k21>, "error out"=w1759:errorcluster)  [unwired: 10 in, 1 out]
                      n1087 = call <vilib>:"DAQmx Stop Task.vi"("task/channels in"=w1762, "error in"=w1763) -> ("task out"=w1749:refnum<k21>, "error out"=w1750:errorcluster)  [unwired: 12 in]
                      n1088 = call <vilib>:"DAQmx Stop Task.vi"("task/channels in"=w1758, "error in"=w1759) -> ("task out"=w1748:refnum<k21>, "error out"=w1747:errorcluster)  [unwired: 12 in]
                    }
                    frame #1 {
                      # "wait"
                      n1089 = Wait (ms)(milliseconds to wait=100.0 ("y")) -> ()  [unwired: 1 out]
                    }
                    frame #2 {
                      # "read"
                      n1090 = local read "Signal source selection"() -> (w1768:T1)
                      n1091 = Equal?(x=w1768, y=T1."Signal Stream" ("Signal source selection")) -> (x = y?=w1766:bool)
                    }
                    frame #3 {
                      # "get spectrum"
                      n1092 = local read "Hosts Synchronized"() -> (w1771:bool)
                      n1093 = And(x=w1771, y=w1769) -> (x .and. y?=w1770:bool)
                      n1094 = case shown="True" w1770 {
                        tunnel: [w1785 w1821] -> w1779
                        tunnel: [w1784 w1820] -> w1778
                        tunnel: [w1783 w1819] -> w1777
                        tunnel: [w1782 w1818] -> w1776
                        tunnel: w1775 -> [w1785 w1817]
                        tunnel: w1774 -> [w1784 w1816]
                        tunnel: w1773 -> [w1783 w1815]
                        tunnel: w1772 -> [w1782 w1814]
                        frame False {
                          n1095 = local read "PicoHarp ON"() -> (w1781:bool)
                          n1096 = case shown="True" w1781 {
                            tunnel: [w1786 w1788] -> w1780
                            frame False {
                              n1097 = Random Number (0-1)() -> (number: 0 to 1=w1786:dbl)
                            }
                            frame True {
                              n1098 = local read "PicoHarp handle"() -> (w1787:i32)
                              n1099 = local read "Signal source selection"() -> (w1789:T1)
                              n1100 = case shown="\"Signal PicoHarp histro\"" w1789 {
                                tunnel: [w1790 w1791 w1796 w1804] -> w1788
                                tunnel: w1787 -> [_ _ w1795 w1805]
                                frame "Signal None", Default {
                                n1101 = Random Number (0-1)() -> (number: 0 to 1=w1790:dbl)
                                }
                                frame "Signal Stream" {
                                n1102 = Random Number (0-1)() -> (number: 0 to 1=w1791:dbl)
                                }
                                frame "Signal PicoHarp histro" {
                                n1103 = local read "Histo Time (s)"() -> (w1794:dbl)
                                n1104 = Multiply(x=w1794, y=1000) -> (x*y=w1793:dbl)
                                n1105 = To Long Integer(number=w1793) -> (32bit integer=w1792:i32)
                                n1106 = call "Start Measurement.vi"("Acquisition time"=w1792, "DeviceIndex"=w1795) -> ("DataValid"=w1798:bool)
                                n1107 = case shown="False" w1798 {
                                tunnel: [u32 0 w1801] -> w1796
                                tunnel: w1795 -> [_ w1800]
                                frame False {
                                }
                                frame True {
                                n1108 = call "Get Histogram.vi"("DeviceIndex"=w1800) -> ("IntegralCount"=w1801:i32)  [unwired: 1 in, 2 out]
                                }
                                }
                                }
                                frame "Signal PicoHarp count rate" {
                                n1109 = dll-call lib="F:/Users/Yuriy/Labview/JKU/StreamEye/StreamEye_master_v2_comp2015/PicoHarpLibrary/PHLib.dll" fn="PH_GetCountRate"("devidx"=w1805, "channel"=1, "rate"=0) -> ("rate"=w1804:i32)  [unwired: 6 in, 2 out]
                                }
                              }
                            }
                          }
                          n1110 = local write "Current Intensity"(w1780) -> ()
                          n1111 = local write "Time Trace"(w1780) -> ()
                        }
                        frame True {
                          n1112 = property on="Spectrum Graph" class="XYGraph (strict)"() -> ("CrsrList"=w1808:T11)  [unwired: 2 in, 2 out]
                          n1113 = control-ref of="Spectrum Graph"() -> (w1811:refnum<vi>)
                          n1114 = control-ref of="time elapsed"() -> (w1809:refnum<vi>)
                          n1115 = control-ref of="Time Trace"() -> (w1813:refnum<vi>)
                          n1116 = control-ref of="single spectrum?"() -> (w1810:refnum<vi>)
                          n1117 = control-ref of="Current Intensity"() -> (w1812:refnum<vi>)
                          n1118 = local read "Intensity mode selection"() -> (w1807:T2)
                          n1119 = for {
                            tunnel: w1808 -> [w1824] mode=indexing
                            tunnel: [w1822] -> w1806 mode=indexing
                            n1120 = Unbundle(w1824) -> ("Position"=w1823:cluster{"X":dbl, "Y":dbl})  [unwired: 15 out]
                            n1121 = Unbundle(w1823) -> ("X"=w1822:dbl)  [unwired: 1 out]
                          }
                          n1122 = call "subVI_get spectrum_master_v1.vi"("writer IN"=w1817, "error writer IN"=w1816, "reader IN"=w1815, "error reader IN"=w1814, "time trace IN"=w1813, "intensity integral IN"=w1812, "Stop IN"=w1810, "reference XY graph IN"=w1811, "Intensity mode selection"=w1807, "reference time elapsed IN"=w1809, "cursors positions"=w1806) -> ("writer OUT"=w1821:refnum<k21>, "error writer OUT"=w1820:errorcluster, "reader OUT"=w1819:refnum<k21>, "error reader OUT"=w1818:errorcluster)  [unwired: 5 in]
                        }
                      }
                    }
                  }
                  n1123 = local read "Stop Measurement"() -> (w1721:bool)
                }
                n1124 = flat-sequence {
                  tunnel: w1707 -> [w1829]
                  tunnel: w1704 -> [w1828]
                  tunnel: w1705 -> [w1827]
                  tunnel: w1706 -> [w1826]
                  frame #0 {
                    n1125 = local write "error reader"(w1826) -> ()
                    n1126 = local write "writer endpoint"(w1829) -> ()
                    n1127 = local write "reader endpoint"(w1827) -> ()
                    n1128 = local write "error writer"(w1828) -> ()
                    n1129 = local write "Stop Measurement"(FALSE ("Stop Cursor")) -> ()
                  }
                }
                n1130 = local write "Galvo task out Y"(w1711) -> ()
                n1131 = local write "Galvo error out Y"(w1708) -> ()
                n1132 = local write "Galvo task out X"(w1710) -> ()
                n1133 = local write "Galvo error out X"(w1709) -> ()
              }
              frame 13 {
                # "Y values (abs)"
                # "X values (abs)"
                # "Start Cursors Pair XY"
                n1134 = flat-sequence {
                  tunnel: w1849 -> [w1871]
                  tunnel: w1850 -> [w1870]
                  tunnel: w1832 -> [w1869]
                  tunnel: w1833 -> [w1868]
                  frame #0 {
                    n1135 = local write "busy"(TRUE ("busy")) -> ()
                    n1136 = local read "Wscale Gal"() -> (w1858:dbl[])
                    n1137 = local write "Wscale hyper"(w1858) -> ()
                    n1138 = Index Array(array=w1858, index=0) -> (element=w1862:dbl)
                    n1139 = Index Array(array=w1858, index=1) -> (element=w1863:dbl)
                    n1140 = Subtract(x=w1863, y=w1862) -> (x-y=w1864:dbl)
                    n1141 = property on="XYZ hyperspectral graph" class="IntGraph (strict)"("XScale.Offset"=w1862, "XScale.Multiplier"=w1864, "XScale.Precision"=u8 2 ("X Scale.Display Format:Precision")) -> ()  [unwired: 2 in, 2 out]
                  }
                  frame #1 {
                    n1142 = for {
                      N: w1871 -> [_]
                      shift-right: [w1881] -> w1866
                      shift-left: w1870 -> [w1880]
                      tunnel: w1869 -> [w1876] mode=indexing
                      tunnel: w1868 -> [w1874] mode=indexing
                      i -> [w1872]
                      n1143 = local read "Xscale Gal"() -> (w1877:dbl[])
                      n1144 = local read "Yscale Gal"() -> (w1875:dbl[])
                      n1145 = local read "XYZ MegaArray Gal"() -> (w1882:i32[][][])
                      n1146 = call "subVI_GetNearestElement.vi"("element value"=w1876, "input array"=w1877) -> ("index"=w1878:u32)  [unwired: 9 in]
                      n1147 = call "subVI_GetNearestElement.vi"("element value"=w1874, "input array"=w1875) -> ("index"=w1873:u32)  [unwired: 9 in]
                      n1148 = Index Array(array=w1882, index (dim 0)=w1878, index (dim 1)=w1873) -> (element=w1879:i32[])  [unwired: 1 in]
                      n1149 = Replace Array Subset(array=w1880, new element=w1879, index (row)=w1872) -> (w1881:i32[][])  [unwired: 1 in]
                    }
                    n1150 = local write "XW MegaArray"(w1866) -> ()
                    n1151 = Transpose 2D Array(2D array=w1866) -> (transposed array=w1867:i32[][])
                    n1152 = local write "XYZ hyperspectral graph"(w1867) -> ()
                  }
                  frame #2 {
                    n1153 = local write "busy"(FALSE ("busy")) -> ()
                    n1154 = local write "Data available XW"(TRUE ("Data available XW")) -> ()
                  }
                }
                n1155 = local read "Xoffset_Gal"() -> (w1839:dbl)
                n1156 = local read "Yoffset_Gal"() -> (w1836:dbl)
                n1157 = local read "numPixels"() -> (w1830:u16)
                n1158 = property on="XYZ Graph Galvos" class="IntGraph (strict)"() -> ("CrsrLis"=w1848:T11)  [unwired: 2 in, 2 out]
                n1159 = local read "Steps Hyperspectral Gal"() -> (w1849:u32)
                n1160 = for {
                  tunnel: w1848 -> [w1857] mode=indexing
                  tunnel: [w1855] -> w1838 mode=indexing
                  tunnel: [w1854] -> w1835 mode=indexing
                  n1161 = Unbundle(w1857) -> ("Position"=w1856:cluster{"X":dbl, "Y":dbl})  [unwired: 15 out]
                  n1162 = Unbundle(w1856) -> ("X"=w1855:dbl, "Y"=w1854:dbl)
                }
                n1163 = property on="XYZ hyperspectral graph" class="IntGraph (strict)"("YScale.Offset"=0.0 ("Y Scale.Offset and Multiplier:Offset"), "YScale.Multiplier"=1.0 ("Y Scale.Offset and Multiplier:Multiplier"), "YScale.Precision"=u8 0 ("X Scale.Display Format:Precision")) -> ()  [unwired: 2 in, 2 out]
                n1164 = Add(x=w1839, y=w1838) -> (x+y=w1837:dbl[])
                n1165 = Add(x=w1835, y=w1836) -> (x+y=w1834:dbl[])
                n1166 = Index Array(array=w1837, index=0) -> (element=w1843:dbl)
                n1167 = Index Array(array=w1837, index=1) -> (element=w1842:dbl)
                n1168 = Index Array(array=w1834, index=0) -> (element=w1841:dbl)
                n1169 = Index Array(array=w1834, index=1) -> (element=w1840:dbl)
                n1170 = call "subVI_RampGenerator.vi"("Number of Positions"=w1849, "End  (um)"=w1840, "Start  (um)"=w1841) -> ("Array"=w1833:dbl[])  [unwired: 1 in]
                n1171 = call "subVI_RampGenerator.vi"("Number of Positions"=w1849, "End  (um)"=w1842, "Start  (um)"=w1843) -> ("Array"=w1832:dbl[])  [unwired: 1 in]
                n1172 = local write "Xscale hyper"(w1832) -> ()
                n1173 = Initialize Array(0, w1849, w1830) -> (w1850:i32[][])
              }
              frame 17 {
                # "Start Cursor XY scanner"
                n1174 = local read "error reader"() -> (w1889:errorcluster)
                n1175 = local read "error writer"() -> (w1891:errorcluster)
                n1176 = local read "reader endpoint"() -> (w1890:refnum<k21>)
                n1177 = local read "writer endpoint"() -> (w1892:refnum<k21>)
                n1178 = while {
                  shift-right: [w1902] -> w1888
                  shift-left: w1892 -> [w1898]
                  shift-right: [w1901] -> w1885
                  shift-left: w1891 -> [w1897]
                  shift-right: [w1900] -> w1886
                  shift-left: w1890 -> [w1896]
                  shift-right: [w1899] -> w1887
                  shift-left: w1889 -> [w1895]
                  stop <- w1894 stop-if-true
                  n1179 = flat-sequence {
                    tunnel: [w1918] -> w1893
                    tunnel: [w1944] -> w1902
                    tunnel: [w1943] -> w1901
                    tunnel: [w1942] -> w1900
                    tunnel: [w1941] -> w1899
                    tunnel: w1898 -> [w1940]
                    tunnel: w1897 -> [w1939]
                    tunnel: w1896 -> [w1938]
                    tunnel: w1895 -> [w1937]
                    tunnel: w1893 -> [w1934]
                    frame #0 {
                      # "um to mm"
                      n1180 = local read "Xoffset_Sca"() -> (w1910:dbl)
                      n1181 = local read "Yoffset_Sca"() -> (w1911:dbl)
                      n1182 = local read "Wait Scan."() -> (w1903:bool)
                      n1183 = local read "Scanner error out"() -> (w1916:errorcluster)
                      n1184 = property on="XYZ Graph Scanner" class="IntGraph (strict)"() -> ("Cursor.Cursor X"=w1905:dbl)  [unwired: 2 in, 2 out]
                      n1185 = property on="XYZ Graph Scanner" class="IntGraph (strict)"() -> ("Cursor.Cursor Y"=w1904:dbl)  [unwired: 2 in, 2 out]
                      n1186 = Add(x=w1911, y=w1904) -> (x+y=w1913:dbl)
                      n1187 = Add(x=w1910, y=w1905) -> (x+y=w1915:dbl)
                      n1188 = Divide(x=w1913, y=1000.0) -> (x/y=w1908:dbl)
                      n1189 = Divide(x=w1915, y=1000.0) -> (x/y=w1909:dbl)
                      n1190 = Build Array(w1909, w1908) -> (w1907:dbl[])
                      n1191 = call "SMC_MoveAbs.vi"("error in (no error)"=w1916, "WaitUntilReady"=w1903, "Input Array"=w1907) -> ("error out"=w1906:errorcluster)  [unwired: 8 in]
                      n1192 = local write "Scanner error out"(w1906) -> ()
                    }
                    frame #1 {
                      # "wait"
                      n1193 = Wait (ms)(milliseconds to wait=100.0 ("y")) -> ()  [unwired: 1 out]
                    }
                    frame #2 {
                      # "read"
                      n1194 = local read "Xoffset_Sca"() -> (w1927:dbl)
                      n1195 = local read "Yoffset_Sca"() -> (w1924:dbl)
                      n1196 = global read "glb_pos.vi" "Position"() -> (w1929:dbl[])
                      n1197 = local read "Signal source selection"() -> (w1920:T1)
                      n1198 = Index Array(array=w1929, index #1=0 ("index"), index #2=1 ("index")) -> (element #1=w1925:dbl, element #2=w1921:dbl)
                      n1199 = Multiply(x=w1925, y=1000.0) -> (x*y=w1928:dbl)
                      n1200 = Multiply(x=w1921, y=1000.0) -> (x*y=w1923:dbl)
                      n1201 = Equal?(x=w1920, y=T1."Signal Stream" ("Signal source selection")) -> (x = y?=w1918:bool)
                      n1202 = Subtract(x=w1928, y=w1927) -> (x-y=w1926:dbl)
                      n1203 = Subtract(x=w1923, y=w1924) -> (x-y=w1922:dbl)
                      n1204 = local write "Xread_Sca"(w1926) -> ()
                      n1205 = local write "Yread_Sca"(w1922) -> ()
                    }
                    frame #3 {
                      # "get spectrum"
                      n1206 = local read "Hosts Synchronized"() -> (w1936:bool)
                      n1207 = And(x=w1936, y=w1934) -> (x .and. y?=w1935:bool)
                      n1208 = case shown="False" w1935 {
                        tunnel: [w1950 w1986] -> w1944
                        tunnel: [w1949 w1985] -> w1943
                        tunnel: [w1948 w1984] -> w1942
                        tunnel: [w1947 w1983] -> w1941
                        tunnel: w1940 -> [w1950 w1982]
                        tunnel: w1939 -> [w1949 w1981]
                        tunnel: w1938 -> [w1948 w1980]
                        tunnel: w1937 -> [w1947 w1979]
                        frame False {
                          n1209 = local read "PicoHarp ON"() -> (w1946:bool)
                          n1210 = case shown="True" w1946 {
                            tunnel: [w1951 w1953] -> w1945
                            frame False {
                              n1211 = Random Number (0-1)() -> (number: 0 to 1=w1951:dbl)
                            }
                            frame True {
                              n1212 = local read "PicoHarp handle"() -> (w1952:i32)
                              n1213 = local read "Signal source selection"() -> (w1954:T1)
                              n1214 = case shown="\"Signal PicoHarp count rate\"" w1954 {
                                tunnel: [w1955 w1956 w1961 w1969] -> w1953
                                tunnel: w1952 -> [_ _ w1960 w1970]
                                frame "Signal None", Default {
                                n1215 = Random Number (0-1)() -> (number: 0 to 1=w1955:dbl)
                                }
                                frame "Signal Stream" {
                                n1216 = Random Number (0-1)() -> (number: 0 to 1=w1956:dbl)
                                }
                                frame "Signal PicoHarp histro" {
                                n1217 = local read "Histo Time (s)"() -> (w1959:dbl)
                                n1218 = Multiply(x=w1959, y=1000) -> (x*y=w1958:dbl)
                                n1219 = To Long Integer(number=w1958) -> (32bit integer=w1957:i32)
                                n1220 = call "Start Measurement.vi"("Acquisition time"=w1957, "DeviceIndex"=w1960) -> ("DataValid"=w1963:bool)
                                n1221 = case shown="True" w1963 {
                                tunnel: [u32 0 w1966] -> w1961
                                tunnel: w1960 -> [_ w1965]
                                frame False {
                                }
                                frame True {
                                n1222 = call "Get Histogram.vi"("DeviceIndex"=w1965) -> ("IntegralCount"=w1966:i32)  [unwired: 1 in, 2 out]
                                }
                                }
                                }
                                frame "Signal PicoHarp count rate" {
                                n1223 = dll-call lib="F:/Users/Yuriy/Labview/JKU/StreamEye/StreamEye_master_v2_comp2015/PicoHarpLibrary/PHLib.dll" fn="PH_GetCountRate"("devidx"=w1970, "channel"=1, "rate"=0) -> ("rate"=w1969:i32)  [unwired: 6 in, 2 out]
                                }
                              }
                            }
                          }
                          n1224 = local write "Current Intensity"(w1945) -> ()
                          n1225 = local write "Time Trace"(w1945) -> ()
                        }
                        frame True {
                          n1226 = property on="Spectrum Graph" class="XYGraph (strict)"() -> ("CrsrList"=w1973:T11)  [unwired: 2 in, 2 out]
                          n1227 = control-ref of="Spectrum Graph"() -> (w1976:refnum<vi>)
                          n1228 = control-ref of="time elapsed"() -> (w1974:refnum<vi>)
                          n1229 = control-ref of="Time Trace"() -> (w1978:refnum<vi>)
                          n1230 = control-ref of="single spectrum?"() -> (w1975:refnum<vi>)
                          n1231 = control-ref of="Current Intensity"() -> (w1977:refnum<vi>)
                          n1232 = local read "Intensity mode selection"() -> (w1972:T2)
                          n1233 = for {
                            tunnel: w1973 -> [w1989] mode=indexing
                            tunnel: [w1987] -> w1971 mode=indexing
                            n1234 = Unbundle(w1989) -> ("Position"=w1988:cluster{"X":dbl, "Y":dbl})  [unwired: 15 out]
                            n1235 = Unbundle(w1988) -> ("X"=w1987:dbl)  [unwired: 1 out]
                          }
                          n1236 = call "subVI_get spectrum_master_v1.vi"("writer IN"=w1982, "error writer IN"=w1981, "reader IN"=w1980, "error reader IN"=w1979, "time trace IN"=w1978, "intensity integral IN"=w1977, "Stop IN"=w1975, "reference XY graph IN"=w1976, "Intensity mode selection"=w1972, "reference time elapsed IN"=w1974, "cursors positions"=w1971) -> ("writer OUT"=w1986:refnum<k21>, "error writer OUT"=w1985:errorcluster, "reader OUT"=w1984:refnum<k21>, "error reader OUT"=w1983:errorcluster)  [unwired: 5 in]
                        }
                      }
                    }
                  }
                  n1237 = local read "Stop Measurement"() -> (w1894:bool)
                }
                n1238 = flat-sequence {
                  tunnel: w1888 -> [w1994]
                  tunnel: w1885 -> [w1993]
                  tunnel: w1886 -> [w1992]
                  tunnel: w1887 -> [w1991]
                  frame #0 {
                    n1239 = local write "writer endpoint"(w1994) -> ()
                    n1240 = local write "error writer"(w1993) -> ()
                    n1241 = local write "reader endpoint"(w1992) -> ()
                    n1242 = local write "error reader"(w1991) -> ()
                    n1243 = local write "Stop Measurement"(FALSE ("Stop Cursor")) -> ()
                  }
                }
              }
              frame 18 {
              }
              frame 20 {
                n1244 = flat-sequence {
                  frame #0 {
                    n1245 = local write "busy"(TRUE ("busy")) -> ()
                  }
                  frame #1 {
                    w1998 = 0.5
                    w2009 = u16 65535 ("Number of Positions")
                    n1246 = local read "Res. (ps)"() -> (w2007:i32)
                    n1247 = Initialize Array "Initialize Array"(u32 0, 65536) -> (w2002:u32[])
                    n1248 = Multiply(x=w1998, y=1000) -> (x*y=w2013:dbl)
                    n1249 = local read "PicoHarp handle"() -> (w2011:i32)
                    n1250 = local read "Test Comp histo"() -> (w1996:bool)
                    n1251 = local read "Histo Time (s)"() -> (w1999:dbl)
                    n1252 = Divide(x=w2007, y=1000) -> (x/y=w2005:dbl)
                    n1253 = Divide(x=w1999, y=w1998) -> (x/y=w2001:dbl)
                    n1254 = Multiply(x=w2005, y=w2009) -> (x*y=w2008:dbl)
                    n1255 = To Long Integer(number=w2001) -> (32bit integer=w2000:i32)
                    n1256 = To Long Integer(number=w2013) -> (32bit integer=w2012:i32)
                    n1257 = call "subVI_RampGenerator.vi"("Number of Positions"=w2009, "End  (um)"=w2008, "Start  (um)"=0.0) -> ("Array"=w1997:dbl[])  [unwired: 1 in]
                    n1258 = case shown="False" w1996 {
                      tunnel: w2012 -> [w2019 w2039]
                      tunnel: w2011 -> [w2018 _]
                      tunnel: w2002 -> [w2017 _]
                      tunnel: w2000 -> [w2016 w2040]
                      tunnel: w1997 -> [w2015 _]
                      frame False {
                        n1259 = for {
                          N: w2016 -> [_]
                          tunnel: w2019 -> [w2030]
                          tunnel: w2018 -> [w2022]
                          shift-right: [w2025] -> _
                          shift-left: w2017 -> [w2029]
                          tunnel: w2015 -> [w2027]
                          stop <- w2024 stop-if-true
                          n1260 = call "Start Measurement.vi"("Acquisition time"=w2030, "DeviceIndex"=w2022) -> ("DataValid"=w2031:bool)
                          n1261 = case shown="True" w2031 {
                            tunnel: [u32 0 w2038] -> w2028
                            tunnel: w2022 -> [_ w2037]
                            tunnel: [w2032 w2034] -> w2025
                            tunnel: w2029 -> [w2032 w2036]
                            frame False {
                            }
                            frame True {
                              n1262 = call "Get Histogram.vi"("DeviceIndex"=w2037) -> ("Histogram"=w2035:u32[], "IntegralCount"=w2038:i32)  [unwired: 1 in, 1 out]
                              n1263 = Add(x=w2036, y=w2035) -> (x+y=w2034:u32[])
                            }
                          }
                          n1264 = dll-call lib="F:/Users/Yuriy/Labview/JKU/StreamEye/StreamEye_master_v2_comp2015/PicoHarpLibrary/PHLib.dll" fn="PH_GetCountRate"("devidx"=w2022, "channel"=1, "rate"=0) -> ("rate"=w2020:i32)  [unwired: 6 in, 2 out]
                          n1265 = local read "Stop Measurement"() -> (w2024:bool)
                          n1266 = local write "Time Trace"(w2020) -> ()
                          n1267 = local write "Current Intensity"(w2028) -> ()
                          n1268 = Bundle("Array"=w2027, w2025) -> (w2026:cluster{"Array":dbl[], u32[]})  [unwired: 1 in]
                          n1269 = local write "Histo Graph"(w2026) -> ()
                        }
                      }
                      frame True {
                        n1270 = for {
                          N: w2040 -> [_]
                          tunnel: w2039 -> [w2041]
                          stop <- w2042 stop-if-true
                          n1271 = flat-sequence {
                            tunnel: w2041 -> [w2056]
                            frame #0 {
                              n1272 = local read "Wait Scan."() -> (w2049:bool)
                              n1273 = global read "glb_pos.vi" "Position"() -> (w2055:dbl[])
                              n1274 = Index Array(array=w2055, index #1=0 ("index"), index #2=1 ("index")) -> (element #1=w2052:dbl, element #2=w2051:dbl)
                              n1275 = Subtract(x=w2052, y=0.0002) -> (x-y=w2053:dbl)
                              n1276 = Subtract(x=w2051, y=0.0002) -> (x-y=w2054:dbl)
                              n1277 = Build Array(w2052, w2051) -> (w2048:dbl[])
                              n1278 = Build Array(w2053, w2054) -> (w2050:dbl[])
                              n1279 = call "SMC_MoveAbs.vi"("WaitUntilReady"=w2049, "Input Array"=w2050) -> ("error out"=w2043:errorcluster)  [unwired: 9 in]
                              n1280 = call "SMC_MoveAbs.vi"("error in (no error)"=w2043, "WaitUntilReady"=w2049, "Input Array"=w2048) -> ()  [unwired: 8 in, 1 out]
                            }
                            frame #1 {
                              n1281 = Wait (ms)(milliseconds to wait=w2056) -> ()  [unwired: 1 out]
                            }
                          }
                          n1282 = local read "Stop Measurement"() -> (w2042:bool)
                        }
                      }
                    }
                  }
                  frame #2 {
                    n1283 = local write "Stop Measurement"(FALSE ("Stop Measurement")) -> ()
                    n1284 = local write "busy"(FALSE ("busy")) -> ()
                  }
                }
              }
              frame 21 {
                # "Y values (abs)"
                # "X values (abs)"
                # "Start Cursors Pair XY"
                n1285 = flat-sequence {
                  tunnel: w2078 -> [w2100]
                  tunnel: w2079 -> [w2099]
                  tunnel: w2061 -> [w2098]
                  tunnel: w2062 -> [w2097]
                  frame #0 {
                    n1286 = local write "busy"(TRUE ("busy")) -> ()
                    n1287 = local read "Wscale Sca"() -> (w2087:dbl[])
                    n1288 = local write "Wscale hyper"(w2087) -> ()
                    n1289 = Index Array(array=w2087, index=0) -> (element=w2091:dbl)
                    n1290 = Index Array(array=w2087, index=1) -> (element=w2092:dbl)
                    n1291 = Subtract(x=w2092, y=w2091) -> (x-y=w2093:dbl)
                    n1292 = property on="XYZ hyperspectral graph" class="IntGraph (strict)"("XScale.Offset"=w2091, "XScale.Multiplier"=w2093, "XScale.Precision"=u8 2 ("X Scale.Display Format:Precision")) -> ()  [unwired: 2 in, 2 out]
                  }
                  frame #1 {
                    n1293 = for {
                      N: w2100 -> [_]
                      shift-right: [w2110] -> w2095
                      shift-left: w2099 -> [w2109]
                      tunnel: w2098 -> [w2105] mode=indexing
                      tunnel: w2097 -> [w2103] mode=indexing
                      i -> [w2101]
                      n1294 = local read "Xscale Sca"() -> (w2106:dbl[])
                      n1295 = local read "Yscale Sca"() -> (w2104:dbl[])
                      n1296 = local read "XYZ MegaArray Sca"() -> (w2111:i32[][][])
                      n1297 = call "subVI_GetNearestElement.vi"("element value"=w2105, "input array"=w2106) -> ("index"=w2107:u32)  [unwired: 9 in]
                      n1298 = call "subVI_GetNearestElement.vi"("element value"=w2103, "input array"=w2104) -> ("index"=w2102:u32)  [unwired: 9 in]
                      n1299 = Index Array(array=w2111, index (dim 0)=w2107, index (dim 1)=w2102) -> (element=w2108:i32[])  [unwired: 1 in]
                      n1300 = Replace Array Subset(array=w2109, new element=w2108, index (row)=w2101) -> (w2110:i32[][])  [unwired: 1 in]
                    }
                    n1301 = local write "XW MegaArray"(w2095) -> ()
                    n1302 = Transpose 2D Array(2D array=w2095) -> (transposed array=w2096:i32[][])
                    n1303 = local write "XYZ hyperspectral graph"(w2096) -> ()
                  }
                  frame #2 {
                    n1304 = local write "busy"(FALSE ("busy")) -> ()
                    n1305 = local write "Stop Measurement"(FALSE ("Stop Cursor")) -> ()
                    n1306 = local write "Data available XW"(TRUE ("Data available XW")) -> ()
                  }
                }
                n1307 = local read "Xoffset_Sca"() -> (w2068:dbl)
                n1308 = local read "Yoffset_Sca"() -> (w2065:dbl)
                n1309 = local read "numPixels"() -> (w2059:u16)
                n1310 = property on="XYZ hyperspectral graph" class="IntGraph (strict)"("YScale.Offset"=0.0 ("Y Scale.Offset and Multiplier:Offset"), "YScale.Multiplier"=1.0 ("Y Scale.Offset and Multiplier:Multiplier"), "YScale.Precision"=u8 0 ("X Scale.Display Format:Precision")) -> ()  [unwired: 2 in, 2 out]
                n1311 = property on="XYZ Graph Scanner" class="IntGraph (strict)"() -> ("CrsrLis"=w2077:T11)  [unwired: 2 in, 2 out]
                n1312 = local read "Steps Hyperspectral Sca"() -> (w2078:u32)
                n1313 = for {
                  tunnel: w2077 -> [w2086] mode=indexing
                  tunnel: [w2084] -> w2067 mode=indexing
                  tunnel: [w2083] -> w2064 mode=indexing
                  n1314 = Unbundle(w2086) -> ("Position"=w2085:cluster{"X":dbl, "Y":dbl})  [unwired: 15 out]
                  n1315 = Unbundle(w2085) -> ("X"=w2084:dbl, "Y"=w2083:dbl)
                }
                n1316 = Add(x=w2068, y=w2067) -> (x+y=w2066:dbl[])
                n1317 = Add(x=w2064, y=w2065) -> (x+y=w2063:dbl[])
                n1318 = Index Array(array=w2066, index=0) -> (element=w2072:dbl)
                n1319 = Index Array(array=w2066, index=1) -> (element=w2071:dbl)
                n1320 = Index Array(array=w2063, index=0) -> (element=w2070:dbl)
                n1321 = Index Array(array=w2063, index=1) -> (element=w2069:dbl)
                n1322 = call "subVI_RampGenerator.vi"("Number of Positions"=w2078, "End  (um)"=w2069, "Start  (um)"=w2070) -> ("Array"=w2062:dbl[])  [unwired: 1 in]
                n1323 = call "subVI_RampGenerator.vi"("Number of Positions"=w2078, "End  (um)"=w2071, "Start  (um)"=w2072) -> ("Array"=w2061:dbl[])  [unwired: 1 in]
                n1324 = local write "Xscale hyper"(w2061) -> ()
                n1325 = Initialize Array(0, w2078, w2059) -> (w2079:i32[][])
              }
              frame 22 {
                n1326 = flat-sequence {
                  tunnel: [w2134] -> w2121
                  tunnel: [w2133] -> w2120
                  tunnel: [w2127] -> w2119
                  tunnel: [w2128] -> w2118
                  tunnel: [w2122] -> w2117
                  tunnel: w2121 -> [w2146]
                  tunnel: w2120 -> [w2145]
                  tunnel: w2119 -> [w2144]
                  tunnel: w2118 -> [w2140]
                  tunnel: w2117 -> [w2143]
                  tunnel: [w2137] -> w2116
                  tunnel: [w2136] -> w2115
                  tunnel: w2116 -> [w2401]
                  tunnel: w2115 -> [w2400]
                  frame #0 {
                    w2127 = 0 ("T2 Photon Count")
                    n1327 = local write "FiFo Overrun"(FALSE ("FiFo Overrun")) -> ()
                    n1328 = local write "busy"(TRUE ("busy")) -> ()
                    n1329 = local read "Filaname"() -> (w2124:string)
                    n1330 = local write "T2 Photon Count"(w2127) -> ()
                    n1331 = local read "PicoHarp handle"() -> (w2133:i32)
                    n1332 = local read "T2 Segments"() -> (w2134:u32)
                    n1333 = Concatenate Strings(w2124, "_T2_txyi.dat") -> (w2125:string)
                    n1334 = Concatenate Strings(w2124, "_T2.PTC") -> (w2130:string)
                    n1335 = local read "Path"() -> (w2126:path)
                    n1336 = local read "Path"() -> (w2131:path)
                    n1337 = Build Path(base path=w2126, name or relative path=w2125) -> (appended path=w2122:path)
                    n1338 = Build Path(base path=w2131, name or relative path=w2130) -> (appended path=w2128:path)
                    n1339 = Tick Count (ms)() -> ()  [unwired: 1 out]
                  }
                  frame #1 {
                    n1340 = Open/Create/Replace File(file path (use dialog)=w2140, operation (0:open)=T6."replace or create", access (0:read/write)=enum16{"read/write", "read-only", "write-only"}."write-only") -> (refnum out=w2141:refnum<file>, error out=w2142:errorcluster)  [unwired: 3 in, 1 out]
                    n1341 = for {
                      N: w2146 -> [_]
                      tunnel: w2145 -> [w2156]
                      shift-right: [w2153] -> _
                      shift-left: w2144 -> [w2155]
                      tunnel: w2143 -> [w2152]
                      tunnel: w2142 -> [w2150]
                      tunnel: w2141 -> [w2149]
                      tunnel: [w2148] -> w2137
                      tunnel: [w2147] -> w2136
                      stop <- w2154 stop-if-true
                      n1342 = flat-sequence {
                        tunnel: w2156 -> [w2171]
                        tunnel: w2155 -> [w2172]
                        tunnel: [w2160] -> w2154
                        tunnel: [w2170] -> w2153
                        tunnel: [w2160] -> w2151
                        tunnel: w2150 -> [w2159]
                        tunnel: w2149 -> [w2157]
                        tunnel: [w2158] -> w2148
                        tunnel: [w2157] -> w2147
                        tunnel: w2152 -> [w2226]
                        tunnel: w2151 -> [w2225]
                        frame #0 {
                          n1343 = local read "T2 Block Size"() -> (w2169:u16)
                          n1344 = local read "Drift Compensate Time"() -> (w2162:i32)
                          n1345 = case shown="0, Default" w2169 {
                            tunnel: [i16 15 ("n") i16 9 ("n") i16 12 ("n") i16 15 ("n") i16 16 ("n") i16 17 ("n")] -> w2168
                            frame 0, Default {
                            }
                            frame 1 {
                            }
                            frame 2 {
                            }
                            frame 3 {
                            }
                            frame 4 {
                            }
                            frame 5 {
                            }
                          }
                          n1346 = Multiply(x=1000, y=w2162) -> (x*y=w2161:i32)
                          n1347 = dll-call lib="F:/Users/Yuriy/Labview/JKU/StreamEye/StreamEye_master_v2_comp2015/PicoHarpLibrary/phlib.dll" fn="PH_StartMeas"("devidx"=w2171, "tacq"=w2161) -> (w2174:i32)  [unwired: 5 in, 2 out]
                          n1348 = Scale By Power Of 2(n=w2168, x=1.0) -> (x*2^n=w2166:dbl)
                          n1349 = Equal To 0?(x=w2174) -> (x = 0?=w2173:bool)
                          n1350 = To Long Integer(number=w2166) -> (32bit integer=w2165:i32)
                          n1351 = Initialize Array(u32 0 ("element"), 262144) -> (w2175:u32[])
                          n1352 = case shown="True" w2173 {
                            selector: w2173 -> [w2187 w2198]
                            tunnel: [w2187 w2197] -> w2177
                            tunnel: w2172 -> [w2184 w2196]
                            tunnel: w2157 -> [_ w2195]
                            tunnel: w2159 -> [w2186 w2194]
                            tunnel: [w2186 w2193] -> w2158
                            tunnel: w2175 -> [_ w2192]
                            tunnel: w2171 -> [_ w2191]
                            tunnel: [w2185 w2188] -> w2160
                            tunnel: [w2184 w2190] -> w2170
                            tunnel: w2165 -> [_ w2189]
                            frame False {
                              n1353 = local read "Stop Measurement"() -> (w2185:bool)
                            }
                            frame True {
                              n1354 = while {
                                tunnel: w2191 -> [w2199]
                                tunnel: w2192 -> [w2201]
                                tunnel: [w2206] -> w2193
                                tunnel: w2194 -> [w2203]
                                tunnel: w2195 -> [w2200]
                                shift-left: w2196 -> [w2208]
                                shift-right: [w2216] -> w2190
                                tunnel: [w2223] -> w2197
                                tunnel: w2198 -> [w2223]
                                tunnel: [w2214] -> w2188
                                tunnel: w2189 -> [w2202]
                                stop <- w2211 continue-if-true
                                n1355 = call "TTTR.vi"("block size"=w2202, "error in (no error)"=w2203, "file refnum"=w2200, "Array"=w2201, "DeviceIndex"=w2199) -> ("count"=w2207:i32, "error out"=w2206:errorcluster, "FiFoOverrun"=w2205:bool, "OK"=w2204:bool)  [unwired: 1 in]
                                n1356 = local read "Stop Measurement"() -> (w2214:bool)
                                n1357 = dll-call lib="F:/Users/Yuriy/Labview/JKU/StreamEye/StreamEye_master_v2_comp2015/PicoHarpLibrary/PHLib.dll" fn="PH_GetCountRate"("devidx"=w2199, "channel"=0, "rate"=0) -> ("rate"=w2210:i32)  [unwired: 6 in, 2 out]
                                n1358 = dll-call lib="F:/Users/Yuriy/Labview/JKU/StreamEye/StreamEye_master_v2_comp2015/PicoHarpLibrary/PHLib.dll" fn="PH_GetCountRate"("devidx"=w2199, "channel"=1, "rate"=0) -> ("rate"=w2209:i32)  [unwired: 6 in, 2 out]
                                n1359 = local write "FiFo Overrun"(w2205) -> ()
                                n1360 = Unbundle(w2206) -> ("status"=w2221:bool)  [unwired: 2 out]
                                n1361 = Add(x=w2207, y=w2208) -> (x+y=w2216:i32)
                                n1362 = local write "T2 Photon Count"(w2216) -> ()
                                n1363 = Not(x=w2221) -> (.not. x?=w2222:bool)
                                n1364 = global write "Global.vi" "GlobalRate0"(w2210) -> ()
                                n1365 = local write "Ch0 Rate"(w2210) -> ()
                                n1366 = global write "Global.vi" "GlobalRate1"(w2209) -> ()
                                n1367 = local write "Ch1 Rate"(w2209) -> ()
                                n1368 = And(x=w2204, y=w2222) -> (x .and. y?=w2213:bool)
                                n1369 = Add(x=w2210, y=w2209) -> (x+y=w2215:i32)
                                n1370 = Not(x=w2214) -> (.not. x?=w2212:bool)
                                n1371 = local write "Current Intensity"(w2215) -> ()
                                n1372 = local write "Time Trace"(w2215) -> ()
                                n1373 = And(x=w2213, y=w2212) -> (x .and. y?=w2211:bool)
                              }
                            }
                          }
                          n1374 = case shown="True" w2177 {
                            tunnel: w2171 -> [_ w2224]
                            frame False {
                            }
                            frame True {
                              n1375 = dll-call lib="F:/Users/Yuriy/Labview/JKU/StreamEye/StreamEye_master_v2_comp2015/PicoHarpLibrary/phlib.dll" fn="PH_StopMeas"("devidx"=w2224) -> ()  [unwired: 5 in, 2 out]
                            }
                          }
                        }
                        frame #1 {
                          n1376 = case shown="False" w2225 {
                            tunnel: w2226 -> [w2227 _]
                            frame False {
                              n1377 = local read "Current Intensity"() -> (w2228:dbl)
                              n1378 = for {
                                N: 2 -> [_]
                                shift-right: [w2232] -> _
                                shift-left: w2228 -> [w2233]
                                tunnel: w2227 -> [w2230]
                                i -> [w2234]
                                n1379 = for {
                                N: 2 -> [_]
                                tunnel: w2234 -> [w2241]
                                shift-right: [w2240] -> w2232
                                shift-left: w2233 -> [w2242]
                                shift-right: [w2237] -> _
                                shift-left: FALSE -> [w2239]
                                tunnel: w2230 -> [w2236]
                                i -> [w2238]
                                n1380 = case shown="False" w2239 {
                                selector: w2239 -> [_ w2398]
                                tunnel: w2242 -> [w2245 w2399]
                                tunnel: w2241 -> [w2249 _]
                                tunnel: [w2243 w2399] -> w2240
                                tunnel: w2238 -> [w2248 _]
                                tunnel: [w2246 w2398] -> w2237
                                tunnel: w2236 -> [w2244 _]
                                frame False {
                                n1381 = while {
                                tunnel: w2249 -> [w2269]
                                tunnel: w2248 -> [w2268]
                                tunnel: [w2264] -> w2247
                                tunnel: w2244 -> [w2254]
                                shift-right: [w2250] -> w2243
                                shift-left: w2245 -> [w2260]
                                i -> [w2264]
                                stop <- w2259 stop-if-true
                                n1382 = flat-sequence {
                                tunnel: w2269 -> [w2342]
                                tunnel: w2268 -> [w2338]
                                tunnel: [w2337] -> w2257
                                tunnel: [w2336] -> w2256
                                tunnel: [w2349] -> w2253
                                tunnel: [w2348] -> w2252
                                tunnel: w2261 -> [w2379]
                                tunnel: w2260 -> [w2376]
                                tunnel: [w2375] -> w2259
                                tunnel: [w2370] -> w2255
                                tunnel: [w2374] -> w2258
                                tunnel: w2254 -> [w2368]
                                tunnel: w2253 -> [w2372]
                                tunnel: w2252 -> [w2371]
                                tunnel: [w2368] -> w2251
                                frame #0 {
                                n1383 = case shown="1" w2338 {
                                tunnel: [1 -1] -> w2336
                                frame 0, Default {
                                }
                                frame 1 {
                                }
                                }
                                n1384 = local read "Wait Scan."() -> (w2343:bool)
                                n1385 = local read "Drift Comp Step"() -> (w2340:dbl)
                                n1386 = Multiply(x=w2340, y=w2336) -> (x*y=w2339:dbl)
                                n1387 = Divide(x=w2339, y=1000.0) -> (x/y=w2344:dbl)
                                n1388 = Increment(x=w2342) -> (x+1=w2337:i32)
                                n1389 = call "SMC_AxisRel.vi"("WaitUntilReady"=w2343, "Distance"=w2344, "AxisNr"=w2337) -> ()  [unwired: 8 in, 1 out]
                                }
                                frame #1 {
                                n1390 = Wait (ms)(milliseconds to wait=u32 100) -> ()  [unwired: 1 out]
                                }
                                frame #2 {
                                # "read"
                                n1391 = local read "Xoffset_Sca"() -> (w2358:dbl)
                                n1392 = local read "Yoffset_Sca"() -> (w2356:dbl)
                                n1393 = global read "glb_pos.vi" "Position"() -> (w2360:dbl[])
                                n1394 = Index Array(array=w2360, index #1=0 ("index"), index #2=1 ("index")) -> (element #1=w2357:dbl, element #2=w2354:dbl)
                                n1395 = Multiply(x=w2357, y=1000.0) -> (x*y=w2359:dbl)
                                n1396 = Multiply(x=w2354, y=1000.0) -> (x*y=w2355:dbl)
                                n1397 = Subtract(x=w2359, y=w2358) -> (x-y=w2349:dbl)
                                n1398 = Subtract(x=w2355, y=w2356) -> (x-y=w2348:dbl)
                                n1399 = local write "Xread_Sca"(w2349) -> ()
                                n1400 = local write "Yread_Sca"(w2348) -> ()
                                }
                                frame #3 {
                                n1401 = Tick Count (ms)() -> (millisecond timer value=w2366:u32)
                                n1402 = local read "Compensate Int Time"() -> (w2363:dbl)
                                n1403 = Divide(x=w2366, y=u32 1000) -> (x/y=w2364:dbl)
                                n1404 = Multiply(x=w2363, y=10.0) -> (x*y=w2361:dbl)
                                n1405 = for {
                                N: w2361 -> [_]
                                tunnel: [w2385] -> w2378 mode=indexing
                                tunnel: [w2384] -> w2377 mode=indexing
                                n1406 = while {
                                tunnel: [w2389] -> w2385
                                tunnel: [w2390] -> w2384
                                stop <- w2391 stop-if-true
                                w2388 = 0 ("y")
                                n1407 = Wait (ms)(milliseconds to wait=u32 100) -> ()  [unwired: 1 out]
                                n1408 = local read "PicoHarp handle"() -> (w2393:i32)
                                n1409 = dll-call lib="F:/Users/Yuriy/Labview/JKU/StreamEye/StreamEye_master_v2_comp2015/PicoHarpLibrary/PHLib.dll" fn="PH_GetCountRate"("devidx"=w2393, "channel"=0, "rate"=0) -> ("rate"=w2390:i32)  [unwired: 6 in, 2 out]
                                n1410 = dll-call lib="F:/Users/Yuriy/Labview/JKU/StreamEye/StreamEye_master_v2_comp2015/PicoHarpLibrary/PHLib.dll" fn="PH_GetCountRate"("devidx"=w2393, "channel"=1, "rate"=0) -> ("rate"=w2389:i32)  [unwired: 6 in, 2 out]
                                n1411 = Greater?(x=w2390, y=w2388) -> (0:w2387:bool)
                                n1412 = Greater?(x=w2389, y=w2388) -> (0:w2386:bool)
                                n1413 = And(x=w2387, y=w2386) -> (x .and. y?=w2391:bool)
                                }
                                }
                                n1414 = Add Array Elements(numeric array=w2377) -> (sum=w2380:i32)
                                n1415 = Add Array Elements(numeric array=w2378) -> (sum=w2382:i32)
                                n1416 = Divide(x=w2380, y=w2361) -> (x/y=w2381:dbl)
                                n1417 = Divide(x=w2382, y=w2361) -> (x/y=w2383:dbl)
                                n1418 = local write "Ch0 Rate"(w2381) -> ()
                                n1419 = local write "Ch1 Rate"(w2383) -> ()
                                n1420 = Add(x=w2381, y=w2383) -> (x+y=w2370:dbl)
                                n1421 = Less?(x=w2370, y=w2376) -> (x < y?=w2374:bool)
                                n1422 = Build Array(w2364, w2372, w2371, w2370) -> (w2369:dbl[])
                                n1423 = local write "Current Intensity"(w2370) -> ()
                                n1424 = local write "Time Trace"(w2370) -> ()
                                n1425 = Or(x=w2374, y=w2379) -> (x .or. y?=w2375:bool)
                                n1426 = call-poly <vilib>:"Write Delimited Spreadsheet.vi"("file path (dialog if empty)"=w2368, "1D data"=w2369, "append to file? (new file:F)"=TRUE ("transpose? (no:F)"), "transpose? (no:F)"=FALSE) -> ()  [unwired: 10 in, 2 out]
                                }
                                }
                                n1427 = local read "Drift Comp Range"() -> (w2267:dbl)
                                n1428 = local read "Drift Comp Step"() -> (w2266:dbl)
                                n1429 = Divide(x=w2267, y=w2266) -> (x/y=w2265:dbl)
                                n1430 = Increment(x=w2264) -> (x+1=w2263:i32)
                                n1431 = Round To Nearest(number=w2265) -> (nearest integer value=w2262:dbl)
                                n1432 = Greater Or Equal?(x=w2263, y=w2262) -> (x >= y?=w2261:bool)
                                n1433 = case shown="True" w2258 {
                                tunnel: w2257 -> [_ w2276]
                                tunnel: w2256 -> [_ w2275]
                                tunnel: w2255 -> [w2270 _]
                                tunnel: [w2270 w2274] -> w2250
                                tunnel: w2251 -> [_ w2271]
                                frame False {
                                }
                                frame True {
                                n1434 = flat-sequence {
                                tunnel: w2276 -> [w2282]
                                tunnel: w2275 -> [w2280]
                                tunnel: [w2290] -> w2273
                                tunnel: [w2289] -> w2272
                                tunnel: [w2321] -> w2274
                                tunnel: w2273 -> [w2319]
                                tunnel: w2272 -> [w2318]
                                tunnel: w2271 -> [w2315]
                                frame #0 {
                                n1435 = local read "Wait Scan."() -> (w2281:bool)
                                n1436 = local read "Drift Comp Step"() -> (w2279:dbl)
                                n1437 = local read "Drift Comp BackStep"() -> (w2277:dbl)
                                n1438 = Multiply(x=w2280, y=-1.0) -> (x*y=w2283:dbl)
                                n1439 = Add(x=w2279, y=w2277) -> (x+y=w2278:dbl)
                                n1440 = Multiply(x=w2278, y=w2283) -> (x*y=w2286:dbl)
                                n1441 = Divide(x=w2286, y=1000.0) -> (x/y=w2287:dbl)
                                n1442 = call "SMC_AxisRel.vi"("WaitUntilReady"=w2281, "Distance"=w2287, "AxisNr"=w2282) -> ()  [unwired: 8 in, 1 out]
                                }
                                frame #1 {
                                n1443 = Wait (ms)(milliseconds to wait=u32 100) -> ()  [unwired: 1 out]
                                }
                                frame #2 {
                                # "read"
                                n1444 = local read "Xoffset_Sca"() -> (w2293:dbl)
                                n1445 = local read "Yoffset_Sca"() -> (w2295:dbl)
                                n1446 = global read "glb_pos.vi" "Position"() -> (w2291:dbl[])
                                n1447 = Index Array(array=w2291, index #1=0 ("index"), index #2=1 ("index")) -> (element #1=w2294:dbl, element #2=w2297:dbl)
                                n1448 = Multiply(x=w2294, y=1000.0) -> (x*y=w2292:dbl)
                                n1449 = Multiply(x=w2297, y=1000.0) -> (x*y=w2296:dbl)
                                n1450 = Subtract(x=w2292, y=w2293) -> (x-y=w2290:dbl)
                                n1451 = Subtract(x=w2296, y=w2295) -> (x-y=w2289:dbl)
                                n1452 = local write "Xread_Sca"(w2290) -> ()
                                n1453 = local write "Yread_Sca"(w2289) -> ()
                                }
                                frame #3 {
                                n1454 = Tick Count (ms)() -> (millisecond timer value=w2313:u32)
                                n1455 = local read "Compensate Int Time"() -> (w2308:dbl)
                                n1456 = Divide(x=w2313, y=u32 1000) -> (x/y=w2311:dbl)
                                n1457 = Multiply(x=w2308, y=10.0) -> (x*y=w2310:dbl)
                                n1458 = for {
                                N: w2310 -> [_]
                                tunnel: [w2323] -> w2306 mode=indexing
                                tunnel: [w2322] -> w2307 mode=indexing
                                n1459 = while {
                                tunnel: [w2327] -> w2323
                                tunnel: [w2328] -> w2322
                                stop <- w2329 stop-if-true
                                w2326 = 0 ("y")
                                n1460 = local read "PicoHarp handle"() -> (w2331:i32)
                                n1461 = Wait (ms)(milliseconds to wait=u32 100) -> ()  [unwired: 1 out]
                                n1462 = dll-call lib="F:/Users/Yuriy/Labview/JKU/StreamEye/StreamEye_master_v2_comp2015/PicoHarpLibrary/PHLib.dll" fn="PH_GetCountRate"("devidx"=w2331, "channel"=0, "rate"=0) -> ("rate"=w2328:i32)  [unwired: 6 in, 2 out]
                                n1463 = dll-call lib="F:/Users/Yuriy/Labview/JKU/StreamEye/StreamEye_master_v2_comp2015/PicoHarpLibrary/PHLib.dll" fn="PH_GetCountRate"("devidx"=w2331, "channel"=1, "rate"=0) -> ("rate"=w2327:i32)  [unwired: 6 in, 2 out]
                                n1464 = Greater?(x=w2328, y=w2326) -> (0:w2324:bool)
                                n1465 = Greater?(x=w2327, y=w2326) -> (0:w2325:bool)
                                n1466 = And(x=w2324, y=w2325) -> (x .and. y?=w2329:bool)
                                }
                                }
                                n1467 = Add Array Elements(numeric array=w2307) -> (sum=w2305:i32)
                                n1468 = Add Array Elements(numeric array=w2306) -> (sum=w2304:i32)
                                n1469 = Divide(x=w2305, y=w2310) -> (x/y=w2303:dbl)
                                n1470 = Divide(x=w2304, y=w2310) -> (x/y=w2302:dbl)
                                n1471 = Add(x=w2303, y=w2302) -> (x+y=w2317:dbl)
                                n1472 = local write "Ch0 Rate"(w2303) -> ()
                                n1473 = local write "Ch1 Rate"(w2302) -> ()
                                n1474 = Build Array(w2311, w2319, w2318, w2317) -> (w2316:dbl[])
                                n1475 = local write "Current Intensity"(w2317) -> ()
                                n1476 = local write "Time Trace"(w2317) -> ()
                                n1477 = call-poly <vilib>:"Write Delimited Spreadsheet.vi"("file path (dialog if empty)"=w2315, "1D data"=w2316, "append to file? (new file:F)"=TRUE ("transpose? (no:F)"), "transpose? (no:F)"=FALSE) -> ()  [unwired: 10 in, 2 out]
                                n1478 = To Double Precision Float(number=w2317) -> (double precision float=w2321:dbl)
                                }
                                }
                                }
                                }
                                }
                                n1479 = Greater Than 0?(x=w2247) -> (x > 0?=w2246:bool)
                                }
                                frame True {
                                }
                                }
                                }
                              }
                            }
                            frame True {
                            }
                          }
                        }
                      }
                    }
                  }
                  frame #2 {
                    n1480 = Close File(refnum=w2400, error in=w2401) -> (error out=→"file error status":errorcluster)  [unwired: 1 out]
                    n1481 = local write "busy"(FALSE ("busy")) -> ()
                    n1482 = local write "Stop Measurement"(FALSE ("Stop Cursor")) -> ()
                  }
                }
              }
              frame 24 {
                n1483 = local read "error reader"() -> (w2409:errorcluster)
                n1484 = local read "error writer"() -> (w2411:errorcluster)
                n1485 = local read "reader endpoint"() -> (w2410:refnum<k21>)
                n1486 = local read "writer endpoint"() -> (w2412:refnum<k21>)
                n1487 = while {
                  tunnel: w2412 -> [w2430]
                  tunnel: w2411 -> [w2429]
                  tunnel: w2410 -> [w2428]
                  tunnel: w2409 -> [w2427]
                  tunnel: [w2426] -> w2408
                  tunnel: [w2425] -> w2407
                  tunnel: [w2424] -> w2406
                  tunnel: [w2423] -> w2405
                  stop <- w2421 stop-if-true
                  n1488 = local read "Stop Measurement"() -> (w2420:bool)
                  n1489 = flat-sequence {
                    tunnel: w2430 -> [w2436]
                    tunnel: w2429 -> [w2435]
                    tunnel: [w2434] -> w2424
                    tunnel: [w2433] -> w2423
                    tunnel: w2420 -> [w2432]
                    tunnel: [w2431] -> w2418
                    tunnel: [w2439] -> w2419
                    tunnel: w2418 -> [w2439]
                    tunnel: w2428 -> [w2454]
                    tunnel: w2427 -> [w2453]
                    tunnel: [w2452] -> w2426
                    tunnel: [w2451] -> w2425
                    tunnel: [w2448] -> w2422
                    tunnel: w2419 -> [w2441]
                    frame #0 {
                      # "ready to acquire"
                      n1490 = shared-variable-write(w2436, w2435, w2432) -> (w2438:refnum<k21>, w2437:errorcluster)  [unwired: 1 in, 1 out]
                      n1491 = Flush Stream(8:w2437, 11:w2438) -> (0:w2433:errorcluster, 3:w2434:refnum<k21>)  [unwired: 2 in, 1 out]
                      n1492 = Tick Count (ms)() -> (millisecond timer value=w2431:u32)
                    }
                    frame #1 {
                    }
                    frame #2 {
                      n1493 = shared-variable-read(w2454, w2453) -> (w2452:refnum<k21>, w2451:errorcluster, w2450:cluster{dbl[], dbl[]})  [unwired: 1 in, 1 out]
                      n1494 = Tick Count (ms)() -> (millisecond timer value=w2443:u32)
                      n1495 = Subtract(x=w2443, y=w2441) -> (x-y=w2444:u32)
                      n1496 = Unbundle(w2450) -> (w2447:dbl[])  [unwired: 1 out]
                      n1497 = Index Array(array=w2447, index=0) -> (element=w2445:dbl)
                      n1498 = Divide(x=w2444, y=u32 1000) -> (x/y=w2440:dbl)
                      n1499 = local write "time elapsed"(w2440) -> ()
                      n1500 = Equal?(x=w2445, y=0) -> (x = y?=w2448:bool)
                    }
                  }
                  n1501 = Or(x=w2422, y=w2420) -> (x .or. y?=w2421:bool)
                }
                n1502 = flat-sequence {
                  tunnel: w2408 -> [w2416]
                  tunnel: w2407 -> [w2415]
                  tunnel: w2406 -> [w2414]
                  tunnel: w2405 -> [w2413]
                  frame #0 {
                    n1503 = local write "reader endpoint"(w2416) -> ()
                    n1504 = local write "error reader"(w2415) -> ()
                    n1505 = local write "writer endpoint"(w2414) -> ()
                    n1506 = local write "error writer"(w2413) -> ()
                    n1507 = local write "Stop Measurement"(FALSE ("Stop Measurement")) -> ()
                  }
                }
              }
            }
          }
          frame #2 {
            # "fast updates"
            n1508 = local read "Scanner ON"() -> (w2484:bool)
            n1509 = local read "Ystart_Gal"() -> (w2476:dbl)
            n1510 = local read "Xstart_Gal"() -> (w2482:dbl)
            n1511 = local read "Ystart_Sca"() -> (w2470:dbl)
            n1512 = local read "Ystep_Sca"() -> (w2468:dbl)
            n1513 = local read "Xstart_Sca"() -> (w2473:dbl)
            n1514 = local read "Xstep_Sca"() -> (w2471:dbl)
            n1515 = local read "Ystep_Gal"() -> (w2474:dbl)
            n1516 = local read "Xstep_Gal"() -> (w2483:dbl)
            n1517 = local read "Yend_Sca"() -> (w2469:dbl)
            n1518 = local read "Xend_Sca"() -> (w2472:dbl)
            n1519 = local read "Yend_Gal"() -> (w2475:dbl)
            n1520 = local read "Xend_Gal"() -> (w2481:dbl)
            n1521 = local read "PicoHarp ON"() -> (w2455:bool)
            n1522 = Subtract(x=w2476, y=w2475) -> (x-y=w2479:dbl)
            n1523 = Subtract(x=w2482, y=w2481) -> (x-y=w2480:dbl)
            n1524 = Subtract(x=w2470, y=w2469) -> (x-y=w2477:dbl)
            n1525 = Subtract(x=w2473, y=w2472) -> (x-y=w2478:dbl)
            n1526 = case shown="True" w2484 {
              frame False {
              }
              frame True {
                # "mm to um"
                n1527 = local read "Xoffset_Sca"() -> (w2501:dbl)
                n1528 = local read "Yoffset_Sca"() -> (w2496:dbl)
                n1529 = global read "glb_pos.vi" "Position"() -> (w2492:dbl[])
                n1530 = Index Array(array=w2492, index #1=0 ("index"), index #2=1 ("index")) -> (element #1=w2498:dbl, element #2=w2493:dbl)
                n1531 = Multiply(x=w2493, y=1000.0) -> (x*y=w2495:dbl)
                n1532 = Subtract(x=w2495, y=w2496) -> (x-y=w2494:dbl)
                n1533 = Multiply(x=w2498, y=1000.0) -> (x*y=w2502:dbl)
                n1534 = local write "Yread_Sca"(w2494) -> ()
                n1535 = Subtract(x=w2502, y=w2501) -> (x-y=w2499:dbl)
                n1536 = local write "Xread_Sca"(w2499) -> ()
              }
            }
            n1537 = Quotient & Remainder(x=w2479, y=w2474) -> (floor(x/y)=w2461:dbl)  [unwired: 1 out]
            n1538 = Quotient & Remainder(x=w2480, y=w2483) -> (floor(x/y)=w2467:dbl)  [unwired: 1 out]
            n1539 = Quotient & Remainder(x=w2477, y=w2468) -> (floor(x/y)=w2456:dbl)  [unwired: 1 out]
            n1540 = Quotient & Remainder(x=w2478, y=w2471) -> (floor(x/y)=w2459:dbl)  [unwired: 1 out]
            n1541 = case shown="True" w2455 {
              frame False {
              }
              frame True {
                n1542 = local read "PicoHarp handle"() -> (w2487:i32)
                n1543 = dll-call lib="F:/Users/Yuriy/Labview/JKU/StreamEye/StreamEye_master_v2_comp2015/PicoHarpLibrary/PHLib.dll" fn="PH_GetCountRate"("devidx"=w2487, "channel"=1, "rate"=0) -> ("rate"=w2485:i32)  [unwired: 6 in, 2 out]
                n1544 = dll-call lib="F:/Users/Yuriy/Labview/JKU/StreamEye/StreamEye_master_v2_comp2015/PicoHarpLibrary/PHLib.dll" fn="PH_GetCountRate"("devidx"=w2487, "channel"=0, "rate"=0) -> ("rate"=w2486:i32)  [unwired: 6 in, 2 out]
                n1545 = local write "Ch1 Rate"(w2485) -> ()
                n1546 = local write "Ch0 Rate"(w2486) -> ()
              }
            }
            n1547 = Absolute Value(x=w2461) -> (abs(x)=w2464:dbl)
            n1548 = Absolute Value(x=w2467) -> (abs(x)=w2466:dbl)
            n1549 = Absolute Value(x=w2456) -> (abs(x)=w2462:dbl)
            n1550 = Absolute Value(x=w2459) -> (abs(x)=w2463:dbl)
            n1551 = Increment(x=w2464) -> (x+1=w2460:dbl)
            n1552 = Increment(x=w2466) -> (x+1=w2465:dbl)
            n1553 = Increment(x=w2462) -> (x+1=w2457:dbl)
            n1554 = Increment(x=w2463) -> (x+1=w2458:dbl)
            n1555 = local write "Ysteps_Gal"(w2460) -> ()
            n1556 = local write "Xsteps_Gal"(w2465) -> ()
            n1557 = local write "Ysteps_Sca"(w2457) -> ()
            n1558 = local write "Xsteps_Sca"(w2458) -> ()
          }
        }
      }
    }
  }
